vi "Text control 2 v7.2_pump-specific.vi"() -> ()   [LabVIEW 2019]
panel:
  in  "Tab Control":enum32{"Main", "Other parameters"}(tab)
  out "Vdg vs time (Bias Stress)":cluster{"Y data in":dbl[], "X data in":dbl[]}[](graph)
  out "Vp vs Vg (FPP)":cluster{"Y data in":dbl[], "X data in":dbl[]}[](graph)
  out "Vp vs time (FPP Bias Stress)":cluster{"Y data in":dbl[], "X data in":dbl[]}[](graph)
  out "Line running":i32
  out "Total lines":i32
  out "Path":path=path "C:/users/rlp38/09Apr2009LTtesting/test2.txt"
  out "I vs Vg":cluster{"Y data in":dbl[], "X data in":dbl[]}[](graph)
  out "Is max":dbl format="%.2e"
  out "Id max":dbl format="%.2e"
  out "Ig max":dbl format="%.2e"
  out "Imax vs time":cluster{"Y data in":dbl[], "X data in":dbl[]}[](graph)
  out "Imin vs time":cluster{"Y data in":dbl[], "X data in":dbl[]}[](graph)
  out "I vs Vd":cluster{"Y data in":dbl[], "X data in":dbl[]}[](graph)
  in  "Script":string="#-------------------------------------------------------\n# SPM pump cleaning script x 10\n#\n# Version: 0.5\n# Author: Dimitrios Simatos\n# Last updated: 2020-09-03\n#-------------------------------------------------------\n# Description\n#\n# This script is designed to run the cleaning sequence of the SPM OEM pump ten times.\n#-------------------------------------------------------\n# Changes\n#\n# Placed initialization and hard stop commands in the beginning.\n#-------------------------------------------------------\n# Important points\n#\n# Never leave any liquid in the pump to dry after the experiments. If they dry, the residue may block the valve.\n# Always run the cleaning cycle after the experiments.\n# Use clockwise rotation when going up in valve port numbers and vice versa.\n#-------------------------------------------------------\n# Things to do before running the script\n#\n# Remove all reservoirs, except the one in Port 3.\n# Set filenames.\n# Replace the tubing, if necessary.\n#-------------------------------------------------------\n# Port connections\n#\n# Port 1: Waste\n# Port 2: Waste\n# Port 3: Various cleaning liquids\n# Port 4: Waste\n# Port 5: Waste\n# Port 6: Waste\n#\n# Between each of the 4 runs, the settings of Port 3 will change, according to the cleaning protocol.\n# The settings for Port 3 are:\n# 1st run: 1% v/v solution of sodium hypochlorite in ultrapure water\n# 2nd run: 0.1% w/v solution of sodium dodecyl sulfate in ultrapure water\n# 3rd run: Ultrapure water\n# 4th run: Waste (in air, not immersed in liquid)\n#-------------------------------------------------------\n# Cleaning protocol for the SPM OEM pump (from the manual)\n#\n# A cleaning procedure should be performed at the end of each day or in between two different experiments.\n# An effective cleaning can be performed in the following manner:\n# • Bleach solution to kill microorganisms\n# 1. Prepare a solution of 1% chlorine bleach and deionized water\n#    NOTE: Prepare a 1% v/v solution of sodium hypochlorite in deionized water\n# 2. Prepare a reservoir and place 1 tubing in the bleach solution and 5 tubings in a waste recipient\n# 3. Pick up the bleach solution through 1 port to entirely fill the syringe\n# 4. Sequentially output the syringe content through the remaining ports and throw it to the waste\n# 5. Repeat operation at least 2 times\n# • Detergent solution to remove debris\n# 1. Prepare a solution of 0.1% detergent and deionized water\n#    NOTE: Prepare a 0.1% w/v solution of sodium dodecyl sulfate in deionized water\n# 2. Move the tubing from the bleach solution reservoir and place it into a reservoir of detergent solution\n# 3. Pick up the detergent solution through 1 port to entirely fill the syringe\n# 4. Sequentially output the detergent solution through the remaining ports into the waste recipient\n# 5. Repeat operation at least 2 times\n# • Rinsing water to prepare the pump for your next experiment\n# 1. Move the tubing from the detergent solution reservoir and place it into a reservoir of deionized water\n# 2. Pick up the rinsing solution through 1 port to entirely fill the syringe\n# 3. Sequentially output the rinse water through the remaining ports into the waste recipient\n# 4. Repeat operation at least 2 times\n# • Replace the tubing, if necessary\n#-------------------------------------------------------\n# Pumping cycles and execution time\n#\n# Execution time for a single cycle: 6 x (1 min + 10 sec) = 7 minutes\n# Total execution time: 4 x 7 = 28 minutes\n# Since the script has to run 4 times, the cleaning lasts for: 4 x 28 = 112 minutes\n# Air must be the last to be pumped through the valve, to remove all liquids.\n# There are 4 pumping cycles. Each one draws a different liquid through port 3 and pumps it sequentially through ports 1,2,4,5,6.\n# During the sequential pumping, each port receives 200 ul of liquid (20% of the total syringe volume = 600 \"plunger units\")\n# The device must be disconnected from the port during the cleaning procedure.\n# All cycles are similar, except cycle 1 has the initialization command uncommented and the first report valve command commented.\n#-------------------------------------------------------\n# Volume of liquid needed\n#\n# Volume of liquid needed per cycle: 1 ml\n# Total volume of liquid needed per script run: 4 x 1 = 4 ml\n# Since the script has to run 4 times, the first 3 with different liquids, I need:\n# 4 ml of 1% v/v solution of sodium hypochlorite in ultrapure water\n# 4 ml of 0.1% w/v solution of sodium dodecyl sulfate in ultrapure water\n# 4 ml of ultrapure water\n#-------------------------------------------------------\n# Parameters\n#\n# Syringe size: 1 ml\n# Step resolution N = 0.01 mm\n# Drawing flow V = 300 pulses/second (6000 ul/min)\n# Pumping flow V = 300 pulses/second (6000 ul/min)\n#-------------------------------------------------------\n# Pump initialization\npump /1T #hard stop pump\npump /1ZR #initialize pump\n#-------------------------------------------------------\n# Cycle 1\n# Fill the syringe\npump /1Q #query pump\npump /1? #report absolute plunger position\n#pump /1?6 #report valve position\nwait-min 1 #wait 1 minute\npump /1N0R #set step resolution: 0.01 mm\npump /1Q #query pump\npump /1? #report absolute plunger position (the plunger should be at 0)\npump /1?6 #report valve position\nwait 1000 #wait 1 second\npump /1V300R #choose speed: 300 steps/s (6000 ul/min)\npump /1Q #query pump\nwait 1000 #wait 1 second\npump /1I3R #go to port 3, clockwise rotation\npump /1Q #query pump\npump /1?6 #report valve position\nwait 1000 #wait 1 second\npump /1A3000R #go to absolute position 3000 (= draw 1 ml)\nwait 30000 #wait 30 seconds\npump /1Q #query pump\npump /1? #report absolute plunger position (the plunger should have finished moving)\n#pump /1?6 #report valve position\n# The sequential pumping begins\n# Port 1\npump /1O1R #switch to port 1, counterclockwise rotation\npump /1Q #query pump\npump /1?6 #report valve position\npump /1A2400R #go to absolute position 2400 (= pump 200 ul)\npump /1Q #query pump\npump /1? #report absolute plunger position (the plunger should be moving to 0)\nwait-min 1 #wait 1 minute\npump /1? #report absolute plunger position (the plunger should have finished moving)\n# Port 2\npump /1I2R #switch to port 2, clockwise rotation\npump /1Q #query pump\npump /1?6 #report valve position\npump /1A1800R #go to absolute position 1800 (= pump 200 ul)\npump /1Q #query pump\npump /1? #report absolute plunger position (the plunger should be moving to 0)\nwait-min 1 #wait 1 minute\npump /1? #report absolute plunger position (the plunger should have finished moving)\n# Port 4\npump /1I4R #switch to port 4, clockwise rotation\npump /1Q #query pump\npump /1?6 #report valve position\npump /1A1200R #go to absolute position 1200 (= pump 200 ul)\npump /1Q #query pump\npump /1? #report absolute plunger position (the plunger should be moving to 0)\nwait-min 1 #wait 1 minute\npump /1? #report absolute plunger position (the plunger should have finished moving)\n# Port 5\npump /1I5R #switch to port 5, clockwise rotation\npump /1Q #query pump\npump /1?6 #report valve position\npump /1A600R #go to absolute position 600 (= pump 200 ul)\npump /1Q #query pump\npump /1? #report absolute plunger position (the plunger should be moving to 0)\nwait-min 1 #wait 1 minute\npump /1? #report absolute plunger position (the plunger should have finished moving)\n# Port 6\npump /1I6R #switch to port 6, clockwise rotation\npump /1Q #query pump\npump /1?6 #report valve position\npump /1A0R #go to absolute position 0 (= pump 200 ul)\npump /1Q #query pump\npump /1? #report absolute plunger position (the plunger should be moving to 0)\nwait-min 1 #wait 1 minute\npump /1? #report absolute plunger position (the plunger should have finished moving)\n#-------------------------------------------------------\n# Cycle 2\n# Fill the syringe\n#pump /1ZR #initialize pump\npump /1Q #query pump\npump /1? #report absolute plunger position\npump /1?6 #report valve position\nwait-min 1 #wait 1 minute\npump /1N0R #set step resolution: 0.01 mm\npump /1Q #query pump\npump /1? #report absolute plunger position (the plunger should be at 0)\npump /1?6 #report valve position\nwait 1000 #wait 1 second\npump /1V300R #choose speed: 300 steps/s (6000 ul/min)\npump /1Q #query pump\nwait 1000 #wait 1 second\npump /1O3R #go to port 3, counterclockwise rotation\npump /1Q #query pump\npump /1?6 #report valve position\nwait 1000 #wait 1 second\npump /1A3000R #go to absolute position 3000 (= draw 1 ml)\nwait 30000 #wait 30 seconds\npump /1Q #query pump\npump /1? #report absolute plunger position (the plunger should have finished moving)\n#pump /1?6 #report valve position\n# The sequential pumping begins\n# Port 1\npump /1O1R #switch to port 1, counterclockwise rotation\npump /1Q #query pump\npump /1?6 #report valve position\npump /1A2400R #go to absolute position 2400 (= pump 200 ul)\npump /1Q #query pump\npump /1? #report absolute plunger position (the plunger should be moving to 0)\nwait-min 1 #wait 1 minute\npump /1? #report absolute plunger position (the plunger should have finished moving)\n# Port 2\npump /1I2R #switch to port 2, clockwise rotation\npump /1Q #query pump\npump /1?6 #report valve position\npump /1A1800R #go to absolute position 1800 (= pump 200 ul)\npump /1Q #query pump\npump /1? #report absolute plunger position (the plunger should be moving to 0)\nwait-min 1 #wait 1 minute\npump /1? #report absolute plunger position (the plunger should have finished moving)\n# Port 4\npump /1I4R #switch to port 4, clockwise rotation\npump /1Q #query pump\npump /1?6 #report valve position\npump /1A1200R #go to absolute position 1200 (= pump 200 ul)\npump /1Q #query pump\npump /1? #report absolute plunger position (the plunger should be moving to 0)\nwait-min 1 #wait 1 minute\npump /1? #report absolute plunger position (the plunger should have finished moving)\n# Port 5\npump /1I5R #switch to port 5, clockwise rotation\npump /1Q #query pump\npump /1?6 #report valve position\npump /1A600R #go to absolute position 600 (= pump 200 ul)\npump /1Q #query pump\npump /1? #report absolute plunger position (the plunger should be moving to 0)\nwait-min 1 #wait 1 minute\npump /1? #report absolute plunger position (the plunger should have finished moving)\n# Port 6\npump /1I6R #switch to port 6, clockwise rotation\npump /1Q #query pump\npump /1?6 #report valve position\npump /1A0R #go to absolute position 0 (= pump 200 ul)\npump /1Q #query pump\npump /1? #report absolute plunger position (the plunger should be moving to 0)\nwait-min 1 #wait 1 minute\npump /1? #report absolute plunger position (the plunger should have finished moving)\n#-------------------------------------------------------\n# Cycle 3\n# Fill the syringe\n#pump /1ZR #initialize pump\npump /1Q #query pump\npump /1? #report absolute plunger position\npump /1?6 #report valve position\nwait-min 1 #wait 1 minute\npump /1N0R #set step resolution: 0.01 mm\npump /1Q #query pump\npump /1? #report absolute plunger position (the plunger should be at 0)\npump /1?6 #report valve position\nwait 1000 #wait 1 second\npump /1V300R #choose speed: 300 steps/s (6000 ul/min)\npump /1Q #query pump\nwait 1000 #wait 1 second\npump /1O3R #go to port 3, counterclockwise rotation\npump /1Q #query pump\npump /1?6 #report valve position\nwait 1000 #wait 1 second\npump /1A3000R #go to absolute position 3000 (= draw 1 ml)\nwait 30000 #wait 30 seconds\npump /1Q #query pump\npump /1? #report absolute plunger position (the plunger should have finished moving)\n#pump /1?6 #report valve position\n# The sequential pumping begins\n# Port 1\npump /1O1R #switch to port 1, counterclockwise rotation\npump /1Q #query pump\npump /1?6 #report valve position\npump /1A2400R #go to absolute position 2400 (= pump 200 ul)\npump /1Q #query pump\npump /1? #report absolute plunger position (the plunger should be moving to 0)\nwait-min 1 #wait 1 minute\npump /1? #report absolute plunger position (the plunger should have finished moving)\n# Port 2\npump /1I2R #switch to port 2, clockwise rotation\npump /1Q #query pump\npump /1?6 #report valve position\npump /1A1800R #go to absolute position 1800 (= pump 200 ul)\npump /1Q #query pump\npump /1? #report absolute plunger position (the plunger should be moving to 0)\nwait-min 1 #wait 1 minute\npump /1? #report absolute plunger position (the plunger should have finished moving)\n# Port 4\npump /1I4R #switch to port 4, clockwise rotation\npump /1Q #query pump\npump /1?6 #report valve position\npump /1A1200R #go to absolute position 1200 (= pump 200 ul)\npump /1Q #query pump\npump /1? #report absolute plunger position (the plunger should be moving to 0)\nwait-min 1 #wait 1 minute\npump /1? #report absolute plunger position (the plunger should have finished moving)\n# Port 5\npump /1I5R #switch to port 5, clockwise rotation\npump /1Q #query pump\npump /1?6 #report valve position\npump /1A600R #go to absolute position 600 (= pump 200 ul)\npump /1Q #query pump\npump /1? #report absolute plunger position (the plunger should be moving to 0)\nwait-min 1 #wait 1 minute\npump /1? #report absolute plunger position (the plunger should have finished moving)\n# Port 6\npump /1I6R #switch to port 6, clockwise rotation\npump /1Q #query pump\npump /1?6 #report valve position\npump /1A0R #go to absolute position 0 (= pump 200 ul)\npump /1Q #query pump\npump /1? #report absolute plunger position (the plunger should be moving to 0)\nwait-min 1 #wait 1 minute\npump /1? #report absolute plunger position (the plunger should have finished moving)\n#-------------------------------------------------------\n# Cycle 4\n# Fill the syringe\n#pump /1ZR #initialize pump\npump /1Q #query pump\npump /1? #report absolute plunger position\npump /1?6 #report valve position\nwait-min 1 #wait 1 minute\npump /1N0R #set step resolution: 0.01 mm\npump /1Q #query pump\npump /1? #report absolute plunger position (the plunger should be at 0)\npump /1?6 #report valve position\nwait 1000 #wait 1 second\npump /1V300R #choose speed: 300 steps/s (6000 ul/min)\npump /1Q #query pump\nwait 1000 #wait 1 second\npump /1O3R #go to port 3, counterclockwise rotation\npump /1Q #query pump\npump /1?6 #report valve position\nwait 1000 #wait 1 second\npump /1A3000R #go to absolute position 3000 (= draw 1 ml)\nwait 30000 #wait 30 seconds\npump /1Q #query pump\npump /1? #report absolute plunger position (the plunger should have finished moving)\n#pump /1?6 #report valve position\n# The sequential pumping begins\n# Port 1\npump /1O1R #switch to port 1, counterclockwise rotation\npump /1Q #query pump\npump /1?6 #report valve position\npump /1A2400R #go to absolute position 2400 (= pump 200 ul)\npump /1Q #query pump\npump /1? #report absolute plunger position (the plunger should be moving to 0)\nwait-min 1 #wait 1 minute\npump /1? #report absolute plunger position (the plunger should have finished moving)\n# Port 2\npump /1I2R #switch to port 2, clockwise rotation\npump /1Q #query pump\npump /1?6 #report valve position\npump /1A1800R #go to absolute position 1800 (= pump 200 ul)\npump /1Q #query pump\npump /1? #report absolute plunger position (the plunger should be moving to 0)\nwait-min 1 #wait 1 minute\npump /1? #report absolute plunger position (the plunger should have finished moving)\n# Port 4\npump /1I4R #switch to port 4, clockwise rotation\npump /1Q #query pump\npump /1?6 #report valve position\npump /1A1200R #go to absolute position 1200 (= pump 200 ul)\npump /1Q #query pump\npump /1? #report absolute plunger position (the plunger should be moving to 0)\nwait-min 1 #wait 1 minute\npump /1? #report absolute plunger position (the plunger should have finished moving)\n# Port 5\npump /1I5R #switch to port 5, clockwise rotation\npump /1Q #query pump\npump /1?6 #report valve position\npump /1A600R #go to absolute position 600 (= pump 200 ul)\npump /1Q #query pump\npump /1? #report absolute plunger position (the plunger should be moving to 0)\nwait-min 1 #wait 1 minute\npump /1? #report absolute plunger position (the plunger should have finished moving)\n# Port 6\npump /1I6R #switch to port 6, clockwise rotation\npump /1Q #query pump\npump /1?6 #report valve position\npump /1A0R #go to absolute position 0 (= pump 200 ul)\npump /1Q #query pump\npump /1? #report absolute plunger position (the plunger should be moving to 0)\nwait-min 1 #wait 1 minute\npump /1? #report absolute plunger position (the plunger should have finished moving)\n#-------------------------------------------------------\n# Cycle 5\n# Fill the syringe\npump /1Q #query pump\npump /1? #report absolute plunger position\n#pump /1?6 #report valve position\nwait-min 1 #wait 1 minute\npump /1N0R #set step resolution: 0.01 mm\npump /1Q #query pump\npump /1? #report absolute plunger position (the plunger should be at 0)\npump /1?6 #report valve position\nwait 1000 #wait 1 second\npump /1V300R #choose speed: 300 steps/s (6000 ul/min)\npump /1Q #query pump\nwait 1000 #wait 1 second\npump /1I3R #go to port 3, clockwise rotation\npump /1Q #query pump\npump /1?6 #report valve position\nwait 1000 #wait 1 second\npump /1A3000R #go to absolute position 3000 (= draw 1 ml)\nwait 30000 #wait 30 seconds\npump /1Q #query pump\npump /1? #report absolute plunger position (the plunger should have finished moving)\n#pump /1?6 #report valve position\n# The sequential pumping begins\n# Port 1\npump /1O1R #switch to port 1, counterclockwise rotation\npump /1Q #query pump\npump /1?6 #report valve position\npump /1A2400R #go to absolute position 2400 (= pump 200 ul)\npump /1Q #query pump\npump /1? #report absolute plunger position (the plunger should be moving to 0)\nwait-min 1 #wait 1 minute\npump /1? #report absolute plunger position (the plunger should have finished moving)\n# Port 2\npump /1I2R #switch to port 2, clockwise rotation\npump /1Q #query pump\npump /1?6 #report valve position\npump /1A1800R #go to absolute position 1800 (= pump 200 ul)\npump /1Q #query pump\npump /1? #report absolute plunger position (the plunger should be moving to 0)\nwait-min 1 #wait 1 minute\npump /1? #report absolute plunger position (the plunger should have finished moving)\n# Port 4\npump /1I4R #switch to port 4, clockwise rotation\npump /1Q #query pump\npump /1?6 #report valve position\npump /1A1200R #go to absolute position 1200 (= pump 200 ul)\npump /1Q #query pump\npump /1? #report absolute plunger position (the plunger should be moving to 0)\nwait-min 1 #wait 1 minute\npump /1? #report absolute plunger position (the plunger should have finished moving)\n# Port 5\npump /1I5R #switch to port 5, clockwise rotation\npump /1Q #query pump\npump /1?6 #report valve position\npump /1A600R #go to absolute position 600 (= pump 200 ul)\npump /1Q #query pump\npump /1? #report absolute plunger position (the plunger should be moving to 0)\nwait-min 1 #wait 1 minute\npump /1? #report absolute plunger position (the plunger should have finished moving)\n# Port 6\npump /1I6R #switch to port 6, clockwise rotation\npump /1Q #query pump\npump /1?6 #report valve position\npump /1A0R #go to absolute position 0 (= pump 200 ul)\npump /1Q #query pump\npump /1? #report absolute plunger position (the plunger should be moving to 0)\nwait-min 1 #wait 1 minute\npump /1? #report absolute plunger position (the plunger should have finished moving)\n#-------------------------------------------------------\n# Cycle 6\n# Fill the syringe\n#pump /1ZR #initialize pump\npump /1Q #query pump\npump /1? #report absolute plunger position\npump /1?6 #report valve position\nwait-min 1 #wait 1 minute\npump /1N0R #set step resolution: 0.01 mm\npump /1Q #query pump\npump /1? #report absolute plunger position (the plunger should be at 0)\npump /1?6 #report valve position\nwait 1000 #wait 1 second\npump /1V300R #choose speed: 300 steps/s (6000 ul/min)\npump /1Q #query pump\nwait 1000 #wait 1 second\npump /1O3R #go to port 3, counterclockwise rotation\npump /1Q #query pump\npump /1?6 #report valve position\nwait 1000 #wait 1 second\npump /1A3000R #go to absolute position 3000 (= draw 1 ml)\nwait 30000 #wait 30 seconds\npump /1Q #query pump\npump /1? #report absolute plunger position (the plunger should have finished moving)\n#pump /1?6 #report valve position\n# The sequential pumping begins\n# Port 1\npump /1O1R #switch to port 1, counterclockwise rotation\npump /1Q #query pump\npump /1?6 #report valve position\npump /1A2400R #go to absolute position 2400 (= pump 200 ul)\npump /1Q #query pump\npump /1? #report absolute plunger position (the plunger should be moving to 0)\nwait-min 1 #wait 1 minute\npump /1? #report absolute plunger position (the plunger should have finished moving)\n# Port 2\npump /1I2R #switch to port 2, clockwise rotation\npump /1Q #query pump\npump /1?6 #report valve position\npump /1A1800R #go to absolute position 1800 (= pump 200 ul)\npump /1Q #query pump\npump /1? #report absolute plunger position (the plunger should be moving to 0)\nwait-min 1 #wait 1 minute\npump /1? #report absolute plunger position (the plunger should have finished moving)\n# Port 4\npump /1I4R #switch to port 4, clockwise rotation\npump /1Q #query pump\npump /1?6 #report valve position\npump /1A1200R #go to absolute position 1200 (= pump 200 ul)\npump /1Q #query pump\npump /1? #report absolute plunger position (the plunger should be moving to 0)\nwait-min 1 #wait 1 minute\npump /1? #report absolute plunger position (the plunger should have finished moving)\n# Port 5\npump /1I5R #switch to port 5, clockwise rotation\npump /1Q #query pump\npump /1?6 #report valve position\npump /1A600R #go to absolute position 600 (= pump 200 ul)\npump /1Q #query pump\npump /1? #report absolute plunger position (the plunger should be moving to 0)\nwait-min 1 #wait 1 minute\npump /1? #report absolute plunger position (the plunger should have finished moving)\n# Port 6\npump /1I6R #switch to port 6, clockwise rotation\npump /1Q #query pump\npump /1?6 #report valve position\npump /1A0R #go to absolute position 0 (= pump 200 ul)\npump /1Q #query pump\npump /1? #report absolute plunger position (the plunger should be moving to 0)\nwait-min 1 #wait 1 minute\npump /1? #report absolute plunger position (the plunger should have finished moving)\n#-------------------------------------------------------\n# Cycle 7\n# Fill the syringe\n#pump /1ZR #initialize pump\npump /1Q #query pump\npump /1? #report absolute plunger position\npump /1?6 #report valve position\nwait-min 1 #wait 1 minute\npump /1N0R #set step resolution: 0.01 mm\npump /1Q #query pump\npump /1? #report absolute plunger position (the plunger should be at 0)\npump /1?6 #report valve position\nwait 1000 #wait 1 second\npump /1V300R #choose speed: 300 steps/s (6000 ul/min)\npump /1Q #query pump\nwait 1000 #wait 1 second\npump /1O3R #go to port 3, counterclockwise rotation\npump /1Q #query pump\npump /1?6 #report valve position\nwait 1000 #wait 1 second\npump /1A3000R #go to absolute position 3000 (= draw 1 ml)\nwait 30000 #wait 30 seconds\npump /1Q #query pump\npump /1? #report absolute plunger position (the plunger should have finished moving)\n#pump /1?6 #report valve position\n# The sequential pumping begins\n# Port 1\npump /1O1R #switch to port 1, counterclockwise rotation\npump /1Q #query pump\npump /1?6 #report valve position\npump /1A2400R #go to absolute position 2400 (= pump 200 ul)\npump /1Q #query pump\npump /1? #report absolute plunger position (the plunger should be moving to 0)\nwait-min 1 #wait 1 minute\npump /1? #report absolute plunger position (the plunger should have finished moving)\n# Port 2\npump /1I2R #switch to port 2, clockwise rotation\npump /1Q #query pump\npump /1?6 #report valve position\npump /1A1800R #go to absolute position 1800 (= pump 200 ul)\npump /1Q #query pump\npump /1? #report absolute plunger position (the plunger should be moving to 0)\nwait-min 1 #wait 1 minute\npump /1? #report absolute plunger position (the plunger should have finished moving)\n# Port 4\npump /1I4R #switch to port 4, clockwise rotation\npump /1Q #query pump\npump /1?6 #report valve position\npump /1A1200R #go to absolute position 1200 (= pump 200 ul)\npump /1Q #query pump\npump /1? #report absolute plunger position (the plunger should be moving to 0)\nwait-min 1 #wait 1 minute\npump /1? #report absolute plunger position (the plunger should have finished moving)\n# Port 5\npump /1I5R #switch to port 5, clockwise rotation\npump /1Q #query pump\npump /1?6 #report valve position\npump /1A600R #go to absolute position 600 (= pump 200 ul)\npump /1Q #query pump\npump /1? #report absolute plunger position (the plunger should be moving to 0)\nwait-min 1 #wait 1 minute\npump /1? #report absolute plunger position (the plunger should have finished moving)\n# Port 6\npump /1I6R #switch to port 6, clockwise rotation\npump /1Q #query pump\npump /1?6 #report valve position\npump /1A0R #go to absolute position 0 (= pump 200 ul)\npump /1Q #query pump\npump /1? #report absolute plunger position (the plunger should be moving to 0)\nwait-min 1 #wait 1 minute\npump /1? #report absolute plunger position (the plunger should have finished moving)\n#-------------------------------------------------------\n# Cycle 8\n# Fill the syringe\n#pump /1ZR #initialize pump\npump /1Q #query pump\npump /1? #report absolute plunger position\npump /1?6 #report valve position\nwait-min 1 #wait 1 minute\npump /1N0R #set step resolution: 0.01 mm\npump /1Q #query pump\npump /1? #report absolute plunger position (the plunger should be at 0)\npump /1?6 #report valve position\nwait 1000 #wait 1 second\npump /1V300R #choose speed: 300 steps/s (6000 ul/min)\npump /1Q #query pump\nwait 1000 #wait 1 second\npump /1O3R #go to port 3, counterclockwise rotation\npump /1Q #query pump\npump /1?6 #report valve position\nwait 1000 #wait 1 second\npump /1A3000R #go to absolute position 3000 (= draw 1 ml)\nwait 30000 #wait 30 seconds\npump /1Q #query pump\npump /1? #report absolute plunger position (the plunger should have finished moving)\n#pump /1?6 #report valve position\n# The sequential pumping begins\n# Port 1\npump /1O1R #switch to port 1, counterclockwise rotation\npump /1Q #query pump\npump /1?6 #report valve position\npump /1A2400R #go to absolute position 2400 (= pump 200 ul)\npump /1Q #query pump\npump /1? #report absolute plunger position (the plunger should be moving to 0)\nwait-min 1 #wait 1 minute\npump /1? #report absolute plunger position (the plunger should have finished moving)\n# Port 2\npump /1I2R #switch to port 2, clockwise rotation\npump /1Q #query pump\npump /1?6 #report valve position\npump /1A1800R #go to absolute position 1800 (= pump 200 ul)\npump /1Q #query pump\npump /1? #report absolute plunger position (the plunger should be moving to 0)\nwait-min 1 #wait 1 minute\npump /1? #report absolute plunger position (the plunger should have finished moving)\n# Port 4\npump /1I4R #switch to port 4, clockwise rotation\npump /1Q #query pump\npump /1?6 #report valve position\npump /1A1200R #go to absolute position 1200 (= pump 200 ul)\npump /1Q #query pump\npump /1? #report absolute plunger position (the plunger should be moving to 0)\nwait-min 1 #wait 1 minute\npump /1? #report absolute plunger position (the plunger should have finished moving)\n# Port 5\npump /1I5R #switch to port 5, clockwise rotation\npump /1Q #query pump\npump /1?6 #report valve position\npump /1A600R #go to absolute position 600 (= pump 200 ul)\npump /1Q #query pump\npump /1? #report absolute plunger position (the plunger should be moving to 0)\nwait-min 1 #wait 1 minute\npump /1? #report absolute plunger position (the plunger should have finished moving)\n# Port 6\npump /1I6R #switch to port 6, clockwise rotation\npump /1Q #query pump\npump /1?6 #report valve position\npump /1A0R #go to absolute position 0 (= pump 200 ul)\npump /1Q #query pump\npump /1? #report absolute plunger position (the plunger should be moving to 0)\nwait-min 1 #wait 1 minute\npump /1? #report absolute plunger position (the plunger should have finished moving)\n#-------------------------------------------------------\n# Cycle 9\n# Fill the syringe\npump /1Q #query pump\npump /1? #report absolute plunger position\n#pump /1?6 #report valve position\nwait-min 1 #wait 1 minute\npump /1N0R #set step resolution: 0.01 mm\npump /1Q #query pump\npump /1? #report absolute plunger position (the plunger should be at 0)\npump /1?6 #report valve position\nwait 1000 #wait 1 second\npump /1V300R #choose speed: 300 steps/s (6000 ul/min)\npump /1Q #query pump\nwait 1000 #wait 1 second\npump /1I3R #go to port 3, clockwise rotation\npump /1Q #query pump\npump /1?6 #report valve position\nwait 1000 #wait 1 second\npump /1A3000R #go to absolute position 3000 (= draw 1 ml)\nwait 30000 #wait 30 seconds\npump /1Q #query pump\npump /1? #report absolute plunger position (the plunger should have finished moving)\n#pump /1?6 #report valve position\n# The sequential pumping begins\n# Port 1\npump /1O1R #switch to port 1, counterclockwise rotation\npump /1Q #query pump\npump /1?6 #report valve position\npump /1A2400R #go to absolute position 2400 (= pump 200 ul)\npump /1Q #query pump\npump /1? #report absolute plunger position (the plunger should be moving to 0)\nwait-min 1 #wait 1 minute\npump /1? #report absolute plunger position (the plunger should have finished moving)\n# Port 2\npump /1I2R #switch to port 2, clockwise rotation\npump /1Q #query pump\npump /1?6 #report valve position\npump /1A1800R #go to absolute position 1800 (= pump 200 ul)\npump /1Q #query pump\npump /1? #report absolute plunger position (the plunger should be moving to 0)\nwait-min 1 #wait 1 minute\npump /1? #report absolute plunger position (the plunger should have finished moving)\n# Port 4\npump /1I4R #switch to port 4, clockwise rotation\npump /1Q #query pump\npump /1?6 #report valve position\npump /1A1200R #go to absolute position 1200 (= pump 200 ul)\npump /1Q #query pump\npump /1? #report absolute plunger position (the plunger should be moving to 0)\nwait-min 1 #wait 1 minute\npump /1? #report absolute plunger position (the plunger should have finished moving)\n# Port 5\npump /1I5R #switch to port 5, clockwise rotation\npump /1Q #query pump\npump /1?6 #report valve position\npump /1A600R #go to absolute position 600 (= pump 200 ul)\npump /1Q #query pump\npump /1? #report absolute plunger position (the plunger should be moving to 0)\nwait-min 1 #wait 1 minute\npump /1? #report absolute plunger position (the plunger should have finished moving)\n# Port 6\npump /1I6R #switch to port 6, clockwise rotation\npump /1Q #query pump\npump /1?6 #report valve position\npump /1A0R #go to absolute position 0 (= pump 200 ul)\npump /1Q #query pump\npump /1? #report absolute plunger position (the plunger should be moving to 0)\nwait-min 1 #wait 1 minute\npump /1? #report absolute plunger position (the plunger should have finished moving)\n#-------------------------------------------------------\n# Cycle 10\n# Fill the syringe\n#pump /1ZR #initialize pump\npump /1Q #query pump\npump /1? #report absolute plunger position\npump /1?6 #report valve position\nwait-min 1 #wait 1 minute\npump /1N0R #set step resolution: 0.01 mm\npump /1Q #query pump\npump /1? #report absolute plunger position (the plunger should be at 0)\npump /1?6 #report valve position\nwait 1000 #wait 1 second\npump /1V300R #choose speed: 300 steps/s (6000 ul/min)\npump /1Q #query pump\nwait 1000 #wait 1 second\npump /1O3R #go to port 3, counterclockwise rotation\npump /1Q #query pump\npump /1?6 #report valve position\nwait 1000 #wait 1 second\npump /1A3000R #go to absolute position 3000 (= draw 1 ml)\nwait 30000 #wait 30 seconds\npump /1Q #query pump\npump /1? #report absolute plunger position (the plunger should have finished moving)\n#pump /1?6 #report valve position\n# The sequential pumping begins\n# Port 1\npump /1O1R #switch to port 1, counterclockwise rotation\npump /1Q #query pump\npump /1?6 #report valve position\npump /1A2400R #go to absolute position 2400 (= pump 200 ul)\npump /1Q #query pump\npump /1? #report absolute plunger position (the plunger should be moving to 0)\nwait-min 1 #wait 1 minute\npump /1? #report absolute plunger position (the plunger should have finished moving)\n# Port 2\npump /1I2R #switch to port 2, clockwise rotation\npump /1Q #query pump\npump /1?6 #report valve position\npump /1A1800R #go to absolute position 1800 (= pump 200 ul)\npump /1Q #query pump\npump /1? #report absolute plunger position (the plunger should be moving to 0)\nwait-min 1 #wait 1 minute\npump /1? #report absolute plunger position (the plunger should have finished moving)\n# Port 4\npump /1I4R #switch to port 4, clockwise rotation\npump /1Q #query pump\npump /1?6 #report valve position\npump /1A1200R #go to absolute position 1200 (= pump 200 ul)\npump /1Q #query pump\npump /1? #report absolute plunger position (the plunger should be moving to 0)\nwait-min 1 #wait 1 minute\npump /1? #report absolute plunger position (the plunger should have finished moving)\n# Port 5\npump /1I5R #switch to port 5, clockwise rotation\npump /1Q #query pump\npump /1?6 #report valve position\npump /1A600R #go to absolute position 600 (= pump 200 ul)\npump /1Q #query pump\npump /1? #report absolute plunger position (the plunger should be moving to 0)\nwait-min 1 #wait 1 minute\npump /1? #report absolute plunger position (the plunger should have finished moving)\n# Port 6\npump /1I6R #switch to port 6, clockwise rotation\npump /1Q #query pump\npump /1?6 #report valve position\npump /1A0R #go to absolute position 0 (= pump 200 ul)\npump /1Q #query pump\npump /1? #report absolute plunger position (the plunger should be moving to 0)\nwait-min 1 #wait 1 minute\npump /1? #report absolute plunger position (the plunger should have finished moving)\n#-------------------------------------------------------\n# Cycle 11\n# Fill the syringe\n#pump /1ZR #initialize pump\npump /1Q #query pump\npump /1? #report absolute plunger position\npump /1?6 #report valve position\nwait-min 1 #wait 1 minute\npump /1N0R #set step resolution: 0.01 mm\npump /1Q #query pump\npump /1? #report absolute plunger position (the plunger should be at 0)\npump /1?6 #report valve position\nwait 1000 #wait 1 second\npump /1V300R #choose speed: 300 steps/s (6000 ul/min)\npump /1Q #query pump\nwait 1000 #wait 1 second\npump /1O3R #go to port 3, counterclockwise rotation\npump /1Q #query pump\npump /1?6 #report valve position\nwait 1000 #wait 1 second\npump /1A3000R #go to absolute position 3000 (= draw 1 ml)\nwait 30000 #wait 30 seconds\npump /1Q #query pump\npump /1? #report absolute plunger position (the plunger should have finished moving)\n#pump /1?6 #report valve position\n# The sequential pumping begins\n# Port 1\npump /1O1R #switch to port 1, counterclockwise rotation\npump /1Q #query pump\npump /1?6 #report valve position\npump /1A2400R #go to absolute position 2400 (= pump 200 ul)\npump /1Q #query pump\npump /1? #report absolute plunger position (the plunger should be moving to 0)\nwait-min 1 #wait 1 minute\npump /1? #report absolute plunger position (the plunger should have finished moving)\n# Port 2\npump /1I2R #switch to port 2, clockwise rotation\npump /1Q #query pump\npump /1?6 #report valve position\npump /1A1800R #go to absolute position 1800 (= pump 200 ul)\npump /1Q #query pump\npump /1? #report absolute plunger position (the plunger should be moving to 0)\nwait-min 1 #wait 1 minute\npump /1? #report absolute plunger position (the plunger should have finished moving)\n# Port 4\npump /1I4R #switch to port 4, clockwise rotation\npump /1Q #query pump\npump /1?6 #report valve position\npump /1A1200R #go to absolute position 1200 (= pump 200 ul)\npump /1Q #query pump\npump /1? #report absolute plunger position (the plunger should be moving to 0)\nwait-min 1 #wait 1 minute\npump /1? #report absolute plunger position (the plunger should have finished moving)\n# Port 5\npump /1I5R #switch to port 5, clockwise rotation\npump /1Q #query pump\npump /1?6 #report valve position\npump /1A600R #go to absolute position 600 (= pump 200 ul)\npump /1Q #query pump\npump /1? #report absolute plunger position (the plunger should be moving to 0)\nwait-min 1 #wait 1 minute\npump /1? #report absolute plunger position (the plunger should have finished moving)\n# Port 6\npump /1I6R #switch to port 6, clockwise rotation\npump /1Q #query pump\npump /1?6 #report valve position\npump /1A0R #go to absolute position 0 (= pump 200 ul)\npump /1Q #query pump\npump /1? #report absolute plunger position (the plunger should be moving to 0)\nwait-min 1 #wait 1 minute\npump /1? #report absolute plunger position (the plunger should have finished moving)\n#-------------------------------------------------------\n# Cycle 12\n# Fill the syringe\n#pump /1ZR #initialize pump\npump /1Q #query pump\npump /1? #report absolute plunger position\npump /1?6 #report valve position\nwait-min 1 #wait 1 minute\npump /1N0R #set step resolution: 0.01 mm\npump /1Q #query pump\npump /1? #report absolute plunger position (the plunger should be at 0)\npump /1?6 #report valve position\nwait 1000 #wait 1 second\npump /1V300R #choose speed: 300 steps/s (6000 ul/min)\npump /1Q #query pump\nwait 1000 #wait 1 second\npump /1O3R #go to port 3, counterclockwise rotation\npump /1Q #query pump\npump /1?6 #report valve position\nwait 1000 #wait 1 second\npump /1A3000R #go to absolute position 3000 (= draw 1 ml)\nwait 30000 #wait 30 seconds\npump /1Q #query pump\npump /1? #report absolute plunger position (the plunger should have finished moving)\n#pump /1?6 #report valve position\n# The sequential pumping begins\n# Port 1\npump /1O1R #switch to port 1, counterclockwise rotation\npump /1Q #query pump\npump /1?6 #report valve position\npump /1A2400R #go to absolute position 2400 (= pump 200 ul)\npump /1Q #query pump\npump /1? #report absolute plunger position (the plunger should be moving to 0)\nwait-min 1 #wait 1 minute\npump /1? #report absolute plunger position (the plunger should have finished moving)\n# Port 2\npump /1I2R #switch to port 2, clockwise rotation\npump /1Q #query pump\npump /1?6 #report valve position\npump /1A1800R #go to absolute position 1800 (= pump 200 ul)\npump /1Q #query pump\npump /1? #report absolute plunger position (the plunger should be moving to 0)\nwait-min 1 #wait 1 minute\npump /1? #report absolute plunger position (the plunger should have finished moving)\n# Port 4\npump /1I4R #switch to port 4, clockwise rotation\npump /1Q #query pump\npump /1?6 #report valve position\npump /1A1200R #go to absolute position 1200 (= pump 200 ul)\npump /1Q #query pump\npump /1? #report absolute plunger position (the plunger should be moving to 0)\nwait-min 1 #wait 1 minute\npump /1? #report absolute plunger position (the plunger should have finished moving)\n# Port 5\npump /1I5R #switch to port 5, clockwise rotation\npump /1Q #query pump\npump /1?6 #report valve position\npump /1A600R #go to absolute position 600 (= pump 200 ul)\npump /1Q #query pump\npump /1? #report absolute plunger position (the plunger should be moving to 0)\nwait-min 1 #wait 1 minute\npump /1? #report absolute plunger position (the plunger should have finished moving)\n# Port 6\npump /1I6R #switch to port 6, clockwise rotation\npump /1Q #query pump\npump /1?6 #report valve position\npump /1A0R #go to absolute position 0 (= pump 200 ul)\npump /1Q #query pump\npump /1? #report absolute plunger position (the plunger should be moving to 0)\nwait-min 1 #wait 1 minute\npump /1? #report absolute plunger position (the plunger should have finished moving)\n#-------------------------------------------------------\n# Cycle 13\n# Fill the syringe\npump /1Q #query pump\npump /1? #report absolute plunger position\n#pump /1?6 #report valve position\nwait-min 1 #wait 1 minute\npump /1N0R #set step resolution: 0.01 mm\npump /1Q #query pump\npump /1? #report absolute plunger position (the plunger should be at 0)\npump /1?6 #report valve position\nwait 1000 #wait 1 second\npump /1V300R #choose speed: 300 steps/s (6000 ul/min)\npump /1Q #query pump\nwait 1000 #wait 1 second\npump /1I3R #go to port 3, clockwise rotation\npump /1Q #query pump\npump /1?6 #report valve position\nwait 1000 #wait 1 second\npump /1A3000R #go to absolute position 3000 (= draw 1 ml)\nwait 30000 #wait 30 seconds\npump /1Q #query pump\npump /1? #report absolute plunger position (the plunger should have finished moving)\n#pump /1?6 #report valve position\n# The sequential pumping begins\n# Port 1\npump /1O1R #switch to port 1, counterclockwise rotation\npump /1Q #query pump\npump /1?6 #report valve position\npump /1A2400R #go to absolute position 2400 (= pump 200 ul)\npump /1Q #query pump\npump /1? #report absolute plunger position (the plunger should be moving to 0)\nwait-min 1 #wait 1 minute\npump /1? #report absolute plunger position (the plunger should have finished moving)\n# Port 2\npump /1I2R #switch to port 2, clockwise rotation\npump /1Q #query pump\npump /1?6 #report valve position\npump /1A1800R #go to absolute position 1800 (= pump 200 ul)\npump /1Q #query pump\npump /1? #report absolute plunger position (the plunger should be moving to 0)\nwait-min 1 #wait 1 minute\npump /1? #report absolute plunger position (the plunger should have finished moving)\n# Port 4\npump /1I4R #switch to port 4, clockwise rotation\npump /1Q #query pump\npump /1?6 #report valve position\npump /1A1200R #go to absolute position 1200 (= pump 200 ul)\npump /1Q #query pump\npump /1? #report absolute plunger position (the plunger should be moving to 0)\nwait-min 1 #wait 1 minute\npump /1? #report absolute plunger position (the plunger should have finished moving)\n# Port 5\npump /1I5R #switch to port 5, clockwise rotation\npump /1Q #query pump\npump /1?6 #report valve position\npump /1A600R #go to absolute position 600 (= pump 200 ul)\npump /1Q #query pump\npump /1? #report absolute plunger position (the plunger should be moving to 0)\nwait-min 1 #wait 1 minute\npump /1? #report absolute plunger position (the plunger should have finished moving)\n# Port 6\npump /1I6R #switch to port 6, clockwise rotation\npump /1Q #query pump\npump /1?6 #report valve position\npump /1A0R #go to absolute position 0 (= pump 200 ul)\npump /1Q #query pump\npump /1? #report absolute plunger position (the plunger should be moving to 0)\nwait-min 1 #wait 1 minute\npump /1? #report absolute plunger position (the plunger should have finished moving)\n#-------------------------------------------------------\n# Cycle 14\n# Fill the syringe\n#pump /1ZR #initialize pump\npump /1Q #query pump\npump /1? #report absolute plunger position\npump /1?6 #report valve position\nwait-min 1 #wait 1 minute\npump /1N0R #set step resolution: 0.01 mm\npump /1Q #query pump\npump /1? #report absolute plunger position (the plunger should be at 0)\npump /1?6 #report valve position\nwait 1000 #wait 1 second\npump /1V300R #choose speed: 300 steps/s (6000 ul/min)\npump /1Q #query pump\nwait 1000 #wait 1 second\npump /1O3R #go to port 3, counterclockwise rotation\npump /1Q #query pump\npump /1?6 #report valve position\nwait 1000 #wait 1 second\npump /1A3000R #go to absolute position 3000 (= draw 1 ml)\nwait 30000 #wait 30 seconds\npump /1Q #query pump\npump /1? #report absolute plunger position (the plunger should have finished moving)\n#pump /1?6 #report valve position\n# The sequential pumping begins\n# Port 1\npump /1O1R #switch to port 1, counterclockwise rotation\npump /1Q #query pump\npump /1?6 #report valve position\npump /1A2400R #go to absolute position 2400 (= pump 200 ul)\npump /1Q #query pump\npump /1? #report absolute plunger position (the plunger should be moving to 0)\nwait-min 1 #wait 1 minute\npump /1? #report absolute plunger position (the plunger should have finished moving)\n# Port 2\npump /1I2R #switch to port 2, clockwise rotation\npump /1Q #query pump\npump /1?6 #report valve position\npump /1A1800R #go to absolute position 1800 (= pump 200 ul)\npump /1Q #query pump\npump /1? #report absolute plunger position (the plunger should be moving to 0)\nwait-min 1 #wait 1 minute\npump /1? #report absolute plunger position (the plunger should have finished moving)\n# Port 4\npump /1I4R #switch to port 4, clockwise rotation\npump /1Q #query pump\npump /1?6 #report valve position\npump /1A1200R #go to absolute position 1200 (= pump 200 ul)\npump /1Q #query pump\npump /1? #report absolute plunger position (the plunger should be moving to 0)\nwait-min 1 #wait 1 minute\npump /1? #report absolute plunger position (the plunger should have finished moving)\n# Port 5\npump /1I5R #switch to port 5, clockwise rotation\npump /1Q #query pump\npump /1?6 #report valve position\npump /1A600R #go to absolute position 600 (= pump 200 ul)\npump /1Q #query pump\npump /1? #report absolute plunger position (the plunger should be moving to 0)\nwait-min 1 #wait 1 minute\npump /1? #report absolute plunger position (the plunger should have finished moving)\n# Port 6\npump /1I6R #switch to port 6, clockwise rotation\npump /1Q #query pump\npump /1?6 #report valve position\npump /1A0R #go to absolute position 0 (= pump 200 ul)\npump /1Q #query pump\npump /1? #report absolute plunger position (the plunger should be moving to 0)\nwait-min 1 #wait 1 minute\npump /1? #report absolute plunger position (the plunger should have finished moving)\n#-------------------------------------------------------\n# Cycle 15\n# Fill the syringe\n#pump /1ZR #initialize pump\npump /1Q #query pump\npump /1? #report absolute plunger position\npump /1?6 #report valve position\nwait-min 1 #wait 1 minute\npump /1N0R #set step resolution: 0.01 mm\npump /1Q #query pump\npump /1? #report absolute plunger position (the plunger should be at 0)\npump /1?6 #report valve position\nwait 1000 #wait 1 second\npump /1V300R #choose speed: 300 steps/s (6000 ul/min)\npump /1Q #query pump\nwait 1000 #wait 1 second\npump /1O3R #go to port 3, counterclockwise rotation\npump /1Q #query pump\npump /1?6 #report valve position\nwait 1000 #wait 1 second\npump /1A3000R #go to absolute position 3000 (= draw 1 ml)\nwait 30000 #wait 30 seconds\npump /1Q #query pump\npump /1? #report absolute plunger position (the plunger should have finished moving)\n#pump /1?6 #report valve position\n# The sequential pumping begins\n# Port 1\npump /1O1R #switch to port 1, counterclockwise rotation\npump /1Q #query pump\npump /1?6 #report valve position\npump /1A2400R #go to absolute position 2400 (= pump 200 ul)\npump /1Q #query pump\npump /1? #report absolute plunger position (the plunger should be moving to 0)\nwait-min 1 #wait 1 minute\npump /1? #report absolute plunger position (the plunger should have finished moving)\n# Port 2\npump /1I2R #switch to port 2, clockwise rotation\npump /1Q #query pump\npump /1?6 #report valve position\npump /1A1800R #go to absolute position 1800 (= pump 200 ul)\npump /1Q #query pump\npump /1? #report absolute plunger position (the plunger should be moving to 0)\nwait-min 1 #wait 1 minute\npump /1? #report absolute plunger position (the plunger should have finished moving)\n# Port 4\npump /1I4R #switch to port 4, clockwise rotation\npump /1Q #query pump\npump /1?6 #report valve position\npump /1A1200R #go to absolute position 1200 (= pump 200 ul)\npump /1Q #query pump\npump /1? #report absolute plunger position (the plunger should be moving to 0)\nwait-min 1 #wait 1 minute\npump /1? #report absolute plunger position (the plunger should have finished moving)\n# Port 5\npump /1I5R #switch to port 5, clockwise rotation\npump /1Q #query pump\npump /1?6 #report valve position\npump /1A600R #go to absolute position 600 (= pump 200 ul)\npump /1Q #query pump\npump /1? #report absolute plunger position (the plunger should be moving to 0)\nwait-min 1 #wait 1 minute\npump /1? #report absolute plunger position (the plunger should have finished moving)\n# Port 6\npump /1I6R #switch to port 6, clockwise rotation\npump /1Q #query pump\npump /1?6 #report valve position\npump /1A0R #go to absolute position 0 (= pump 200 ul)\npump /1Q #query pump\npump /1? #report absolute plunger position (the plunger should be moving to 0)\nwait-min 1 #wait 1 minute\npump /1? #report absolute plunger position (the plunger should have finished moving)\n#-------------------------------------------------------\n# Cycle 16\n# Fill the syringe\n#pump /1ZR #initialize pump\npump /1Q #query pump\npump /1? #report absolute plunger position\npump /1?6 #report valve position\nwait-min 1 #wait 1 minute\npump /1N0R #set step resolution: 0.01 mm\npump /1Q #query pump\npump /1? #report absolute plunger position (the plunger should be at 0)\npump /1?6 #report valve position\nwait 1000 #wait 1 second\npump /1V300R #choose speed: 300 steps/s (6000 ul/min)\npump /1Q #query pump\nwait 1000 #wait 1 second\npump /1O3R #go to port 3, counterclockwise rotation\npump /1Q #query pump\npump /1?6 #report valve position\nwait 1000 #wait 1 second\npump /1A3000R #go to absolute position 3000 (= draw 1 ml)\nwait 30000 #wait 30 seconds\npump /1Q #query pump\npump /1? #report absolute plunger position (the plunger should have finished moving)\n#pump /1?6 #report valve position\n# The sequential pumping begins\n# Port 1\npump /1O1R #switch to port 1, counterclockwise rotation\npump /1Q #query pump\npump /1?6 #report valve position\npump /1A2400R #go to absolute position 2400 (= pump 200 ul)\npump /1Q #query pump\npump /1? #report absolute plunger position (the plunger should be moving to 0)\nwait-min 1 #wait 1 minute\npump /1? #report absolute plunger position (the plunger should have finished moving)\n# Port 2\npump /1I2R #switch to port 2, clockwise rotation\npump /1Q #query pump\npump /1?6 #report valve position\npump /1A1800R #go to absolute position 1800 (= pump 200 ul)\npump /1Q #query pump\npump /1? #report absolute plunger position (the plunger should be moving to 0)\nwait-min 1 #wait 1 minute\npump /1? #report absolute plunger position (the plunger should have finished moving)\n# Port 4\npump /1I4R #switch to port 4, clockwise rotation\npump /1Q #query pump\npump /1?6 #report valve position\npump /1A1200R #go to absolute position 1200 (= pump 200 ul)\npump /1Q #query pump\npump /1? #report absolute plunger position (the plunger should be moving to 0)\nwait-min 1 #wait 1 minute\npump /1? #report absolute plunger position (the plunger should have finished moving)\n# Port 5\npump /1I5R #switch to port 5, clockwise rotation\npump /1Q #query pump\npump /1?6 #report valve position\npump /1A600R #go to absolute position 600 (= pump 200 ul)\npump /1Q #query pump\npump /1? #report absolute plunger position (the plunger should be moving to 0)\nwait-min 1 #wait 1 minute\npump /1? #report absolute plunger position (the plunger should have finished moving)\n# Port 6\npump /1I6R #switch to port 6, clockwise rotation\npump /1Q #query pump\npump /1?6 #report valve position\npump /1A0R #go to absolute position 0 (= pump 200 ul)\npump /1Q #query pump\npump /1? #report absolute plunger position (the plunger should be moving to 0)\nwait-min 1 #wait 1 minute\npump /1? #report absolute plunger position (the plunger should have finished moving)\n#-------------------------------------------------------\n# Cycle 17\n# Fill the syringe\npump /1Q #query pump\npump /1? #report absolute plunger position\n#pump /1?6 #report valve position\nwait-min 1 #wait 1 minute\npump /1N0R #set step resolution: 0.01 mm\npump /1Q #query pump\npump /1? #report absolute plunger position (the plunger should be at 0)\npump /1?6 #report valve position\nwait 1000 #wait 1 second\npump /1V300R #choose speed: 300 steps/s (6000 ul/min)\npump /1Q #query pump\nwait 1000 #wait 1 second\npump /1I3R #go to port 3, clockwise rotation\npump /1Q #query pump\npump /1?6 #report valve position\nwait 1000 #wait 1 second\npump /1A3000R #go to absolute position 3000 (= draw 1 ml)\nwait 30000 #wait 30 seconds\npump /1Q #query pump\npump /1? #report absolute plunger position (the plunger should have finished moving)\n#pump /1?6 #report valve position\n# The sequential pumping begins\n# Port 1\npump /1O1R #switch to port 1, counterclockwise rotation\npump /1Q #query pump\npump /1?6 #report valve position\npump /1A2400R #go to absolute position 2400 (= pump 200 ul)\npump /1Q #query pump\npump /1? #report absolute plunger position (the plunger should be moving to 0)\nwait-min 1 #wait 1 minute\npump /1? #report absolute plunger position (the plunger should have finished moving)\n# Port 2\npump /1I2R #switch to port 2, clockwise rotation\npump /1Q #query pump\npump /1?6 #report valve position\npump /1A1800R #go to absolute position 1800 (= pump 200 ul)\npump /1Q #query pump\npump /1? #report absolute plunger position (the plunger should be moving to 0)\nwait-min 1 #wait 1 minute\npump /1? #report absolute plunger position (the plunger should have finished moving)\n# Port 4\npump /1I4R #switch to port 4, clockwise rotation\npump /1Q #query pump\npump /1?6 #report valve position\npump /1A1200R #go to absolute position 1200 (= pump 200 ul)\npump /1Q #query pump\npump /1? #report absolute plunger position (the plunger should be moving to 0)\nwait-min 1 #wait 1 minute\npump /1? #report absolute plunger position (the plunger should have finished moving)\n# Port 5\npump /1I5R #switch to port 5, clockwise rotation\npump /1Q #query pump\npump /1?6 #report valve position\npump /1A600R #go to absolute position 600 (= pump 200 ul)\npump /1Q #query pump\npump /1? #report absolute plunger position (the plunger should be moving to 0)\nwait-min 1 #wait 1 minute\npump /1? #report absolute plunger position (the plunger should have finished moving)\n# Port 6\npump /1I6R #switch to port 6, clockwise rotation\npump /1Q #query pump\npump /1?6 #report valve position\npump /1A0R #go to absolute position 0 (= pump 200 ul)\npump /1Q #query pump\npump /1? #report absolute plunger position (the plunger should be moving to 0)\nwait-min 1 #wait 1 minute\npump /1? #report absolute plunger position (the plunger should have finished moving)\n#-------------------------------------------------------\n# Cycle 18\n# Fill the syringe\n#pump /1ZR #initialize pump\npump /1Q #query pump\npump /1? #report absolute plunger position\npump /1?6 #report valve position\nwait-min 1 #wait 1 minute\npump /1N0R #set step resolution: 0.01 mm\npump /1Q #query pump\npump /1? #report absolute plunger position (the plunger should be at 0)\npump /1?6 #report valve position\nwait 1000 #wait 1 second\npump /1V300R #choose speed: 300 steps/s (6000 ul/min)\npump /1Q #query pump\nwait 1000 #wait 1 second\npump /1O3R #go to port 3, counterclockwise rotation\npump /1Q #query pump\npump /1?6 #report valve position\nwait 1000 #wait 1 second\npump /1A3000R #go to absolute position 3000 (= draw 1 ml)\nwait 30000 #wait 30 seconds\npump /1Q #query pump\npump /1? #report absolute plunger position (the plunger should have finished moving)\n#pump /1?6 #report valve position\n# The sequential pumping begins\n# Port 1\npump /1O1R #switch to port 1, counterclockwise rotation\npump /1Q #query pump\npump /1?6 #report valve position\npump /1A2400R #go to absolute position 2400 (= pump 200 ul)\npump /1Q #query pump\npump /1? #report absolute plunger position (the plunger should be moving to 0)\nwait-min 1 #wait 1 minute\npump /1? #report absolute plunger position (the plunger should have finished moving)\n# Port 2\npump /1I2R #switch to port 2, clockwise rotation\npump /1Q #query pump\npump /1?6 #report valve position\npump /1A1800R #go to absolute position 1800 (= pump 200 ul)\npump /1Q #query pump\npump /1? #report absolute plunger position (the plunger should be moving to 0)\nwait-min 1 #wait 1 minute\npump /1? #report absolute plunger position (the plunger should have finished moving)\n# Port 4\npump /1I4R #switch to port 4, clockwise rotation\npump /1Q #query pump\npump /1?6 #report valve position\npump /1A1200R #go to absolute position 1200 (= pump 200 ul)\npump /1Q #query pump\npump /1? #report absolute plunger position (the plunger should be moving to 0)\nwait-min 1 #wait 1 minute\npump /1? #report absolute plunger position (the plunger should have finished moving)\n# Port 5\npump /1I5R #switch to port 5, clockwise rotation\npump /1Q #query pump\npump /1?6 #report valve position\npump /1A600R #go to absolute position 600 (= pump 200 ul)\npump /1Q #query pump\npump /1? #report absolute plunger position (the plunger should be moving to 0)\nwait-min 1 #wait 1 minute\npump /1? #report absolute plunger position (the plunger should have finished moving)\n# Port 6\npump /1I6R #switch to port 6, clockwise rotation\npump /1Q #query pump\npump /1?6 #report valve position\npump /1A0R #go to absolute position 0 (= pump 200 ul)\npump /1Q #query pump\npump /1? #report absolute plunger position (the plunger should be moving to 0)\nwait-min 1 #wait 1 minute\npump /1? #report absolute plunger position (the plunger should have finished moving)\n#-------------------------------------------------------\n# Cycle 19\n# Fill the syringe\n#pump /1ZR #initialize pump\npump /1Q #query pump\npump /1? #report absolute plunger position\npump /1?6 #report valve position\nwait-min 1 #wait 1 minute\npump /1N0R #set step resolution: 0.01 mm\npump /1Q #query pump\npump /1? #report absolute plunger position (the plunger should be at 0)\npump /1?6 #report valve position\nwait 1000 #wait 1 second\npump /1V300R #choose speed: 300 steps/s (6000 ul/min)\npump /1Q #query pump\nwait 1000 #wait 1 second\npump /1O3R #go to port 3, counterclockwise rotation\npump /1Q #query pump\npump /1?6 #report valve position\nwait 1000 #wait 1 second\npump /1A3000R #go to absolute position 3000 (= draw 1 ml)\nwait 30000 #wait 30 seconds\npump /1Q #query pump\npump /1? #report absolute plunger position (the plunger should have finished moving)\n#pump /1?6 #report valve position\n# The sequential pumping begins\n# Port 1\npump /1O1R #switch to port 1, counterclockwise rotation\npump /1Q #query pump\npump /1?6 #report valve position\npump /1A2400R #go to absolute position 2400 (= pump 200 ul)\npump /1Q #query pump\npump /1? #report absolute plunger position (the plunger should be moving to 0)\nwait-min 1 #wait 1 minute\npump /1? #report absolute plunger position (the plunger should have finished moving)\n# Port 2\npump /1I2R #switch to port 2, clockwise rotation\npump /1Q #query pump\npump /1?6 #report valve position\npump /1A1800R #go to absolute position 1800 (= pump 200 ul)\npump /1Q #query pump\npump /1? #report absolute plunger position (the plunger should be moving to 0)\nwait-min 1 #wait 1 minute\npump /1? #report absolute plunger position (the plunger should have finished moving)\n# Port 4\npump /1I4R #switch to port 4, clockwise rotation\npump /1Q #query pump\npump /1?6 #report valve position\npump /1A1200R #go to absolute position 1200 (= pump 200 ul)\npump /1Q #query pump\npump /1? #report absolute plunger position (the plunger should be moving to 0)\nwait-min 1 #wait 1 minute\npump /1? #report absolute plunger position (the plunger should have finished moving)\n# Port 5\npump /1I5R #switch to port 5, clockwise rotation\npump /1Q #query pump\npump /1?6 #report valve position\npump /1A600R #go to absolute position 600 (= pump 200 ul)\npump /1Q #query pump\npump /1? #report absolute plunger position (the plunger should be moving to 0)\nwait-min 1 #wait 1 minute\npump /1? #report absolute plunger position (the plunger should have finished moving)\n# Port 6\npump /1I6R #switch to port 6, clockwise rotation\npump /1Q #query pump\npump /1?6 #report valve position\npump /1A0R #go to absolute position 0 (= pump 200 ul)\npump /1Q #query pump\npump /1? #report absolute plunger position (the plunger should be moving to 0)\nwait-min 1 #wait 1 minute\npump /1? #report absolute plunger position (the plunger should have finished moving)\n#-------------------------------------------------------\n# Cycle 20\n# Fill the syringe\n#pump /1ZR #initialize pump\npump /1Q #query pump\npump /1? #report absolute plunger position\npump /1?6 #report valve position\nwait-min 1 #wait 1 minute\npump /1N0R #set step resolution: 0.01 mm\npump /1Q #query pump\npump /1? #report absolute plunger position (the plunger should be at 0)\npump /1?6 #report valve position\nwait 1000 #wait 1 second\npump /1V300R #choose speed: 300 steps/s (6000 ul/min)\npump /1Q #query pump\nwait 1000 #wait 1 second\npump /1O3R #go to port 3, counterclockwise rotation\npump /1Q #query pump\npump /1?6 #report valve position\nwait 1000 #wait 1 second\npump /1A3000R #go to absolute position 3000 (= draw 1 ml)\nwait 30000 #wait 30 seconds\npump /1Q #query pump\npump /1? #report absolute plunger position (the plunger should have finished moving)\n#pump /1?6 #report valve position\n# The sequential pumping begins\n# Port 1\npump /1O1R #switch to port 1, counterclockwise rotation\npump /1Q #query pump\npump /1?6 #report valve position\npump /1A2400R #go to absolute position 2400 (= pump 200 ul)\npump /1Q #query pump\npump /1? #report absolute plunger position (the plunger should be moving to 0)\nwait-min 1 #wait 1 minute\npump /1? #report absolute plunger position (the plunger should have finished moving)\n# Port 2\npump /1I2R #switch to port 2, clockwise rotation\npump /1Q #query pump\npump /1?6 #report valve position\npump /1A1800R #go to absolute position 1800 (= pump 200 ul)\npump /1Q #query pump\npump /1? #report absolute plunger position (the plunger should be moving to 0)\nwait-min 1 #wait 1 minute\npump /1? #report absolute plunger position (the plunger should have finished moving)\n# Port 4\npump /1I4R #switch to port 4, clockwise rotation\npump /1Q #query pump\npump /1?6 #report valve position\npump /1A1200R #go to absolute position 1200 (= pump 200 ul)\npump /1Q #query pump\npump /1? #report absolute plunger position (the plunger should be moving to 0)\nwait-min 1 #wait 1 minute\npump /1? #report absolute plunger position (the plunger should have finished moving)\n# Port 5\npump /1I5R #switch to port 5, clockwise rotation\npump /1Q #query pump\npump /1?6 #report valve position\npump /1A600R #go to absolute position 600 (= pump 200 ul)\npump /1Q #query pump\npump /1? #report absolute plunger position (the plunger should be moving to 0)\nwait-min 1 #wait 1 minute\npump /1? #report absolute plunger position (the plunger should have finished moving)\n# Port 6\npump /1I6R #switch to port 6, clockwise rotation\npump /1Q #query pump\npump /1?6 #report valve position\npump /1A0R #go to absolute position 0 (= pump 200 ul)\npump /1Q #query pump\npump /1? #report absolute plunger position (the plunger should be moving to 0)\nwait-min 1 #wait 1 minute\npump /1? #report absolute plunger position (the plunger should have finished moving)\n#-------------------------------------------------------\n# Cycle 21\n# Fill the syringe\npump /1Q #query pump\npump /1? #report absolute plunger position\n#pump /1?6 #report valve position\nwait-min 1 #wait 1 minute\npump /1N0R #set step resolution: 0.01 mm\npump /1Q #query pump\npump /1? #report absolute plunger position (the plunger should be at 0)\npump /1?6 #report valve position\nwait 1000 #wait 1 second\npump /1V300R #choose speed: 300 steps/s (6000 ul/min)\npump /1Q #query pump\nwait 1000 #wait 1 second\npump /1I3R #go to port 3, clockwise rotation\npump /1Q #query pump\npump /1?6 #report valve position\nwait 1000 #wait 1 second\npump /1A3000R #go to absolute position 3000 (= draw 1 ml)\nwait 30000 #wait 30 seconds\npump /1Q #query pump\npump /1? #report absolute plunger position (the plunger should have finished moving)\n#pump /1?6 #report valve position\n# The sequential pumping begins\n# Port 1\npump /1O1R #switch to port 1, counterclockwise rotation\npump /1Q #query pump\npump /1?6 #report valve position\npump /1A2400R #go to absolute position 2400 (= pump 200 ul)\npump /1Q #query pump\npump /1? #report absolute plunger position (the plunger should be moving to 0)\nwait-min 1 #wait 1 minute\npump /1? #report absolute plunger position (the plunger should have finished moving)\n# Port 2\npump /1I2R #switch to port 2, clockwise rotation\npump /1Q #query pump\npump /1?6 #report valve position\npump /1A1800R #go to absolute position 1800 (= pump 200 ul)\npump /1Q #query pump\npump /1? #report absolute plunger position (the plunger should be moving to 0)\nwait-min 1 #wait 1 minute\npump /1? #report absolute plunger position (the plunger should have finished moving)\n# Port 4\npump /1I4R #switch to port 4, clockwise rotation\npump /1Q #query pump\npump /1?6 #report valve position\npump /1A1200R #go to absolute position 1200 (= pump 200 ul)\npump /1Q #query pump\npump /1? #report absolute plunger position (the plunger should be moving to 0)\nwait-min 1 #wait 1 minute\npump /1? #report absolute plunger position (the plunger should have finished moving)\n# Port 5\npump /1I5R #switch to port 5, clockwise rotation\npump /1Q #query pump\npump /1?6 #report valve position\npump /1A600R #go to absolute position 600 (= pump 200 ul)\npump /1Q #query pump\npump /1? #report absolute plunger position (the plunger should be moving to 0)\nwait-min 1 #wait 1 minute\npump /1? #report absolute plunger position (the plunger should have finished moving)\n# Port 6\npump /1I6R #switch to port 6, clockwise rotation\npump /1Q #query pump\npump /1?6 #report valve position\npump /1A0R #go to absolute position 0 (= pump 200 ul)\npump /1Q #query pump\npump /1? #report absolute plunger position (the plunger should be moving to 0)\nwait-min 1 #wait 1 minute\npump /1? #report absolute plunger position (the plunger should have finished moving)\n#-------------------------------------------------------\n# Cycle 22\n# Fill the syringe\n#pump /1ZR #initialize pump\npump /1Q #query pump\npump /1? #report absolute plunger position\npump /1?6 #report valve position\nwait-min 1 #wait 1 minute\npump /1N0R #set step resolution: 0.01 mm\npump /1Q #query pump\npump /1? #report absolute plunger position (the plunger should be at 0)\npump /1?6 #report valve position\nwait 1000 #wait 1 second\npump /1V300R #choose speed: 300 steps/s (6000 ul/min)\npump /1Q #query pump\nwait 1000 #wait 1 second\npump /1O3R #go to port 3, counterclockwise rotation\npump /1Q #query pump\npump /1?6 #report valve position\nwait 1000 #wait 1 second\npump /1A3000R #go to absolute position 3000 (= draw 1 ml)\nwait 30000 #wait 30 seconds\npump /1Q #query pump\npump /1? #report absolute plunger position (the plunger should have finished moving)\n#pump /1?6 #report valve position\n# The sequential pumping begins\n# Port 1\npump /1O1R #switch to port 1, counterclockwise rotation\npump /1Q #query pump\npump /1?6 #report valve position\npump /1A2400R #go to absolute position 2400 (= pump 200 ul)\npump /1Q #query pump\npump /1? #report absolute plunger position (the plunger should be moving to 0)\nwait-min 1 #wait 1 minute\npump /1? #report absolute plunger position (the plunger should have finished moving)\n# Port 2\npump /1I2R #switch to port 2, clockwise rotation\npump /1Q #query pump\npump /1?6 #report valve position\npump /1A1800R #go to absolute position 1800 (= pump 200 ul)\npump /1Q #query pump\npump /1? #report absolute plunger position (the plunger should be moving to 0)\nwait-min 1 #wait 1 minute\npump /1? #report absolute plunger position (the plunger should have finished moving)\n# Port 4\npump /1I4R #switch to port 4, clockwise rotation\npump /1Q #query pump\npump /1?6 #report valve position\npump /1A1200R #go to absolute position 1200 (= pump 200 ul)\npump /1Q #query pump\npump /1? #report absolute plunger position (the plunger should be moving to 0)\nwait-min 1 #wait 1 minute\npump /1? #report absolute plunger position (the plunger should have finished moving)\n# Port 5\npump /1I5R #switch to port 5, clockwise rotation\npump /1Q #query pump\npump /1?6 #report valve position\npump /1A600R #go to absolute position 600 (= pump 200 ul)\npump /1Q #query pump\npump /1? #report absolute plunger position (the plunger should be moving to 0)\nwait-min 1 #wait 1 minute\npump /1? #report absolute plunger position (the plunger should have finished moving)\n# Port 6\npump /1I6R #switch to port 6, clockwise rotation\npump /1Q #query pump\npump /1?6 #report valve position\npump /1A0R #go to absolute position 0 (= pump 200 ul)\npump /1Q #query pump\npump /1? #report absolute plunger position (the plunger should be moving to 0)\nwait-min 1 #wait 1 minute\npump /1? #report absolute plunger position (the plunger should have finished moving)\n#-------------------------------------------------------\n# Cycle 23\n# Fill the syringe\n#pump /1ZR #initialize pump\npump /1Q #query pump\npump /1? #report absolute plunger position\npump /1?6 #report valve position\nwait-min 1 #wait 1 minute\npump /1N0R #set step resolution: 0.01 mm\npump /1Q #query pump\npump /1? #report absolute plunger position (the plunger should be at 0)\npump /1?6 #report valve position\nwait 1000 #wait 1 second\npump /1V300R #choose speed: 300 steps/s (6000 ul/min)\npump /1Q #query pump\nwait 1000 #wait 1 second\npump /1O3R #go to port 3, counterclockwise rotation\npump /1Q #query pump\npump /1?6 #report valve position\nwait 1000 #wait 1 second\npump /1A3000R #go to absolute position 3000 (= draw 1 ml)\nwait 30000 #wait 30 seconds\npump /1Q #query pump\npump /1? #report absolute plunger position (the plunger should have finished moving)\n#pump /1?6 #report valve position\n# The sequential pumping begins\n# Port 1\npump /1O1R #switch to port 1, counterclockwise rotation\npump /1Q #query pump\npump /1?6 #report valve position\npump /1A2400R #go to absolute position 2400 (= pump 200 ul)\npump /1Q #query pump\npump /1? #report absolute plunger position (the plunger should be moving to 0)\nwait-min 1 #wait 1 minute\npump /1? #report absolute plunger position (the plunger should have finished moving)\n# Port 2\npump /1I2R #switch to port 2, clockwise rotation\npump /1Q #query pump\npump /1?6 #report valve position\npump /1A1800R #go to absolute position 1800 (= pump 200 ul)\npump /1Q #query pump\npump /1? #report absolute plunger position (the plunger should be moving to 0)\nwait-min 1 #wait 1 minute\npump /1? #report absolute plunger position (the plunger should have finished moving)\n# Port 4\npump /1I4R #switch to port 4, clockwise rotation\npump /1Q #query pump\npump /1?6 #report valve position\npump /1A1200R #go to absolute position 1200 (= pump 200 ul)\npump /1Q #query pump\npump /1? #report absolute plunger position (the plunger should be moving to 0)\nwait-min 1 #wait 1 minute\npump /1? #report absolute plunger position (the plunger should have finished moving)\n# Port 5\npump /1I5R #switch to port 5, clockwise rotation\npump /1Q #query pump\npump /1?6 #report valve position\npump /1A600R #go to absolute position 600 (= pump 200 ul)\npump /1Q #query pump\npump /1? #report absolute plunger position (the plunger should be moving to 0)\nwait-min 1 #wait 1 minute\npump /1? #report absolute plunger position (the plunger should have finished moving)\n# Port 6\npump /1I6R #switch to port 6, clockwise rotation\npump /1Q #query pump\npump /1?6 #report valve position\npump /1A0R #go to absolute position 0 (= pump 200 ul)\npump /1Q #query pump\npump /1? #report absolute plunger position (the plunger should be moving to 0)\nwait-min 1 #wait 1 minute\npump /1? #report absolute plunger position (the plunger should have finished moving)\n#-------------------------------------------------------\n# Cycle 24\n# Fill the syringe\n#pump /1ZR #initialize pump\npump /1Q #query pump\npump /1? #report absolute plunger position\npump /1?6 #report valve position\nwait-min 1 #wait 1 minute\npump /1N0R #set step resolution: 0.01 mm\npump /1Q #query pump\npump /1? #report absolute plunger position (the plunger should be at 0)\npump /1?6 #report valve position\nwait 1000 #wait 1 second\npump /1V300R #choose speed: 300 steps/s (6000 ul/min)\npump /1Q #query pump\nwait 1000 #wait 1 second\npump /1O3R #go to port 3, counterclockwise rotation\npump /1Q #query pump\npump /1?6 #report valve position\nwait 1000 #wait 1 second\npump /1A3000R #go to absolute position 3000 (= draw 1 ml)\nwait 30000 #wait 30 seconds\npump /1Q #query pump\npump /1? #report absolute plunger position (the plunger should have finished moving)\n#pump /1?6 #report valve position\n# The sequential pumping begins\n# Port 1\npump /1O1R #switch to port 1, counterclockwise rotation\npump /1Q #query pump\npump /1?6 #report valve position\npump /1A2400R #go to absolute position 2400 (= pump 200 ul)\npump /1Q #query pump\npump /1? #report absolute plunger position (the plunger should be moving to 0)\nwait-min 1 #wait 1 minute\npump /1? #report absolute plunger position (the plunger should have finished moving)\n# Port 2\npump /1I2R #switch to port 2, clockwise rotation\npump /1Q #query pump\npump /1?6 #report valve position\npump /1A1800R #go to absolute position 1800 (= pump 200 ul)\npump /1Q #query pump\npump /1? #report absolute plunger position (the plunger should be moving to 0)\nwait-min 1 #wait 1 minute\npump /1? #report absolute plunger position (the plunger should have finished moving)\n# Port 4\npump /1I4R #switch to port 4, clockwise rotation\npump /1Q #query pump\npump /1?6 #report valve position\npump /1A1200R #go to absolute position 1200 (= pump 200 ul)\npump /1Q #query pump\npump /1? #report absolute plunger position (the plunger should be moving to 0)\nwait-min 1 #wait 1 minute\npump /1? #report absolute plunger position (the plunger should have finished moving)\n# Port 5\npump /1I5R #switch to port 5, clockwise rotation\npump /1Q #query pump\npump /1?6 #report valve position\npump /1A600R #go to absolute position 600 (= pump 200 ul)\npump /1Q #query pump\npump /1? #report absolute plunger position (the plunger should be moving to 0)\nwait-min 1 #wait 1 minute\npump /1? #report absolute plunger position (the plunger should have finished moving)\n# Port 6\npump /1I6R #switch to port 6, clockwise rotation\npump /1Q #query pump\npump /1?6 #report valve position\npump /1A0R #go to absolute position 0 (= pump 200 ul)\npump /1Q #query pump\npump /1? #report absolute plunger position (the plunger should be moving to 0)\nwait-min 1 #wait 1 minute\npump /1? #report absolute plunger position (the plunger should have finished moving)\n#-------------------------------------------------------\n# Cycle 25\n# Fill the syringe\npump /1Q #query pump\npump /1? #report absolute plunger position\n#pump /1?6 #report valve position\nwait-min 1 #wait 1 minute\npump /1N0R #set step resolution: 0.01 mm\npump /1Q #query pump\npump /1? #report absolute plunger position (the plunger should be at 0)\npump /1?6 #report valve position\nwait 1000 #wait 1 second\npump /1V300R #choose speed: 300 steps/s (6000 ul/min)\npump /1Q #query pump\nwait 1000 #wait 1 second\npump /1I3R #go to port 3, clockwise rotation\npump /1Q #query pump\npump /1?6 #report valve position\nwait 1000 #wait 1 second\npump /1A3000R #go to absolute position 3000 (= draw 1 ml)\nwait 30000 #wait 30 seconds\npump /1Q #query pump\npump /1? #report absolute plunger position (the plunger should have finished moving)\n#pump /1?6 #report valve position\n# The sequential pumping begins\n# Port 1\npump /1O1R #switch to port 1, counterclockwise rotation\npump /1Q #query pump\npump /1?6 #report valve position\npump /1A2400R #go to absolute position 2400 (= pump 200 ul)\npump /1Q #query pump\npump /1? #report absolute plunger position (the plunger should be moving to 0)\nwait-min 1 #wait 1 minute\npump /1? #report absolute plunger position (the plunger should have finished moving)\n# Port 2\npump /1I2R #switch to port 2, clockwise rotation\npump /1Q #query pump\npump /1?6 #report valve position\npump /1A1800R #go to absolute position 1800 (= pump 200 ul)\npump /1Q #query pump\npump /1? #report absolute plunger position (the plunger should be moving to 0)\nwait-min 1 #wait 1 minute\npump /1? #report absolute plunger position (the plunger should have finished moving)\n# Port 4\npump /1I4R #switch to port 4, clockwise rotation\npump /1Q #query pump\npump /1?6 #report valve position\npump /1A1200R #go to absolute position 1200 (= pump 200 ul)\npump /1Q #query pump\npump /1? #report absolute plunger position (the plunger should be moving to 0)\nwait-min 1 #wait 1 minute\npump /1? #report absolute plunger position (the plunger should have finished moving)\n# Port 5\npump /1I5R #switch to port 5, clockwise rotation\npump /1Q #query pump\npump /1?6 #report valve position\npump /1A600R #go to absolute position 600 (= pump 200 ul)\npump /1Q #query pump\npump /1? #report absolute plunger position (the plunger should be moving to 0)\nwait-min 1 #wait 1 minute\npump /1? #report absolute plunger position (the plunger should have finished moving)\n# Port 6\npump /1I6R #switch to port 6, clockwise rotation\npump /1Q #query pump\npump /1?6 #report valve position\npump /1A0R #go to absolute position 0 (= pump 200 ul)\npump /1Q #query pump\npump /1? #report absolute plunger position (the plunger should be moving to 0)\nwait-min 1 #wait 1 minute\npump /1? #report absolute plunger position (the plunger should have finished moving)\n#-------------------------------------------------------\n# Cycle 26\n# Fill the syringe\n#pump /1ZR #initialize pump\npump /1Q #query pump\npump /1? #report absolute plunger position\npump /1?6 #report valve position\nwait-min 1 #wait 1 minute\npump /1N0R #set step resolution: 0.01 mm\npump /1Q #query pump\npump /1? #report absolute plunger position (the plunger should be at 0)\npump /1?6 #report valve position\nwait 1000 #wait 1 second\npump /1V300R #choose speed: 300 steps/s (6000 ul/min)\npump /1Q #query pump\nwait 1000 #wait 1 second\npump /1O3R #go to port 3, counterclockwise rotation\npump /1Q #query pump\npump /1?6 #report valve position\nwait 1000 #wait 1 second\npump /1A3000R #go to absolute position 3000 (= draw 1 ml)\nwait 30000 #wait 30 seconds\npump /1Q #query pump\npump /1? #report absolute plunger position (the plunger should have finished moving)\n#pump /1?6 #report valve position\n# The sequential pumping begins\n# Port 1\npump /1O1R #switch to port 1, counterclockwise rotation\npump /1Q #query pump\npump /1?6 #report valve position\npump /1A2400R #go to absolute position 2400 (= pump 200 ul)\npump /1Q #query pump\npump /1? #report absolute plunger position (the plunger should be moving to 0)\nwait-min 1 #wait 1 minute\npump /1? #report absolute plunger position (the plunger should have finished moving)\n# Port 2\npump /1I2R #switch to port 2, clockwise rotation\npump /1Q #query pump\npump /1?6 #report valve position\npump /1A1800R #go to absolute position 1800 (= pump 200 ul)\npump /1Q #query pump\npump /1? #report absolute plunger position (the plunger should be moving to 0)\nwait-min 1 #wait 1 minute\npump /1? #report absolute plunger position (the plunger should have finished moving)\n# Port 4\npump /1I4R #switch to port 4, clockwise rotation\npump /1Q #query pump\npump /1?6 #report valve position\npump /1A1200R #go to absolute position 1200 (= pump 200 ul)\npump /1Q #query pump\npump /1? #report absolute plunger position (the plunger should be moving to 0)\nwait-min 1 #wait 1 minute\npump /1? #report absolute plunger position (the plunger should have finished moving)\n# Port 5\npump /1I5R #switch to port 5, clockwise rotation\npump /1Q #query pump\npump /1?6 #report valve position\npump /1A600R #go to absolute position 600 (= pump 200 ul)\npump /1Q #query pump\npump /1? #report absolute plunger position (the plunger should be moving to 0)\nwait-min 1 #wait 1 minute\npump /1? #report absolute plunger position (the plunger should have finished moving)\n# Port 6\npump /1I6R #switch to port 6, clockwise rotation\npump /1Q #query pump\npump /1?6 #report valve position\npump /1A0R #go to absolute position 0 (= pump 200 ul)\npump /1Q #query pump\npump /1? #report absolute plunger position (the plunger should be moving to 0)\nwait-min 1 #wait 1 minute\npump /1? #report absolute plunger position (the plunger should have finished moving)\n#-------------------------------------------------------\n# Cycle 27\n# Fill the syringe\n#pump /1ZR #initialize pump\npump /1Q #query pump\npump /1? #report absolute plunger position\npump /1?6 #report valve position\nwait-min 1 #wait 1 minute\npump /1N0R #set step resolution: 0.01 mm\npump /1Q #query pump\npump /1? #report absolute plunger position (the plunger should be at 0)\npump /1?6 #report valve position\nwait 1000 #wait 1 second\npump /1V300R #choose speed: 300 steps/s (6000 ul/min)\npump /1Q #query pump\nwait 1000 #wait 1 second\npump /1O3R #go to port 3, counterclockwise rotation\npump /1Q #query pump\npump /1?6 #report valve position\nwait 1000 #wait 1 second\npump /1A3000R #go to absolute position 3000 (= draw 1 ml)\nwait 30000 #wait 30 seconds\npump /1Q #query pump\npump /1? #report absolute plunger position (the plunger should have finished moving)\n#pump /1?6 #report valve position\n# The sequential pumping begins\n# Port 1\npump /1O1R #switch to port 1, counterclockwise rotation\npump /1Q #query pump\npump /1?6 #report valve position\npump /1A2400R #go to absolute position 2400 (= pump 200 ul)\npump /1Q #query pump\npump /1? #report absolute plunger position (the plunger should be moving to 0)\nwait-min 1 #wait 1 minute\npump /1? #report absolute plunger position (the plunger should have finished moving)\n# Port 2\npump /1I2R #switch to port 2, clockwise rotation\npump /1Q #query pump\npump /1?6 #report valve position\npump /1A1800R #go to absolute position 1800 (= pump 200 ul)\npump /1Q #query pump\npump /1? #report absolute plunger position (the plunger should be moving to 0)\nwait-min 1 #wait 1 minute\npump /1? #report absolute plunger position (the plunger should have finished moving)\n# Port 4\npump /1I4R #switch to port 4, clockwise rotation\npump /1Q #query pump\npump /1?6 #report valve position\npump /1A1200R #go to absolute position 1200 (= pump 200 ul)\npump /1Q #query pump\npump /1? #report absolute plunger position (the plunger should be moving to 0)\nwait-min 1 #wait 1 minute\npump /1? #report absolute plunger position (the plunger should have finished moving)\n# Port 5\npump /1I5R #switch to port 5, clockwise rotation\npump /1Q #query pump\npump /1?6 #report valve position\npump /1A600R #go to absolute position 600 (= pump 200 ul)\npump /1Q #query pump\npump /1? #report absolute plunger position (the plunger should be moving to 0)\nwait-min 1 #wait 1 minute\npump /1? #report absolute plunger position (the plunger should have finished moving)\n# Port 6\npump /1I6R #switch to port 6, clockwise rotation\npump /1Q #query pump\npump /1?6 #report valve position\npump /1A0R #go to absolute position 0 (= pump 200 ul)\npump /1Q #query pump\npump /1? #report absolute plunger position (the plunger should be moving to 0)\nwait-min 1 #wait 1 minute\npump /1? #report absolute plunger position (the plunger should have finished moving)\n#-------------------------------------------------------\n# Cycle 28\n# Fill the syringe\n#pump /1ZR #initialize pump\npump /1Q #query pump\npump /1? #report absolute plunger position\npump /1?6 #report valve position\nwait-min 1 #wait 1 minute\npump /1N0R #set step resolution: 0.01 mm\npump /1Q #query pump\npump /1? #report absolute plunger position (the plunger should be at 0)\npump /1?6 #report valve position\nwait 1000 #wait 1 second\npump /1V300R #choose speed: 300 steps/s (6000 ul/min)\npump /1Q #query pump\nwait 1000 #wait 1 second\npump /1O3R #go to port 3, counterclockwise rotation\npump /1Q #query pump\npump /1?6 #report valve position\nwait 1000 #wait 1 second\npump /1A3000R #go to absolute position 3000 (= draw 1 ml)\nwait 30000 #wait 30 seconds\npump /1Q #query pump\npump /1? #report absolute plunger position (the plunger should have finished moving)\n#pump /1?6 #report valve position\n# The sequential pumping begins\n# Port 1\npump /1O1R #switch to port 1, counterclockwise rotation\npump /1Q #query pump\npump /1?6 #report valve position\npump /1A2400R #go to absolute position 2400 (= pump 200 ul)\npump /1Q #query pump\npump /1? #report absolute plunger position (the plunger should be moving to 0)\nwait-min 1 #wait 1 minute\npump /1? #report absolute plunger position (the plunger should have finished moving)\n# Port 2\npump /1I2R #switch to port 2, clockwise rotation\npump /1Q #query pump\npump /1?6 #report valve position\npump /1A1800R #go to absolute position 1800 (= pump 200 ul)\npump /1Q #query pump\npump /1? #report absolute plunger position (the plunger should be moving to 0)\nwait-min 1 #wait 1 minute\npump /1? #report absolute plunger position (the plunger should have finished moving)\n# Port 4\npump /1I4R #switch to port 4, clockwise rotation\npump /1Q #query pump\npump /1?6 #report valve position\npump /1A1200R #go to absolute position 1200 (= pump 200 ul)\npump /1Q #query pump\npump /1? #report absolute plunger position (the plunger should be moving to 0)\nwait-min 1 #wait 1 minute\npump /1? #report absolute plunger position (the plunger should have finished moving)\n# Port 5\npump /1I5R #switch to port 5, clockwise rotation\npump /1Q #query pump\npump /1?6 #report valve position\npump /1A600R #go to absolute position 600 (= pump 200 ul)\npump /1Q #query pump\npump /1? #report absolute plunger position (the plunger should be moving to 0)\nwait-min 1 #wait 1 minute\npump /1? #report absolute plunger position (the plunger should have finished moving)\n# Port 6\npump /1I6R #switch to port 6, clockwise rotation\npump /1Q #query pump\npump /1?6 #report valve position\npump /1A0R #go to absolute position 0 (= pump 200 ul)\npump /1Q #query pump\npump /1? #report absolute plunger position (the plunger should be moving to 0)\nwait-min 1 #wait 1 minute\npump /1? #report absolute plunger position (the plunger should have finished moving)\n#-------------------------------------------------------\n# Cycle 29\n# Fill the syringe\npump /1Q #query pump\npump /1? #report absolute plunger position\n#pump /1?6 #report valve position\nwait-min 1 #wait 1 minute\npump /1N0R #set step resolution: 0.01 mm\npump /1Q #query pump\npump /1? #report absolute plunger position (the plunger should be at 0)\npump /1?6 #report valve position\nwait 1000 #wait 1 second\npump /1V300R #choose speed: 300 steps/s (6000 ul/min)\npump /1Q #query pump\nwait 1000 #wait 1 second\npump /1I3R #go to port 3, clockwise rotation\npump /1Q #query pump\npump /1?6 #report valve position\nwait 1000 #wait 1 second\npump /1A3000R #go to absolute position 3000 (= draw 1 ml)\nwait 30000 #wait 30 seconds\npump /1Q #query pump\npump /1? #report absolute plunger position (the plunger should have finished moving)\n#pump /1?6 #report valve position\n# The sequential pumping begins\n# Port 1\npump /1O1R #switch to port 1, counterclockwise rotation\npump /1Q #query pump\npump /1?6 #report valve position\npump /1A2400R #go to absolute position 2400 (= pump 200 ul)\npump /1Q #query pump\npump /1? #report absolute plunger position (the plunger should be moving to 0)\nwait-min 1 #wait 1 minute\npump /1? #report absolute plunger position (the plunger should have finished moving)\n# Port 2\npump /1I2R #switch to port 2, clockwise rotation\npump /1Q #query pump\npump /1?6 #report valve position\npump /1A1800R #go to absolute position 1800 (= pump 200 ul)\npump /1Q #query pump\npump /1? #report absolute plunger position (the plunger should be moving to 0)\nwait-min 1 #wait 1 minute\npump /1? #report absolute plunger position (the plunger should have finished moving)\n# Port 4\npump /1I4R #switch to port 4, clockwise rotation\npump /1Q #query pump\npump /1?6 #report valve position\npump /1A1200R #go to absolute position 1200 (= pump 200 ul)\npump /1Q #query pump\npump /1? #report absolute plunger position (the plunger should be moving to 0)\nwait-min 1 #wait 1 minute\npump /1? #report absolute plunger position (the plunger should have finished moving)\n# Port 5\npump /1I5R #switch to port 5, clockwise rotation\npump /1Q #query pump\npump /1?6 #report valve position\npump /1A600R #go to absolute position 600 (= pump 200 ul)\npump /1Q #query pump\npump /1? #report absolute plunger position (the plunger should be moving to 0)\nwait-min 1 #wait 1 minute\npump /1? #report absolute plunger position (the plunger should have finished moving)\n# Port 6\npump /1I6R #switch to port 6, clockwise rotation\npump /1Q #query pump\npump /1?6 #report valve position\npump /1A0R #go to absolute position 0 (= pump 200 ul)\npump /1Q #query pump\npump /1? #report absolute plunger position (the plunger should be moving to 0)\nwait-min 1 #wait 1 minute\npump /1? #report absolute plunger position (the plunger should have finished moving)\n#-------------------------------------------------------\n# Cycle 30\n# Fill the syringe\n#pump /1ZR #initialize pump\npump /1Q #query pump\npump /1? #report absolute plunger position\npump /1?6 #report valve position\nwait-min 1 #wait 1 minute\npump /1N0R #set step resolution: 0.01 mm\npump /1Q #query pump\npump /1? #report absolute plunger position (the plunger should be at 0)\npump /1?6 #report valve position\nwait 1000 #wait 1 second\npump /1V300R #choose speed: 300 steps/s (6000 ul/min)\npump /1Q #query pump\nwait 1000 #wait 1 second\npump /1O3R #go to port 3, counterclockwise rotation\npump /1Q #query pump\npump /1?6 #report valve position\nwait 1000 #wait 1 second\npump /1A3000R #go to absolute position 3000 (= draw 1 ml)\nwait 30000 #wait 30 seconds\npump /1Q #query pump\npump /1? #report absolute plunger position (the plunger should have finished moving)\n#pump /1?6 #report valve position\n# The sequential pumping begins\n# Port 1\npump /1O1R #switch to port 1, counterclockwise rotation\npump /1Q #query pump\npump /1?6 #report valve position\npump /1A2400R #go to absolute position 2400 (= pump 200 ul)\npump /1Q #query pump\npump /1? #report absolute plunger position (the plunger should be moving to 0)\nwait-min 1 #wait 1 minute\npump /1? #report absolute plunger position (the plunger should have finished moving)\n# Port 2\npump /1I2R #switch to port 2, clockwise rotation\npump /1Q #query pump\npump /1?6 #report valve position\npump /1A1800R #go to absolute position 1800 (= pump 200 ul)\npump /1Q #query pump\npump /1? #report absolute plunger position (the plunger should be moving to 0)\nwait-min 1 #wait 1 minute\npump /1? #report absolute plunger position (the plunger should have finished moving)\n# Port 4\npump /1I4R #switch to port 4, clockwise rotation\npump /1Q #query pump\npump /1?6 #report valve position\npump /1A1200R #go to absolute position 1200 (= pump 200 ul)\npump /1Q #query pump\npump /1? #report absolute plunger position (the plunger should be moving to 0)\nwait-min 1 #wait 1 minute\npump /1? #report absolute plunger position (the plunger should have finished moving)\n# Port 5\npump /1I5R #switch to port 5, clockwise rotation\npump /1Q #query pump\npump /1?6 #report valve position\npump /1A600R #go to absolute position 600 (= pump 200 ul)\npump /1Q #query pump\npump /1? #report absolute plunger position (the plunger should be moving to 0)\nwait-min 1 #wait 1 minute\npump /1? #report absolute plunger position (the plunger should have finished moving)\n# Port 6\npump /1I6R #switch to port 6, clockwise rotation\npump /1Q #query pump\npump /1?6 #report valve position\npump /1A0R #go to absolute position 0 (= pump 200 ul)\npump /1Q #query pump\npump /1? #report absolute plunger position (the plunger should be moving to 0)\nwait-min 1 #wait 1 minute\npump /1? #report absolute plunger position (the plunger should have finished moving)\n#-------------------------------------------------------\n# Cycle 31\n# Fill the syringe\n#pump /1ZR #initialize pump\npump /1Q #query pump\npump /1? #report absolute plunger position\npump /1?6 #report valve position\nwait-min 1 #wait 1 minute\npump /1N0R #set step resolution: 0.01 mm\npump /1Q #query pump\npump /1? #report absolute plunger position (the plunger should be at 0)\npump /1?6 #report valve position\nwait 1000 #wait 1 second\npump /1V300R #choose speed: 300 steps/s (6000 ul/min)\npump /1Q #query pump\nwait 1000 #wait 1 second\npump /1O3R #go to port 3, counterclockwise rotation\npump /1Q #query pump\npump /1?6 #report valve position\nwait 1000 #wait 1 second\npump /1A3000R #go to absolute position 3000 (= draw 1 ml)\nwait 30000 #wait 30 seconds\npump /1Q #query pump\npump /1? #report absolute plunger position (the plunger should have finished moving)\n#pump /1?6 #report valve position\n# The sequential pumping begins\n# Port 1\npump /1O1R #switch to port 1, counterclockwise rotation\npump /1Q #query pump\npump /1?6 #report valve position\npump /1A2400R #go to absolute position 2400 (= pump 200 ul)\npump /1Q #query pump\npump /1? #report absolute plunger position (the plunger should be moving to 0)\nwait-min 1 #wait 1 minute\npump /1? #report absolute plunger position (the plunger should have finished moving)\n# Port 2\npump /1I2R #switch to port 2, clockwise rotation\npump /1Q #query pump\npump /1?6 #report valve position\npump /1A1800R #go to absolute position 1800 (= pump 200 ul)\npump /1Q #query pump\npump /1? #report absolute plunger position (the plunger should be moving to 0)\nwait-min 1 #wait 1 minute\npump /1? #report absolute plunger position (the plunger should have finished moving)\n# Port 4\npump /1I4R #switch to port 4, clockwise rotation\npump /1Q #query pump\npump /1?6 #report valve position\npump /1A1200R #go to absolute position 1200 (= pump 200 ul)\npump /1Q #query pump\npump /1? #report absolute plunger position (the plunger should be moving to 0)\nwait-min 1 #wait 1 minute\npump /1? #report absolute plunger position (the plunger should have finished moving)\n# Port 5\npump /1I5R #switch to port 5, clockwise rotation\npump /1Q #query pump\npump /1?6 #report valve position\npump /1A600R #go to absolute position 600 (= pump 200 ul)\npump /1Q #query pump\npump /1? #report absolute plunger position (the plunger should be moving to 0)\nwait-min 1 #wait 1 minute\npump /1? #report absolute plunger position (the plunger should have finished moving)\n# Port 6\npump /1I6R #switch to port 6, clockwise rotation\npump /1Q #query pump\npump /1?6 #report valve position\npump /1A0R #go to absolute position 0 (= pump 200 ul)\npump /1Q #query pump\npump /1? #report absolute plunger position (the plunger should be moving to 0)\nwait-min 1 #wait 1 minute\npump /1? #report absolute plunger position (the plunger should have finished moving)\n#-------------------------------------------------------\n# Cycle 32\n# Fill the syringe\n#pump /1ZR #initialize pump\npump /1Q #query pump\npump /1? #report absolute plunger position\npump /1?6 #report valve position\nwait-min 1 #wait 1 minute\npump /1N0R #set step resolution: 0.01 mm\npump /1Q #query pump\npump /1? #report absolute plunger position (the plunger should be at 0)\npump /1?6 #report valve position\nwait 1000 #wait 1 second\npump /1V300R #choose speed: 300 steps/s (6000 ul/min)\npump /1Q #query pump\nwait 1000 #wait 1 second\npump /1O3R #go to port 3, counterclockwise rotation\npump /1Q #query pump\npump /1?6 #report valve position\nwait 1000 #wait 1 second\npump /1A3000R #go to absolute position 3000 (= draw 1 ml)\nwait 30000 #wait 30 seconds\npump /1Q #query pump\npump /1? #report absolute plunger position (the plunger should have finished moving)\n#pump /1?6 #report valve position\n# The sequential pumping begins\n# Port 1\npump /1O1R #switch to port 1, counterclockwise rotation\npump /1Q #query pump\npump /1?6 #report valve position\npump /1A2400R #go to absolute position 2400 (= pump 200 ul)\npump /1Q #query pump\npump /1? #report absolute plunger position (the plunger should be moving to 0)\nwait-min 1 #wait 1 minute\npump /1? #report absolute plunger position (the plunger should have finished moving)\n# Port 2\npump /1I2R #switch to port 2, clockwise rotation\npump /1Q #query pump\npump /1?6 #report valve position\npump /1A1800R #go to absolute position 1800 (= pump 200 ul)\npump /1Q #query pump\npump /1? #report absolute plunger position (the plunger should be moving to 0)\nwait-min 1 #wait 1 minute\npump /1? #report absolute plunger position (the plunger should have finished moving)\n# Port 4\npump /1I4R #switch to port 4, clockwise rotation\npump /1Q #query pump\npump /1?6 #report valve position\npump /1A1200R #go to absolute position 1200 (= pump 200 ul)\npump /1Q #query pump\npump /1? #report absolute plunger position (the plunger should be moving to 0)\nwait-min 1 #wait 1 minute\npump /1? #report absolute plunger position (the plunger should have finished moving)\n# Port 5\npump /1I5R #switch to port 5, clockwise rotation\npump /1Q #query pump\npump /1?6 #report valve position\npump /1A600R #go to absolute position 600 (= pump 200 ul)\npump /1Q #query pump\npump /1? #report absolute plunger position (the plunger should be moving to 0)\nwait-min 1 #wait 1 minute\npump /1? #report absolute plunger position (the plunger should have finished moving)\n# Port 6\npump /1I6R #switch to port 6, clockwise rotation\npump /1Q #query pump\npump /1?6 #report valve position\npump /1A0R #go to absolute position 0 (= pump 200 ul)\npump /1Q #query pump\npump /1? #report absolute plunger position (the plunger should be moving to 0)\nwait-min 1 #wait 1 minute\npump /1? #report absolute plunger position (the plunger should have finished moving)\n#-------------------------------------------------------\n# Cycle 33\n# Fill the syringe\npump /1Q #query pump\npump /1? #report absolute plunger position\n#pump /1?6 #report valve position\nwait-min 1 #wait 1 minute\npump /1N0R #set step resolution: 0.01 mm\npump /1Q #query pump\npump /1? #report absolute plunger position (the plunger should be at 0)\npump /1?6 #report valve position\nwait 1000 #wait 1 second\npump /1V300R #choose speed: 300 steps/s (6000 ul/min)\npump /1Q #query pump\nwait 1000 #wait 1 second\npump /1I3R #go to port 3, clockwise rotation\npump /1Q #query pump\npump /1?6 #report valve position\nwait 1000 #wait 1 second\npump /1A3000R #go to absolute position 3000 (= draw 1 ml)\nwait 30000 #wait 30 seconds\npump /1Q #query pump\npump /1? #report absolute plunger position (the plunger should have finished moving)\n#pump /1?6 #report valve position\n# The sequential pumping begins\n# Port 1\npump /1O1R #switch to port 1, counterclockwise rotation\npump /1Q #query pump\npump /1?6 #report valve position\npump /1A2400R #go to absolute position 2400 (= pump 200 ul)\npump /1Q #query pump\npump /1? #report absolute plunger position (the plunger should be moving to 0)\nwait-min 1 #wait 1 minute\npump /1? #report absolute plunger position (the plunger should have finished moving)\n# Port 2\npump /1I2R #switch to port 2, clockwise rotation\npump /1Q #query pump\npump /1?6 #report valve position\npump /1A1800R #go to absolute position 1800 (= pump 200 ul)\npump /1Q #query pump\npump /1? #report absolute plunger position (the plunger should be moving to 0)\nwait-min 1 #wait 1 minute\npump /1? #report absolute plunger position (the plunger should have finished moving)\n# Port 4\npump /1I4R #switch to port 4, clockwise rotation\npump /1Q #query pump\npump /1?6 #report valve position\npump /1A1200R #go to absolute position 1200 (= pump 200 ul)\npump /1Q #query pump\npump /1? #report absolute plunger position (the plunger should be moving to 0)\nwait-min 1 #wait 1 minute\npump /1? #report absolute plunger position (the plunger should have finished moving)\n# Port 5\npump /1I5R #switch to port 5, clockwise rotation\npump /1Q #query pump\npump /1?6 #report valve position\npump /1A600R #go to absolute position 600 (= pump 200 ul)\npump /1Q #query pump\npump /1? #report absolute plunger position (the plunger should be moving to 0)\nwait-min 1 #wait 1 minute\npump /1? #report absolute plunger position (the plunger should have finished moving)\n# Port 6\npump /1I6R #switch to port 6, clockwise rotation\npump /1Q #query pump\npump /1?6 #report valve position\npump /1A0R #go to absolute position 0 (= pump 200 ul)\npump /1Q #query pump\npump /1? #report absolute plunger position (the plunger should be moving to 0)\nwait-min 1 #wait 1 minute\npump /1? #report absolute plunger position (the plunger should have finished moving)\n#-------------------------------------------------------\n# Cycle 34\n# Fill the syringe\n#pump /1ZR #initialize pump\npump /1Q #query pump\npump /1? #report absolute plunger position\npump /1?6 #report valve position\nwait-min 1 #wait 1 minute\npump /1N0R #set step resolution: 0.01 mm\npump /1Q #query pump\npump /1? #report absolute plunger position (the plunger should be at 0)\npump /1?6 #report valve position\nwait 1000 #wait 1 second\npump /1V300R #choose speed: 300 steps/s (6000 ul/min)\npump /1Q #query pump\nwait 1000 #wait 1 second\npump /1O3R #go to port 3, counterclockwise rotation\npump /1Q #query pump\npump /1?6 #report valve position\nwait 1000 #wait 1 second\npump /1A3000R #go to absolute position 3000 (= draw 1 ml)\nwait 30000 #wait 30 seconds\npump /1Q #query pump\npump /1? #report absolute plunger position (the plunger should have finished moving)\n#pump /1?6 #report valve position\n# The sequential pumping begins\n# Port 1\npump /1O1R #switch to port 1, counterclockwise rotation\npump /1Q #query pump\npump /1?6 #report valve position\npump /1A2400R #go to absolute position 2400 (= pump 200 ul)\npump /1Q #query pump\npump /1? #report absolute plunger position (the plunger should be moving to 0)\nwait-min 1 #wait 1 minute\npump /1? #report absolute plunger position (the plunger should have finished moving)\n# Port 2\npump /1I2R #switch to port 2, clockwise rotation\npump /1Q #query pump\npump /1?6 #report valve position\npump /1A1800R #go to absolute position 1800 (= pump 200 ul)\npump /1Q #query pump\npump /1? #report absolute plunger position (the plunger should be moving to 0)\nwait-min 1 #wait 1 minute\npump /1? #report absolute plunger position (the plunger should have finished moving)\n# Port 4\npump /1I4R #switch to port 4, clockwise rotation\npump /1Q #query pump\npump /1?6 #report valve position\npump /1A1200R #go to absolute position 1200 (= pump 200 ul)\npump /1Q #query pump\npump /1? #report absolute plunger position (the plunger should be moving to 0)\nwait-min 1 #wait 1 minute\npump /1? #report absolute plunger position (the plunger should have finished moving)\n# Port 5\npump /1I5R #switch to port 5, clockwise rotation\npump /1Q #query pump\npump /1?6 #report valve position\npump /1A600R #go to absolute position 600 (= pump 200 ul)\npump /1Q #query pump\npump /1? #report absolute plunger position (the plunger should be moving to 0)\nwait-min 1 #wait 1 minute\npump /1? #report absolute plunger position (the plunger should have finished moving)\n# Port 6\npump /1I6R #switch to port 6, clockwise rotation\npump /1Q #query pump\npump /1?6 #report valve position\npump /1A0R #go to absolute position 0 (= pump 200 ul)\npump /1Q #query pump\npump /1? #report absolute plunger position (the plunger should be moving to 0)\nwait-min 1 #wait 1 minute\npump /1? #report absolute plunger position (the plunger should have finished moving)\n#-------------------------------------------------------\n# Cycle 35\n# Fill the syringe\n#pump /1ZR #initialize pump\npump /1Q #query pump\npump /1? #report absolute plunger position\npump /1?6 #report valve position\nwait-min 1 #wait 1 minute\npump /1N0R #set step resolution: 0.01 mm\npump /1Q #query pump\npump /1? #report absolute plunger position (the plunger should be at 0)\npump /1?6 #report valve position\nwait 1000 #wait 1 second\npump /1V300R #choose speed: 300 steps/s (6000 ul/min)\npump /1Q #query pump\nwait 1000 #wait 1 second\npump /1O3R #go to port 3, counterclockwise rotation\npump /1Q #query pump\npump /1?6 #report valve position\nwait 1000 #wait 1 second\npump /1A3000R #go to absolute position 3000 (= draw 1 ml)\nwait 30000 #wait 30 seconds\npump /1Q #query pump\npump /1? #report absolute plunger position (the plunger should have finished moving)\n#pump /1?6 #report valve position\n# The sequential pumping begins\n# Port 1\npump /1O1R #switch to port 1, counterclockwise rotation\npump /1Q #query pump\npump /1?6 #report valve position\npump /1A2400R #go to absolute position 2400 (= pump 200 ul)\npump /1Q #query pump\npump /1? #report absolute plunger position (the plunger should be moving to 0)\nwait-min 1 #wait 1 minute\npump /1? #report absolute plunger position (the plunger should have finished moving)\n# Port 2\npump /1I2R #switch to port 2, clockwise rotation\npump /1Q #query pump\npump /1?6 #report valve position\npump /1A1800R #go to absolute position 1800 (= pump 200 ul)\npump /1Q #query pump\npump /1? #report absolute plunger position (the plunger should be moving to 0)\nwait-min 1 #wait 1 minute\npump /1? #report absolute plunger position (the plunger should have finished moving)\n# Port 4\npump /1I4R #switch to port 4, clockwise rotation\npump /1Q #query pump\npump /1?6 #report valve position\npump /1A1200R #go to absolute position 1200 (= pump 200 ul)\npump /1Q #query pump\npump /1? #report absolute plunger position (the plunger should be moving to 0)\nwait-min 1 #wait 1 minute\npump /1? #report absolute plunger position (the plunger should have finished moving)\n# Port 5\npump /1I5R #switch to port 5, clockwise rotation\npump /1Q #query pump\npump /1?6 #report valve position\npump /1A600R #go to absolute position 600 (= pump 200 ul)\npump /1Q #query pump\npump /1? #report absolute plunger position (the plunger should be moving to 0)\nwait-min 1 #wait 1 minute\npump /1? #report absolute plunger position (the plunger should have finished moving)\n# Port 6\npump /1I6R #switch to port 6, clockwise rotation\npump /1Q #query pump\npump /1?6 #report valve position\npump /1A0R #go to absolute position 0 (= pump 200 ul)\npump /1Q #query pump\npump /1? #report absolute plunger position (the plunger should be moving to 0)\nwait-min 1 #wait 1 minute\npump /1? #report absolute plunger position (the plunger should have finished moving)\n#-------------------------------------------------------\n# Cycle 36\n# Fill the syringe\n#pump /1ZR #initialize pump\npump /1Q #query pump\npump /1? #report absolute plunger position\npump /1?6 #report valve position\nwait-min 1 #wait 1 minute\npump /1N0R #set step resolution: 0.01 mm\npump /1Q #query pump\npump /1? #report absolute plunger position (the plunger should be at 0)\npump /1?6 #report valve position\nwait 1000 #wait 1 second\npump /1V300R #choose speed: 300 steps/s (6000 ul/min)\npump /1Q #query pump\nwait 1000 #wait 1 second\npump /1O3R #go to port 3, counterclockwise rotation\npump /1Q #query pump\npump /1?6 #report valve position\nwait 1000 #wait 1 second\npump /1A3000R #go to absolute position 3000 (= draw 1 ml)\nwait 30000 #wait 30 seconds\npump /1Q #query pump\npump /1? #report absolute plunger position (the plunger should have finished moving)\n#pump /1?6 #report valve position\n# The sequential pumping begins\n# Port 1\npump /1O1R #switch to port 1, counterclockwise rotation\npump /1Q #query pump\npump /1?6 #report valve position\npump /1A2400R #go to absolute position 2400 (= pump 200 ul)\npump /1Q #query pump\npump /1? #report absolute plunger position (the plunger should be moving to 0)\nwait-min 1 #wait 1 minute\npump /1? #report absolute plunger position (the plunger should have finished moving)\n# Port 2\npump /1I2R #switch to port 2, clockwise rotation\npump /1Q #query pump\npump /1?6 #report valve position\npump /1A1800R #go to absolute position 1800 (= pump 200 ul)\npump /1Q #query pump\npump /1? #report absolute plunger position (the plunger should be moving to 0)\nwait-min 1 #wait 1 minute\npump /1? #report absolute plunger position (the plunger should have finished moving)\n# Port 4\npump /1I4R #switch to port 4, clockwise rotation\npump /1Q #query pump\npump /1?6 #report valve position\npump /1A1200R #go to absolute position 1200 (= pump 200 ul)\npump /1Q #query pump\npump /1? #report absolute plunger position (the plunger should be moving to 0)\nwait-min 1 #wait 1 minute\npump /1? #report absolute plunger position (the plunger should have finished moving)\n# Port 5\npump /1I5R #switch to port 5, clockwise rotation\npump /1Q #query pump\npump /1?6 #report valve position\npump /1A600R #go to absolute position 600 (= pump 200 ul)\npump /1Q #query pump\npump /1? #report absolute plunger position (the plunger should be moving to 0)\nwait-min 1 #wait 1 minute\npump /1? #report absolute plunger position (the plunger should have finished moving)\n# Port 6\npump /1I6R #switch to port 6, clockwise rotation\npump /1Q #query pump\npump /1?6 #report valve position\npump /1A0R #go to absolute position 0 (= pump 200 ul)\npump /1Q #query pump\npump /1? #report absolute plunger position (the plunger should be moving to 0)\nwait-min 1 #wait 1 minute\npump /1? #report absolute plunger position (the plunger should have finished moving)\n#-------------------------------------------------------\n# Cycle 37\n# Fill the syringe\npump /1Q #query pump\npump /1? #report absolute plunger position\n#pump /1?6 #report valve position\nwait-min 1 #wait 1 minute\npump /1N0R #set step resolution: 0.01 mm\npump /1Q #query pump\npump /1? #report absolute plunger position (the plunger should be at 0)\npump /1?6 #report valve position\nwait 1000 #wait 1 second\npump /1V300R #choose speed: 300 steps/s (6000 ul/min)\npump /1Q #query pump\nwait 1000 #wait 1 second\npump /1I3R #go to port 3, clockwise rotation\npump /1Q #query pump\npump /1?6 #report valve position\nwait 1000 #wait 1 second\npump /1A3000R #go to absolute position 3000 (= draw 1 ml)\nwait 30000 #wait 30 seconds\npump /1Q #query pump\npump /1? #report absolute plunger position (the plunger should have finished moving)\n#pump /1?6 #report valve position\n# The sequential pumping begins\n# Port 1\npump /1O1R #switch to port 1, counterclockwise rotation\npump /1Q #query pump\npump /1?6 #report valve position\npump /1A2400R #go to absolute position 2400 (= pump 200 ul)\npump /1Q #query pump\npump /1? #report absolute plunger position (the plunger should be moving to 0)\nwait-min 1 #wait 1 minute\npump /1? #report absolute plunger position (the plunger should have finished moving)\n# Port 2\npump /1I2R #switch to port 2, clockwise rotation\npump /1Q #query pump\npump /1?6 #report valve position\npump /1A1800R #go to absolute position 1800 (= pump 200 ul)\npump /1Q #query pump\npump /1? #report absolute plunger position (the plunger should be moving to 0)\nwait-min 1 #wait 1 minute\npump /1? #report absolute plunger position (the plunger should have finished moving)\n# Port 4\npump /1I4R #switch to port 4, clockwise rotation\npump /1Q #query pump\npump /1?6 #report valve position\npump /1A1200R #go to absolute position 1200 (= pump 200 ul)\npump /1Q #query pump\npump /1? #report absolute plunger position (the plunger should be moving to 0)\nwait-min 1 #wait 1 minute\npump /1? #report absolute plunger position (the plunger should have finished moving)\n# Port 5\npump /1I5R #switch to port 5, clockwise rotation\npump /1Q #query pump\npump /1?6 #report valve position\npump /1A600R #go to absolute position 600 (= pump 200 ul)\npump /1Q #query pump\npump /1? #report absolute plunger position (the plunger should be moving to 0)\nwait-min 1 #wait 1 minute\npump /1? #report absolute plunger position (the plunger should have finished moving)\n# Port 6\npump /1I6R #switch to port 6, clockwise rotation\npump /1Q #query pump\npump /1?6 #report valve position\npump /1A0R #go to absolute position 0 (= pump 200 ul)\npump /1Q #query pump\npump /1? #report absolute plunger position (the plunger should be moving to 0)\nwait-min 1 #wait 1 minute\npump /1? #report absolute plunger position (the plunger should have finished moving)\n#-------------------------------------------------------\n# Cycle 38\n# Fill the syringe\n#pump /1ZR #initialize pump\npump /1Q #query pump\npump /1? #report absolute plunger position\npump /1?6 #report valve position\nwait-min 1 #wait 1 minute\npump /1N0R #set step resolution: 0.01 mm\npump /1Q #query pump\npump /1? #report absolute plunger position (the plunger should be at 0)\npump /1?6 #report valve position\nwait 1000 #wait 1 second\npump /1V300R #choose speed: 300 steps/s (6000 ul/min)\npump /1Q #query pump\nwait 1000 #wait 1 second\npump /1O3R #go to port 3, counterclockwise rotation\npump /1Q #query pump\npump /1?6 #report valve position\nwait 1000 #wait 1 second\npump /1A3000R #go to absolute position 3000 (= draw 1 ml)\nwait 30000 #wait 30 seconds\npump /1Q #query pump\npump /1? #report absolute plunger position (the plunger should have finished moving)\n#pump /1?6 #report valve position\n# The sequential pumping begins\n# Port 1\npump /1O1R #switch to port 1, counterclockwise rotation\npump /1Q #query pump\npump /1?6 #report valve position\npump /1A2400R #go to absolute position 2400 (= pump 200 ul)\npump /1Q #query pump\npump /1? #report absolute plunger position (the plunger should be moving to 0)\nwait-min 1 #wait 1 minute\npump /1? #report absolute plunger position (the plunger should have finished moving)\n# Port 2\npump /1I2R #switch to port 2, clockwise rotation\npump /1Q #query pump\npump /1?6 #report valve position\npump /1A1800R #go to absolute position 1800 (= pump 200 ul)\npump /1Q #query pump\npump /1? #report absolute plunger position (the plunger should be moving to 0)\nwait-min 1 #wait 1 minute\npump /1? #report absolute plunger position (the plunger should have finished moving)\n# Port 4\npump /1I4R #switch to port 4, clockwise rotation\npump /1Q #query pump\npump /1?6 #report valve position\npump /1A1200R #go to absolute position 1200 (= pump 200 ul)\npump /1Q #query pump\npump /1? #report absolute plunger position (the plunger should be moving to 0)\nwait-min 1 #wait 1 minute\npump /1? #report absolute plunger position (the plunger should have finished moving)\n# Port 5\npump /1I5R #switch to port 5, clockwise rotation\npump /1Q #query pump\npump /1?6 #report valve position\npump /1A600R #go to absolute position 600 (= pump 200 ul)\npump /1Q #query pump\npump /1? #report absolute plunger position (the plunger should be moving to 0)\nwait-min 1 #wait 1 minute\npump /1? #report absolute plunger position (the plunger should have finished moving)\n# Port 6\npump /1I6R #switch to port 6, clockwise rotation\npump /1Q #query pump\npump /1?6 #report valve position\npump /1A0R #go to absolute position 0 (= pump 200 ul)\npump /1Q #query pump\npump /1? #report absolute plunger position (the plunger should be moving to 0)\nwait-min 1 #wait 1 minute\npump /1? #report absolute plunger position (the plunger should have finished moving)\n#-------------------------------------------------------\n# Cycle 39\n# Fill the syringe\n#pump /1ZR #initialize pump\npump /1Q #query pump\npump /1? #report absolute plunger position\npump /1?6 #report valve position\nwait-min 1 #wait 1 minute\npump /1N0R #set step resolution: 0.01 mm\npump /1Q #query pump\npump /1? #report absolute plunger position (the plunger should be at 0)\npump /1?6 #report valve position\nwait 1000 #wait 1 second\npump /1V300R #choose speed: 300 steps/s (6000 ul/min)\npump /1Q #query pump\nwait 1000 #wait 1 second\npump /1O3R #go to port 3, counterclockwise rotation\npump /1Q #query pump\npump /1?6 #report valve position\nwait 1000 #wait 1 second\npump /1A3000R #go to absolute position 3000 (= draw 1 ml)\nwait 30000 #wait 30 seconds\npump /1Q #query pump\npump /1? #report absolute plunger position (the plunger should have finished moving)\n#pump /1?6 #report valve position\n# The sequential pumping begins\n# Port 1\npump /1O1R #switch to port 1, counterclockwise rotation\npump /1Q #query pump\npump /1?6 #report valve position\npump /1A2400R #go to absolute position 2400 (= pump 200 ul)\npump /1Q #query pump\npump /1? #report absolute plunger position (the plunger should be moving to 0)\nwait-min 1 #wait 1 minute\npump /1? #report absolute plunger position (the plunger should have finished moving)\n# Port 2\npump /1I2R #switch to port 2, clockwise rotation\npump /1Q #query pump\npump /1?6 #report valve position\npump /1A1800R #go to absolute position 1800 (= pump 200 ul)\npump /1Q #query pump\npump /1? #report absolute plunger position (the plunger should be moving to 0)\nwait-min 1 #wait 1 minute\npump /1? #report absolute plunger position (the plunger should have finished moving)\n# Port 4\npump /1I4R #switch to port 4, clockwise rotation\npump /1Q #query pump\npump /1?6 #report valve position\npump /1A1200R #go to absolute position 1200 (= pump 200 ul)\npump /1Q #query pump\npump /1? #report absolute plunger position (the plunger should be moving to 0)\nwait-min 1 #wait 1 minute\npump /1? #report absolute plunger position (the plunger should have finished moving)\n# Port 5\npump /1I5R #switch to port 5, clockwise rotation\npump /1Q #query pump\npump /1?6 #report valve position\npump /1A600R #go to absolute position 600 (= pump 200 ul)\npump /1Q #query pump\npump /1? #report absolute plunger position (the plunger should be moving to 0)\nwait-min 1 #wait 1 minute\npump /1? #report absolute plunger position (the plunger should have finished moving)\n# Port 6\npump /1I6R #switch to port 6, clockwise rotation\npump /1Q #query pump\npump /1?6 #report valve position\npump /1A0R #go to absolute position 0 (= pump 200 ul)\npump /1Q #query pump\npump /1? #report absolute plunger position (the plunger should be moving to 0)\nwait-min 1 #wait 1 minute\npump /1? #report absolute plunger position (the plunger should have finished moving)\n#-------------------------------------------------------\n# Cycle 40\n# Fill the syringe\n#pump /1ZR #initialize pump\npump /1Q #query pump\npump /1? #report absolute plunger position\npump /1?6 #report valve position\nwait-min 1 #wait 1 minute\npump /1N0R #set step resolution: 0.01 mm\npump /1Q #query pump\npump /1? #report absolute plunger position (the plunger should be at 0)\npump /1?6 #report valve position\nwait 1000 #wait 1 second\npump /1V300R #choose speed: 300 steps/s (6000 ul/min)\npump /1Q #query pump\nwait 1000 #wait 1 second\npump /1O3R #go to port 3, counterclockwise rotation\npump /1Q #query pump\npump /1?6 #report valve position\nwait 1000 #wait 1 second\npump /1A3000R #go to absolute position 3000 (= draw 1 ml)\nwait 30000 #wait 30 seconds\npump /1Q #query pump\npump /1? #report absolute plunger position (the plunger should have finished moving)\n#pump /1?6 #report valve position\n# The sequential pumping begins\n# Port 1\npump /1O1R #switch to port 1, counterclockwise rotation\npump /1Q #query pump\npump /1?6 #report valve position\npump /1A2400R #go to absolute position 2400 (= pump 200 ul)\npump /1Q #query pump\npump /1? #report absolute plunger position (the plunger should be moving to 0)\nwait-min 1 #wait 1 minute\npump /1? #report absolute plunger position (the plunger should have finished moving)\n# Port 2\npump /1I2R #switch to port 2, clockwise rotation\npump /1Q #query pump\npump /1?6 #report valve position\npump /1A1800R #go to absolute position 1800 (= pump 200 ul)\npump /1Q #query pump\npump /1? #report absolute plunger position (the plunger should be moving to 0)\nwait-min 1 #wait 1 minute\npump /1? #report absolute plunger position (the plunger should have finished moving)\n# Port 4\npump /1I4R #switch to port 4, clockwise rotation\npump /1Q #query pump\npump /1?6 #report valve position\npump /1A1200R #go to absolute position 1200 (= pump 200 ul)\npump /1Q #query pump\npump /1? #report absolute plunger position (the plunger should be moving to 0)\nwait-min 1 #wait 1 minute\npump /1? #report absolute plunger position (the plunger should have finished moving)\n# Port 5\npump /1I5R #switch to port 5, clockwise rotation\npump /1Q #query pump\npump /1?6 #report valve position\npump /1A600R #go to absolute position 600 (= pump 200 ul)\npump /1Q #query pump\npump /1? #report absolute plunger position (the plunger should be moving to 0)\nwait-min 1 #wait 1 minute\npump /1? #report absolute plunger position (the plunger should have finished moving)\n# Port 6\npump /1I6R #switch to port 6, clockwise rotation\npump /1Q #query pump\npump /1?6 #report valve position\npump /1A0R #go to absolute position 0 (= pump 200 ul)\npump /1Q #query pump\npump /1? #report absolute plunger position (the plunger should be moving to 0)\nwait-min 1 #wait 1 minute\npump /1? #report absolute plunger position (the plunger should have finished moving)\n#-------------------------------------------------------"
  out "Command running:":string
  out "Serial port data":string
  out "Elapsed Time":dbl caption="Elapsed Time (s)"
  in  "Time Units":u16(ring)=1 items=["Seconds", "Minutes", "Hours"]
  in  "Time Offset":dbl caption="Set Start Time (s)"
  in  "Reset":bool
  in  "Auto Reset":bool
  in  "integration time":u32(slide) max=2 step=1 scale=0.0..2.0
  in  "Interrupt scan":bool
  out "Absolute plunger position vs time":cluster{"Y data in":dbl[], "X data in":dbl[]}[](graph)
  out "Valve position vs time":cluster{"Y data in":dbl[], "X data in":dbl[]}[](graph)
  out "Is on":dbl format="%.2e"
  out "Id on":dbl format="%.2e"
  out "Ig on":dbl format="%.2e"
  out "Ion vs time":cluster{"Y data in":dbl[], "X data in":dbl[]}[](graph)
  out "Ioff vs time":cluster{"Y data in":dbl[], "X data in":dbl[]}[](graph)
  out "Ig min":dbl format="%.2e"
  out "Id min":dbl format="%.2e"
  out "Is min":dbl format="%.2e"
  out "Is off":dbl format="%.2e"
  out "Id off":dbl format="%.2e"
  out "Ig off":dbl format="%.2e"
  in  "Integration time (long)":dbl=0.32 min=0.04 max=2.0 step=0.02 format="%.2f"
  in  "Integration time (short)":dbl=0.0019 min=8e-05 max=0.0019 step=8e-05 format="%^.0e"
  in  "Gate: Compliance":dbl=0.001 format="%.8f"
  in  "Drain: Compliance":dbl=0.001 format="%.8f"
  in  "Hard stop pump":bool
  in  "Halt pump":bool
  in  "Interrupt program":bool
  in  "Suffix (script)":string="step_1_up-H2O_initial_script.txt"
  in  "Filename (variable part)":string="step_1_up-H2O_initial_"
  in  "Plot output curve extrema vs time":bool
  in  "Plot transfer curve extrema vs time":bool=TRUE
  in  "Plot sample extrema vs time":bool
  out "I vs time (Bias Stress)":cluster{"Y data in":dbl[], "X data in":dbl[]}[](graph)
  out "Vp1":dbl format="%.2e"
  out "Vp2":dbl format="%.2e"
  in  "Sample I - Probe 4 (Disabled)":u32(ring)=3 items=["SMU1  ", "SMU2  ", "SMU3  ", "SMU4  ", "SMU5  ", "SMU6  ", "VSU1  ", "VSU2  "]
  in  "Sample I - Source/Common":u32(ring) items=["SMU1  ", "SMU2  ", "SMU3  ", "SMU4  ", "SMU5  ", "SMU6  ", "VSU1  ", "VSU2  "]
  in  "Sample I - Probe 3 (Disabled)":u32(ring)=2 items=["SMU1  ", "SMU2  ", "SMU3  ", "SMU4  ", "SMU5  ", "SMU6  ", "VSU1  ", "VSU2  "]
  in  "Sample I - Drain/Gate":u32(ring)=1 items=["SMU1  ", "SMU2  ", "SMU3  ", "SMU4  ", "SMU5  ", "SMU6  ", "VSU1  ", "VSU2  "]
  in  "Sample - Probe 4":u32(ring)=3 items=["SMU1  ", "SMU2  ", "SMU3  ", "SMU4  ", "SMU5  ", "SMU6  ", "VSU1  ", "VSU2  "]
  in  "Sample - Source/Common":u32(ring) items=["SMU1  ", "SMU2  ", "SMU3  ", "SMU4  ", "SMU5  ", "SMU6  ", "VSU1  ", "VSU2  "]
  in  "Sample - Gate":u32(ring)=2 items=["SMU1  ", "SMU2  ", "SMU3  ", "SMU4  ", "SMU5  ", "SMU6  ", "VSU1  ", "VSU2  "]
  in  "Sample - Drain":u32(ring)=1 items=["SMU1  ", "SMU2  ", "SMU3  ", "SMU4  ", "SMU5  ", "SMU6  ", "VSU1  ", "VSU2  "]
  in  "VSU2 Stress - Source/Common":u32(ring) items=["SMU1  ", "SMU2  ", "SMU3  ", "SMU4  ", "SMU5  ", "SMU6  ", "VSU1  "]
  in  "Stress I - Source/Common":u32(ring) items=["SMU1  ", "SMU2  ", "SMU3  ", "SMU4  ", "SMU5  ", "SMU6  ", "VSU1  ", "VSU2  "]
  in  "Stress I - Drain/Gate":u32(ring)=1 items=["SMU1  ", "SMU2  ", "SMU3  ", "SMU4  ", "SMU5  ", "SMU6  ", "VSU1  ", "VSU2  "]
  in  "Stress V - Source/Common":u32(ring) items=["SMU1  ", "SMU2  ", "SMU3  ", "SMU4  ", "SMU5  ", "SMU6  ", "VSU1  ", "VSU2  "]
  in  "Stress V - Gate":u32(ring)=2 items=["SMU1  ", "SMU2  ", "SMU3  ", "SMU4  ", "SMU5  ", "SMU6  ", "VSU1  ", "VSU2  "]
  in  "Stress V - Drain":u32(ring)=1 items=["SMU1  ", "SMU2  ", "SMU3  ", "SMU4  ", "SMU5  ", "SMU6  ", "VSU1  ", "VSU2  "]
  in  "FPP - Source":u32(ring)=6 items=["SMU1  ", "SMU2  ", "SMU3  ", "SMU4  ", "SMU5  ", "SMU6  ", "VSU1  ", "VSU2  "]
  in  "FPP - Probe 2":u32(ring)=3 items=["SMU1  ", "SMU2  ", "SMU3  ", "SMU4  ", "SMU5  ", "SMU6  ", "VSU1  ", "VSU2  "]
  in  "FPP - Probe 1":u32(ring) items=["SMU1  ", "SMU2  ", "SMU3  ", "SMU4  ", "SMU5  ", "SMU6  ", "VSU1  ", "VSU2  "]
  in  "FPP - Gate":u32(ring)=2 items=["SMU1  ", "SMU2  ", "SMU3  ", "SMU4  ", "SMU5  ", "SMU6  ", "VSU1  ", "VSU2  "]
  in  "FPP - Drain":u32(ring)=1 items=["SMU1  ", "SMU2  ", "SMU3  ", "SMU4  ", "SMU5  ", "SMU6  ", "VSU1  ", "VSU2  "]
  in  "Pulsed Stress V - Vextra":u32(ring)=6 items=["SMU1  ", "SMU2  ", "SMU3  ", "SMU4  ", "SMU5  ", "SMU6  ", "VSU1  ", "VSU2  "]
  in  "Pulsed Stress V - Probe 4":u32(ring)=3 items=["SMU1  ", "SMU2  ", "SMU3  ", "SMU4  ", "SMU5  ", "SMU6  ", "VSU1  ", "VSU2  "]
  in  "Pulsed Stress V - Source/Common":u32(ring) items=["SMU1  ", "SMU2  ", "SMU3  ", "SMU4  ", "SMU5  ", "SMU6  ", "VSU1  ", "VSU2  "]
  in  "Pulsed Stress V - Gate":u32(ring)=2 items=["SMU1  ", "SMU2  ", "SMU3  ", "SMU4  ", "SMU5  ", "SMU6  ", "VSU1  ", "VSU2  "]
  in  "Pulsed Stress V - Drain":u32(ring)=1 items=["SMU1  ", "SMU2  ", "SMU3  ", "SMU4  ", "SMU5  ", "SMU6  ", "VSU1  ", "VSU2  "]
  in  "Transfer/Output - Probe 4":u32(ring)=3 items=["SMU1  ", "SMU2  ", "SMU3  ", "SMU4  ", "SMU5  ", "SMU6  ", "VSU1  ", "VSU2  "]
  in  "Transfer/Output - Source/Common":u32(ring) items=["SMU1  ", "SMU2  ", "SMU3  ", "SMU4  ", "SMU5  ", "SMU6  ", "VSU1  ", "VSU2  "]
  in  "Transfer/Output - Gate":u32(ring)=2 items=["SMU1  ", "SMU2  ", "SMU3  ", "SMU4  ", "SMU5  ", "SMU6  ", "VSU1  ", "VSU2  "]
  in  "Transfer/Output - Drain":u32(ring)=1 items=["SMU1  ", "SMU2  ", "SMU3  ", "SMU4  ", "SMU5  ", "SMU6  ", "VSU1  ", "VSU2  "]
  in  "Gate Range\nmode":u16(ring) items=["Auto", "Limited", "Fixed"]
  in  "Gate Range":u8(slide)=3 max=11 scale=0.0..11.0
  in  "Source/Drain\nRange mode":u16(ring) items=["Auto", "Limited", "Fixed"]
  in  "Source/Drain Range":u8(slide)=3 max=11 scale=0.0..11.0
  in  "Panel Controls":T1={"Emergency Stop"=refnum, "TransGraph Max"=1e-05, "Text/Graph (text=false)"=TRUE} {"TransGraph Max" format="%.2e"}
  in  "Panel Controls 2":T2={"Emergency Stop"=refnum, "TransGraph Max"=1e-05, "Text/Graph (text=false)"=TRUE, "TransGraph Min"=1e-11} {"TransGraph Min" format="%.2e"; "TransGraph Max" format="%.2e"}
  in  "Probe 4":cluster{"on/off":bool, "Voltage":dbl} {"Voltage" min=-100.0 max=100.0 format="%.2f"}
  in  "Full Reset":bool
  in  "Standby":T3
  out "error out":errorcluster
  in  "Delay before read (ms)":u32=1000
  in  "byte count":u32=64
  in  "Serial End Mode for Reads":u16(ring)=2 items=["None", "LastBit", "TermChar"]
  in  "Timeout (ms)":u32=10000
  in  "Enable Termination\nChar (T)":bool=TRUE
  in  "Termination char\n(0xA = '\\n' = LF)\n(0xD = '\\r' = CR)":u8=13 format="%.0x"
  in  "flow control":u16(ring) items=["None"=0, "XON/XOFF"=1, "RTS/CTS"=2, "DTR/DSR"=4]
  in  "stop bits":u16(ring)=10 items=["1.0"=10, "1.5"=15, "2.0"=20]
  in  "parity":u16(ring) items=["None", "Odd", "Even", "Mark", "Space"]
  in  "data bits":u16=8 min=5 max=8 step=1
  in  "VISA resource name":refnum<visa-resource-name>="COM6"
  in  "baud rate":u32=9600
  out "Timings Indicator":T4 {"integration time" scale=0.0..2.0}
  in  "Timings (overwritten by the Front Panel)":T5={"integration time"=0, "Short/Long integration time"=0.00064, "hold time (sec)"=0.0, "delay time (sec)"=0.0, "Step Time (0 disables)"=0.0, "sweep method"=0, "Pulse period"=0.005, "Base voltage"=0.0, "Pulse width"=0.0005} {"Pulse width" min=0.0005 max=0.1 step=0.0001 format="%.4f"; "Base voltage" format="%^.4e"; "Pulse period" min=0.005 max=1.0 step=0.0001 format="%.4f"; "sweep method" items=["Continuous", "Pulsed"]; "Step Time (0 disables)" format="%.2f"; "delay time (sec)" format="%.4f"; "hold time (sec)" format="%.4f"; "Short/Long integration time" format="%^.0e"; "integration time" scale=0.0..2.0}
  out "Probe 4 Indicator":cluster{"on/off":bool, "Voltage":dbl} {"Voltage" min=-100.0 max=100.0 format="%.2f"}
  in  "VISA resource name in":refnum<visa-resource-name>="GPIB0::14::INSTR"
  in  "Gate":T6={"Gate Start"=0.0, "Gate Stop"=2.0, "Gate Step (linear only)"=1.0, "Gate Compliance"=0.0001, "Gate PComp"=0.0, "Range mode"=0, "Range"=6} {"Range" max=11 scale=0.0..11.0; "Range mode" items=["Auto", "Limited", "Fixed"]; "Gate PComp" format="%^.2e"; "Gate Compliance" format="%^.2e"; "Gate Step (linear only)" format="%^.4e"; "Gate Stop" format="%^.4e"; "Gate Start" format="%^.4e"}
  in  "Drain 2":T7={"Drain Start"=0.0, "Drain Stop"=2.0, "Drain Compliance"=0.0001, "Drain Step"=1.0, "Drain PComp"=0.0, "Range mode"=0, "Range"=6} {"Range" max=11 scale=0.0..11.0; "Range mode" items=["Auto", "Limited", "Fixed"]; "Drain PComp" format="%^.2e"; "Drain Step" format="%^.4e"; "Drain Compliance" format="%^.2e"; "Drain Stop" format="%^.4e"; "Drain Start" format="%^.4e"}
  # "Syntax:\nitime [s|m|l] time(sec): [s|m|l] determines the integration time setting (small|medium|long) and time sets the value.\nNOTE: The value of the integration time has to be within the range allowed by its category (s|m|l), otherwise, the closest value will be used. (e.g. if the category is set to short but the time value is very long, the actual value used will be the maximum short integration time.\nIntegration times:\n    Short: Default: 640 us. Range: 8E-5 - 1.92E-3 seconds.\n    Medium: Fixed at 1 NPL cycle (0.02 seconds).\n    Long: Default: 16 NPL cycles (0.32 seconds). Range: 2-100 NPL cycles (0.04 seconds - 2 seconds).\ngaterangemode [a|l|f]\ndrainrangemode [a|l|f]\npulsed [on|off] PulsePeriod(sec) PulseBaseVoltage PulseONWidth(sec)\nstandby [on l off]\nwait NumMilliseconds\nwait-min NumMinutes\n# texthere = comment\nProbe4 [ON|OFF] Voltage\ntransfer [s|d] VgStart VgStop VgStep VdStart VdStop VdStep\noutput [s|d] VgStart VgStop VgStep VdStart VdStop VdStep\nsample Vg Vd NumSamples Time(s) SampleInterval(s)\nsamplei Idg NumSamples Time(s) SampleInterval(s) VDGcompliance\n100 samples is approximately 13 seconds with medium integration\n# If in doubt use SampleInterval(s) = 0.004\n    NOTE: When doing bias stress measurements, it is best to set the Time Units to \"Seconds\", as the \"sample\" command has been configured to give the output to seconds.\nstressV VG VD IGcompliance IDcompliance Duration(sec)\nstressI IDG VDGcompliance Duration(sec)\nvsu2pulse Bias Duration(s)\npulsedstressV [s|d] VEstop VgON VgOFF Period(s) PulseONwidth(s) Vd\nsample-fpp Vg Vd NumSamples Time\nresample-fpp Vg Vd\ntransfer-fpp [s|d] VgStart VgStop VgStep VdStart VdStop VdStep\noutput-fpp [s|d] VgStart VgStop VgStep VdStart VdStop VdStep\nserial SerialPortCommand\npump SerialPortCommand for the SPM pump\n\nSPM Pump Syntax (<x>: pump number, use 1 if only one pump):\nif the command syntax contains [R], then append the letter R to the command\n/<x>Q: query (a query command should follow each command)\n/<x>Z[R] or /<x>Y[R]: initialize pump\n/<x>N<n>[R] (<n>=0,1): <0> (<1>) microstep 0.01 mm (0.00125 mm) resolution\n/<x>I<n> (<n>=0-6): turn to port number n (clockwise)\n/<x>O<n> (<n>=0-6): turn to port number n (counterclockwise)\n/<x>X: Re-execute last command string\n/<x>G<n>[R] (<n>=0-60000): repeat command sequence (default: 0, 0=loop forever)\n/<x>g: Mark the start of a repeat sequence (max = 10)\n/<x>M<n>[R] (<n>=0-86400000): delay command execution by n milliseconds\n/<x>H: Halt; Pause the sequence after finishing the current move\n/<x>T: Hardstop; Interrupt the current move and suppress it from the sequence\n/<x>A<n>[R] (<n>=0-3000 with N=0, 0-24000 with N=1): absolute position\n/<x>P<n>[R] (<n>=0-3000 with N=0, 0-24000 with N=1): relative pickup\n/<x>D<n>[R] (<n>=0-3000 with N=0, 0-24000 with N=1): relative dispense\n/<x>V<n>[R] (<n>=1-1600 default: 150): set peak speed (pulses/sec)\nNOTE: The lowest speed limit is 1 pulse/sec, not 5, as the manual states.\n/<x>S<n>[R] (<n>=10-40 default: 22): set speed (NOT in pulses/sec, look in manual)\nNOTE: When controlled with absolute position, one does not need to pay special attention to the syringe that is mounted on the pump.\nWithdraw from lower stage (ports 3, 5), dispense from higher stage (ports 2, 4, 6).\nConnect Port 1 to waste."
  # "Time"
  # "1\n2\n3\n4\n5\n6\n7\n8\n9\n10\n11\n12\n13\n14\n15\n16\n17\n18\n19\n20"
  # "Serial port settings"
  # "SMUs"
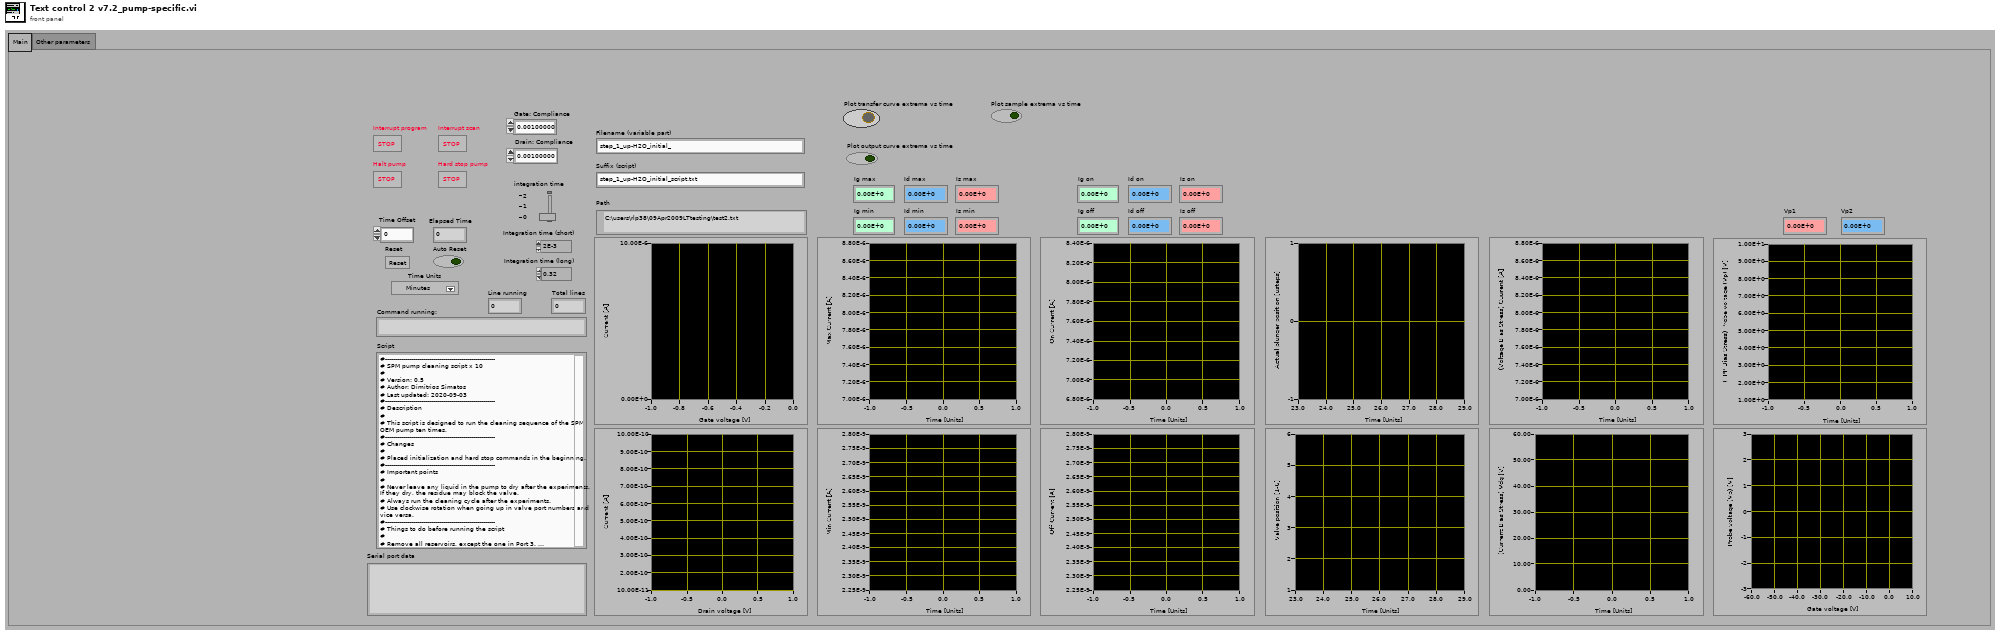
[diagram p1: front panel]
types:
  T1 = cluster{"Emergency Stop":refnum<vi>, "TransGraph Max":dbl, "Text/Graph (text=false)":bool}
  T2 = cluster{"Emergency Stop":refnum<vi>, "TransGraph Max":dbl, "Text/Graph (text=false)":bool, "TransGraph Min":dbl}
  T3 = cluster{"Gate Standby":bool, "Drain Standby":bool}
  T4 = cluster{"Short/Long integration time":dbl, "hold time (sec)":dbl, "delay time (sec)":dbl, "Step Time (0 disables)":dbl, "sweep method":u16, "Pulse period":dbl, "Base voltage":dbl, "Pulse width":dbl, "integration time":u32}
  T5 = cluster{"integration time":u32, "Short/Long integration time":dbl, "hold time (sec)":dbl, "delay time (sec)":dbl, "Step Time (0 disables)":dbl, "sweep method":u16, "Pulse period":dbl, "Base voltage":dbl, "Pulse width":dbl}
  T6 = cluster{"Gate Start":dbl, "Gate Stop":dbl, "Gate Step (linear only)":dbl, "Gate Compliance":dbl, "Gate PComp":dbl, "Range mode":u16, "Range":u8}
  T7 = cluster{"Drain Start":dbl, "Drain Stop":dbl, "Drain Compliance":dbl, "Drain Step":dbl, "Drain PComp":dbl, "Range mode":u16, "Range":u8}
  T8 = enum16{"open", "replace", "create", "open or create", "replace or create", "replace or create with confirmation"}
  T9 = cluster{"V2 Start":dbl, "V2 Step":dbl, "Number of points":i32}
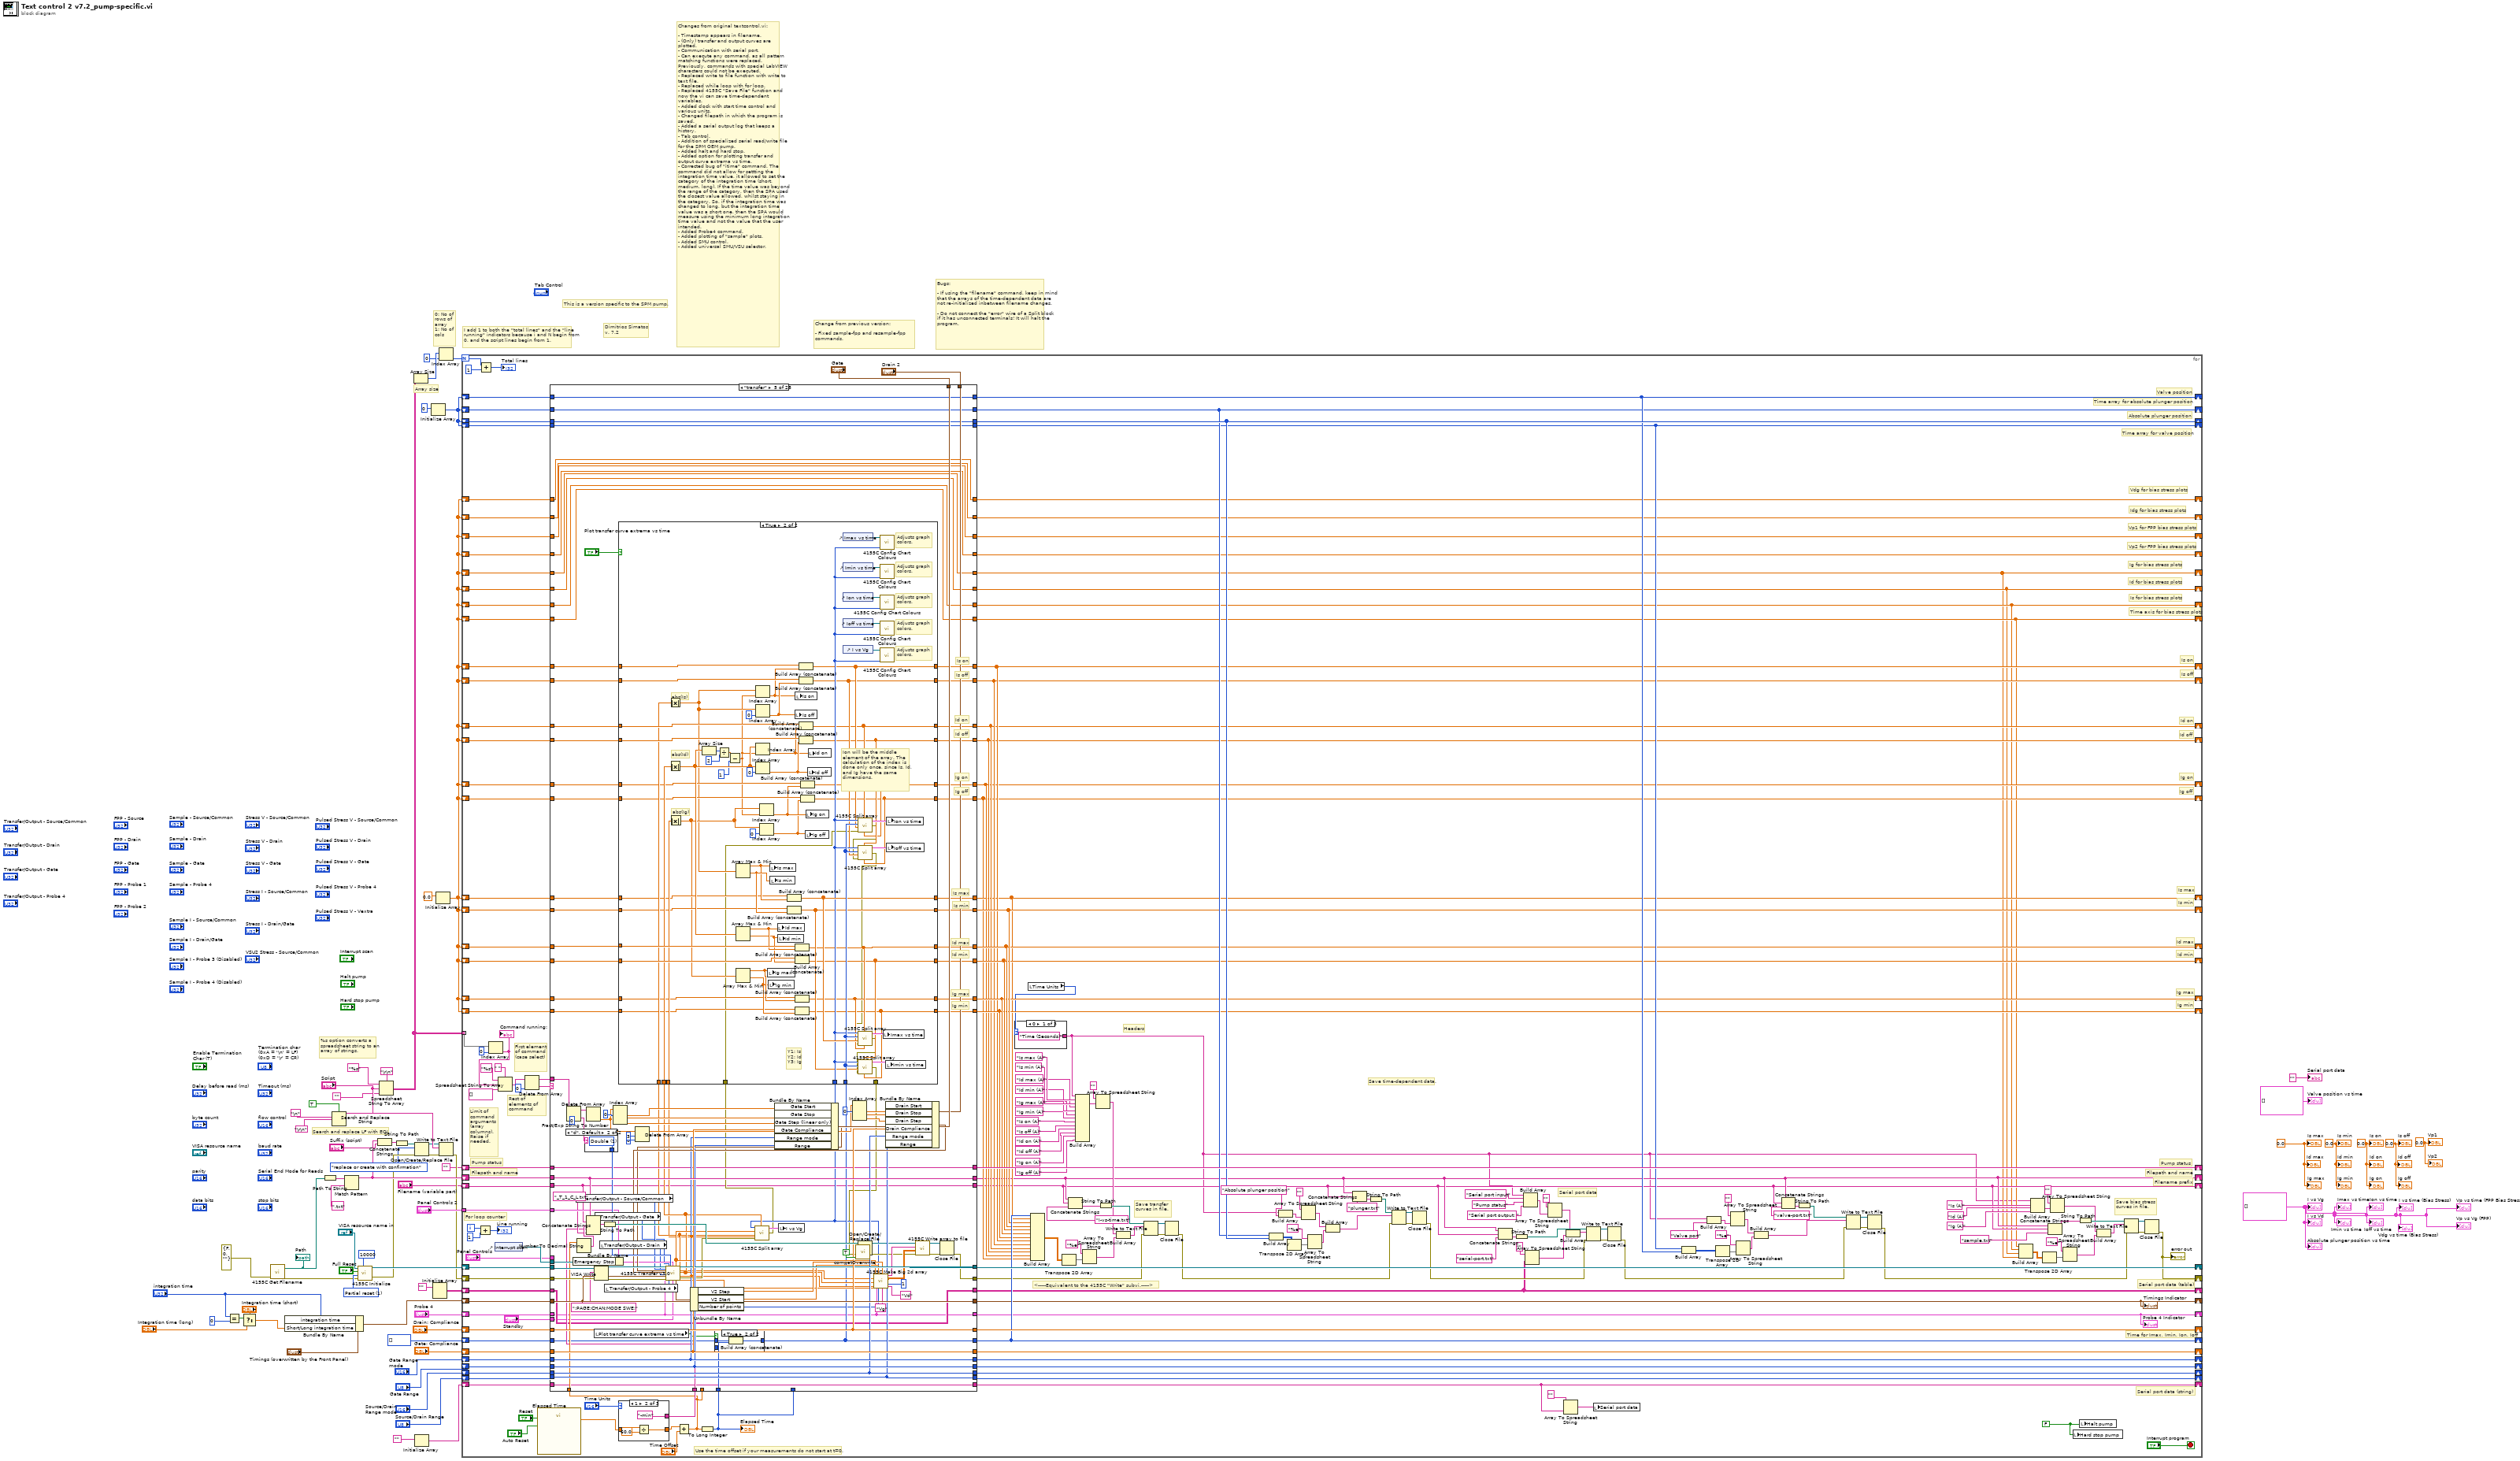
[diagram p0: block diagram]
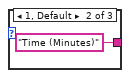
[diagram p2: hidden frame]
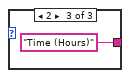
[diagram p3: hidden frame]
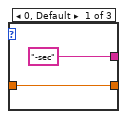
[diagram p4: hidden frame]
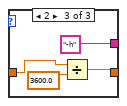
[diagram p5: hidden frame]
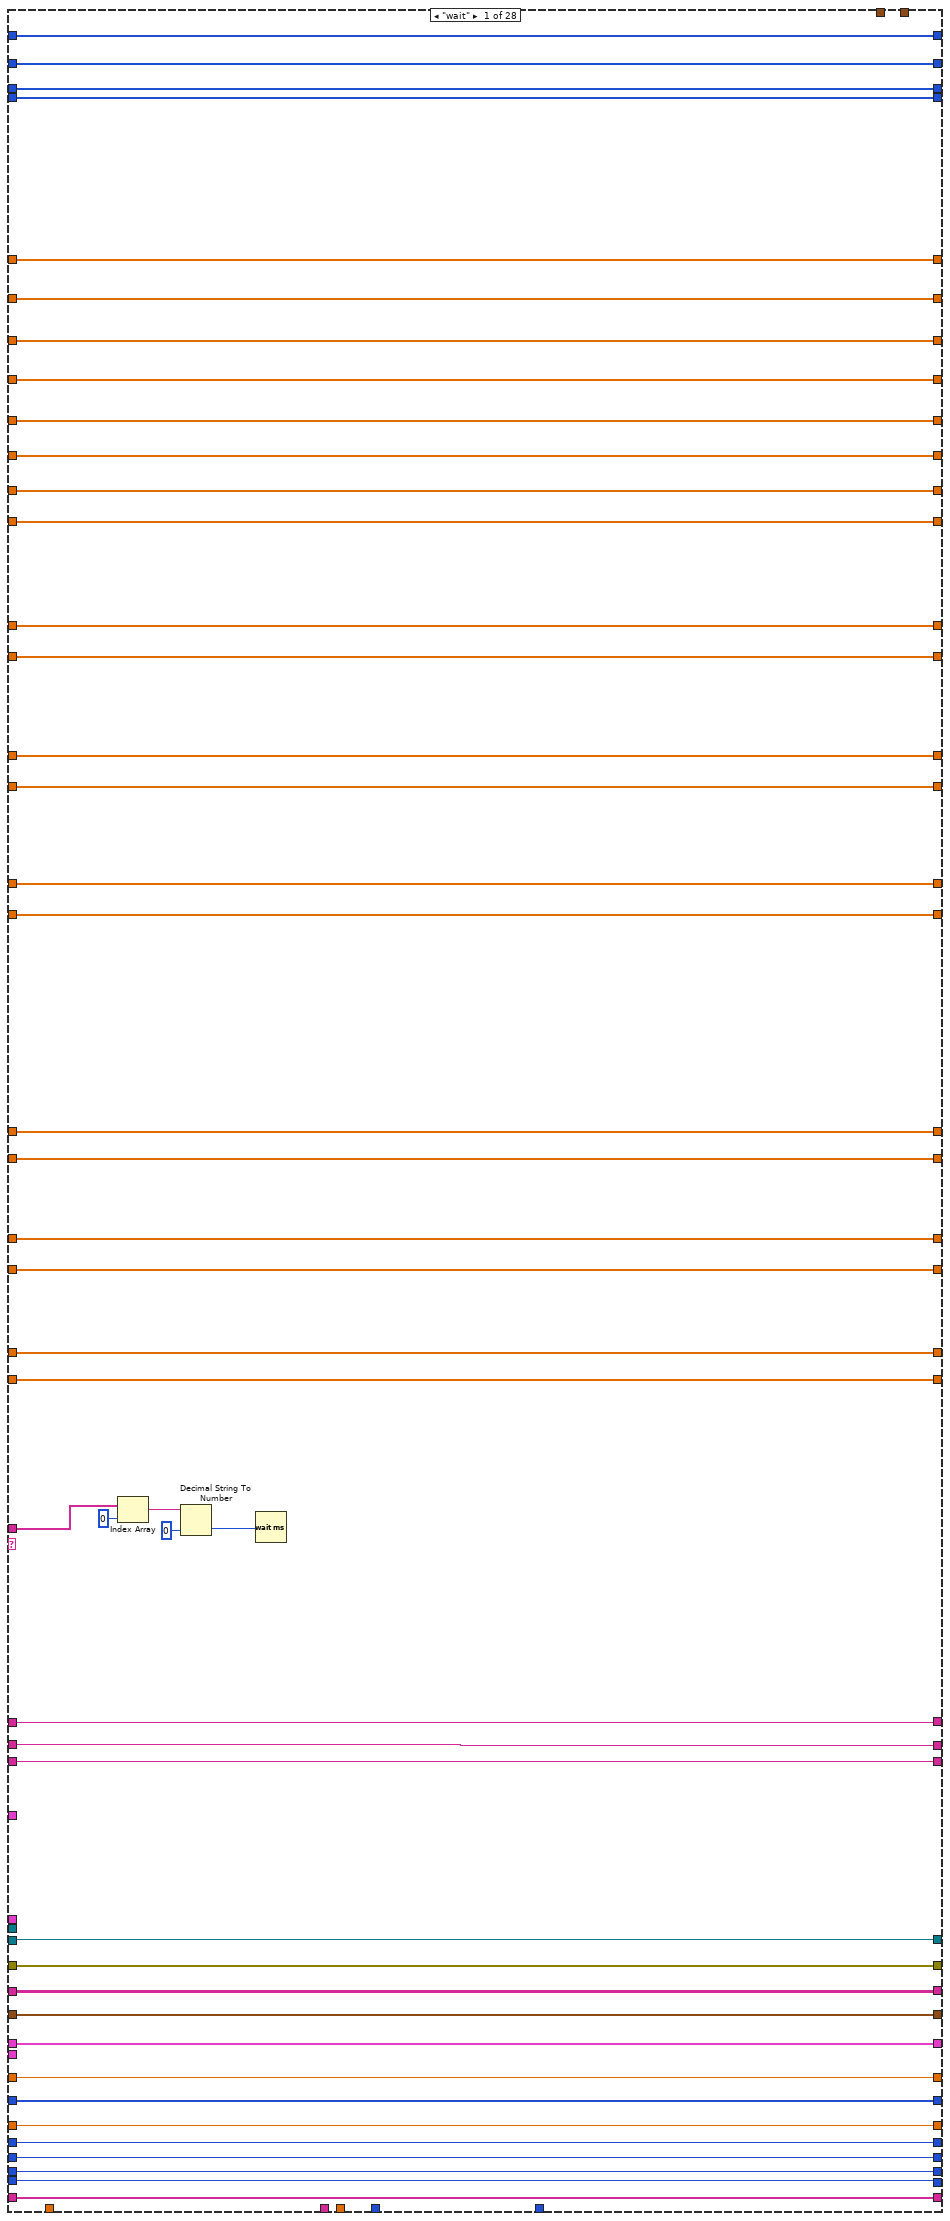
[diagram p6: hidden frame]
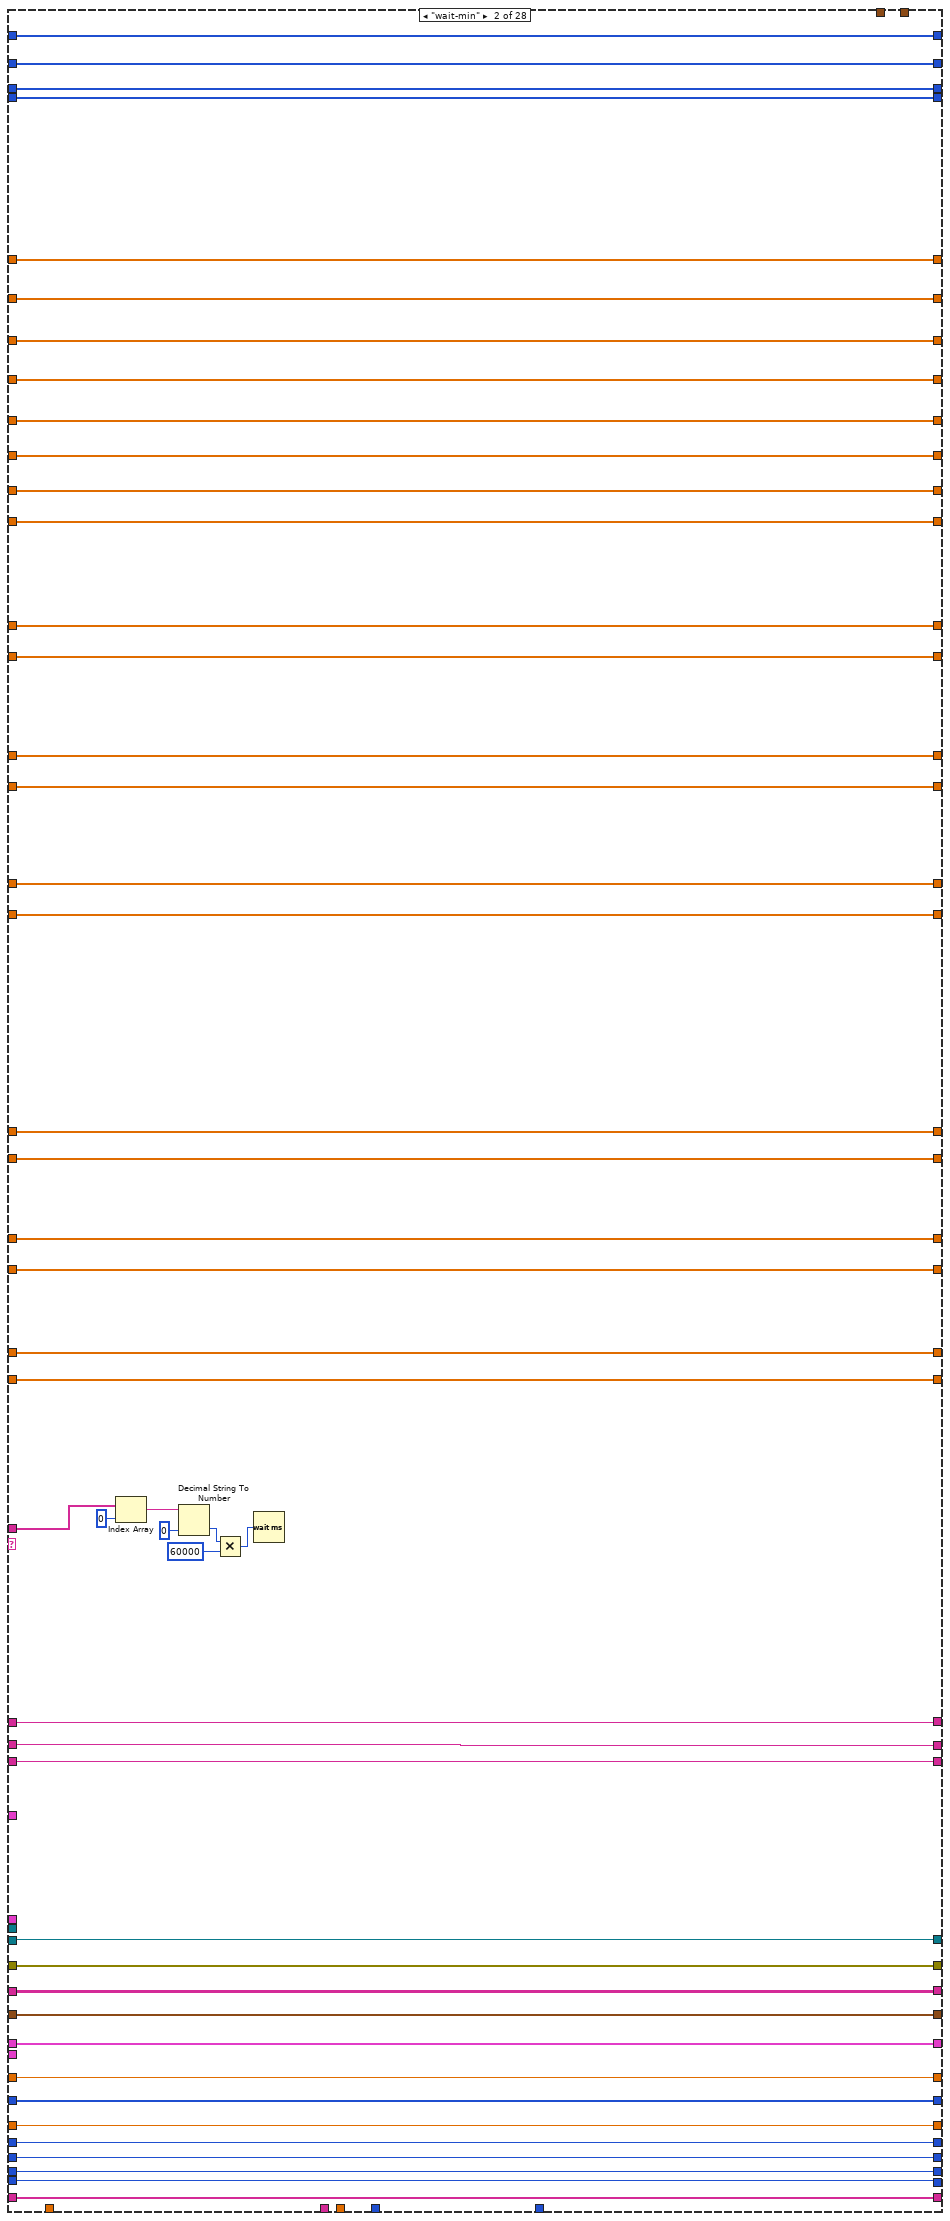
[diagram p7: hidden frame]
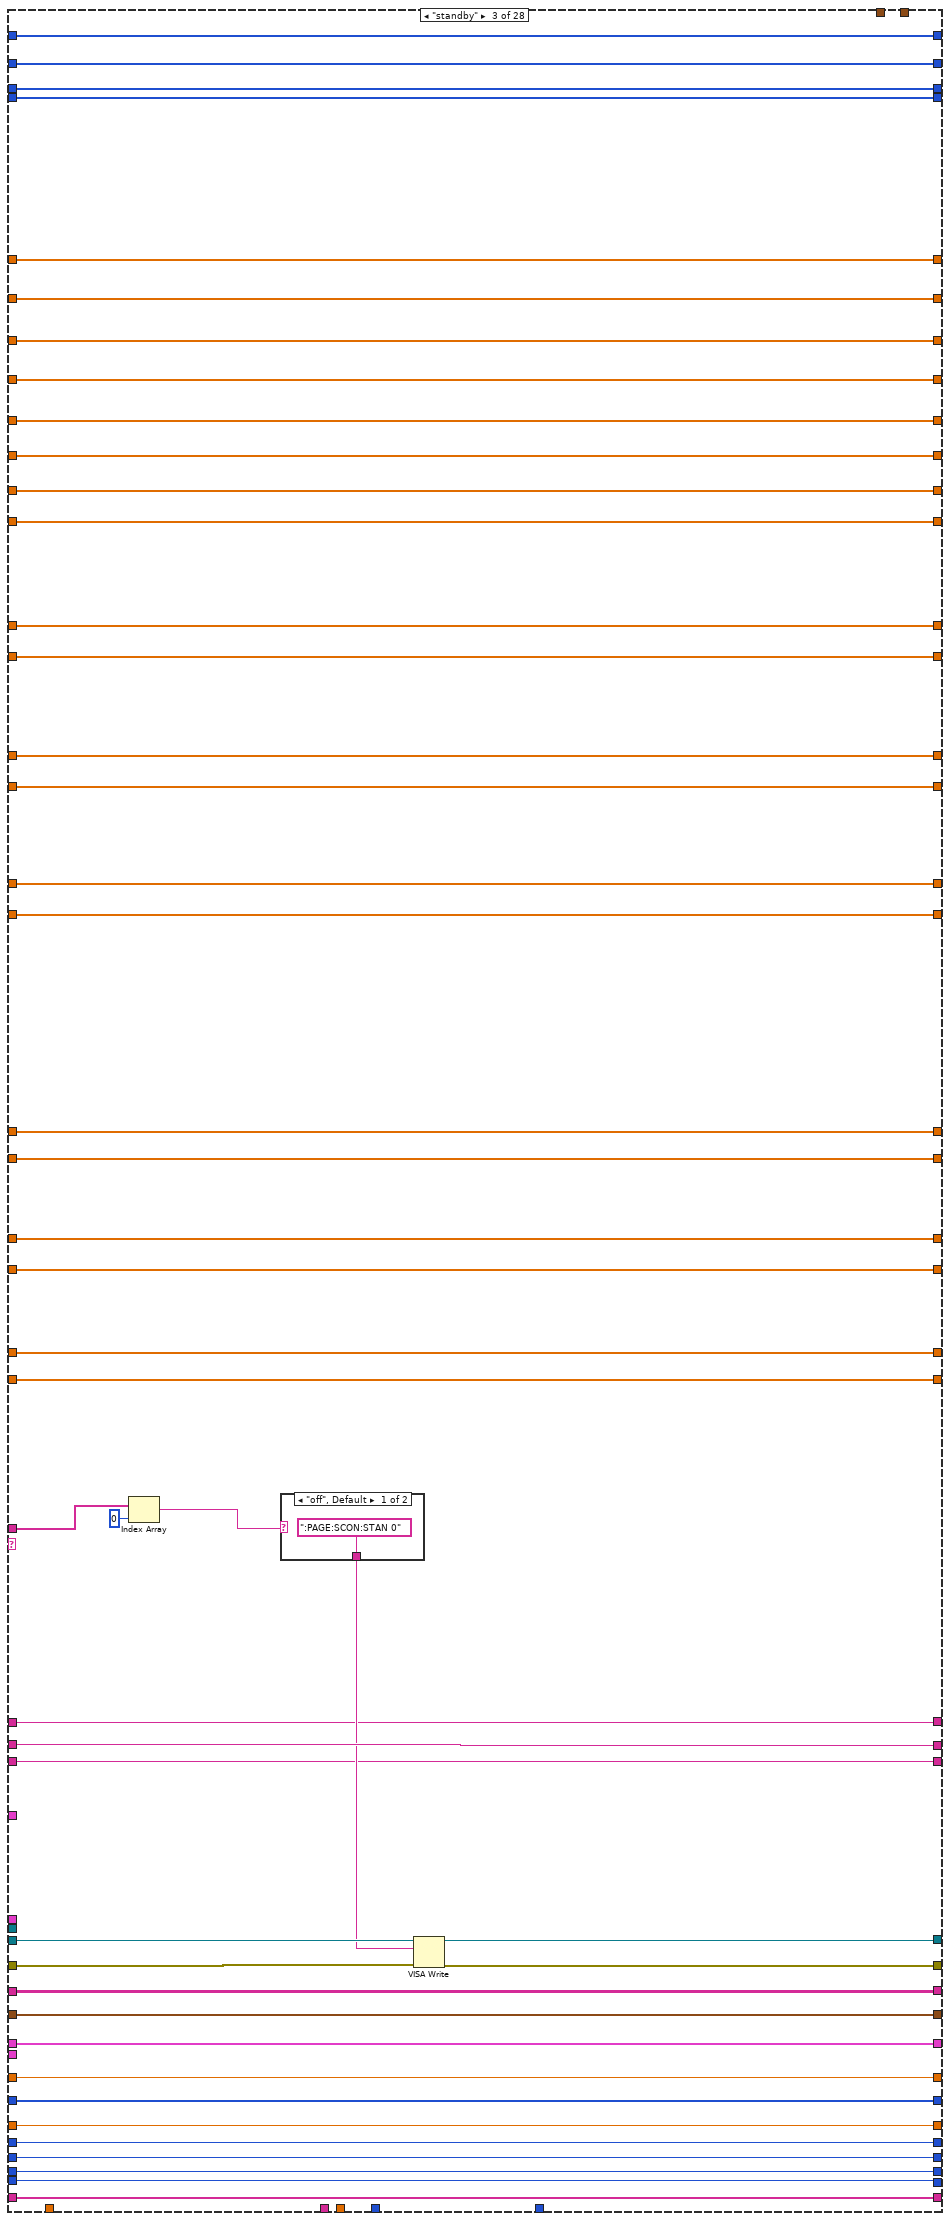
[diagram p8: hidden frame]
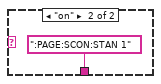
[diagram p9: hidden frame]
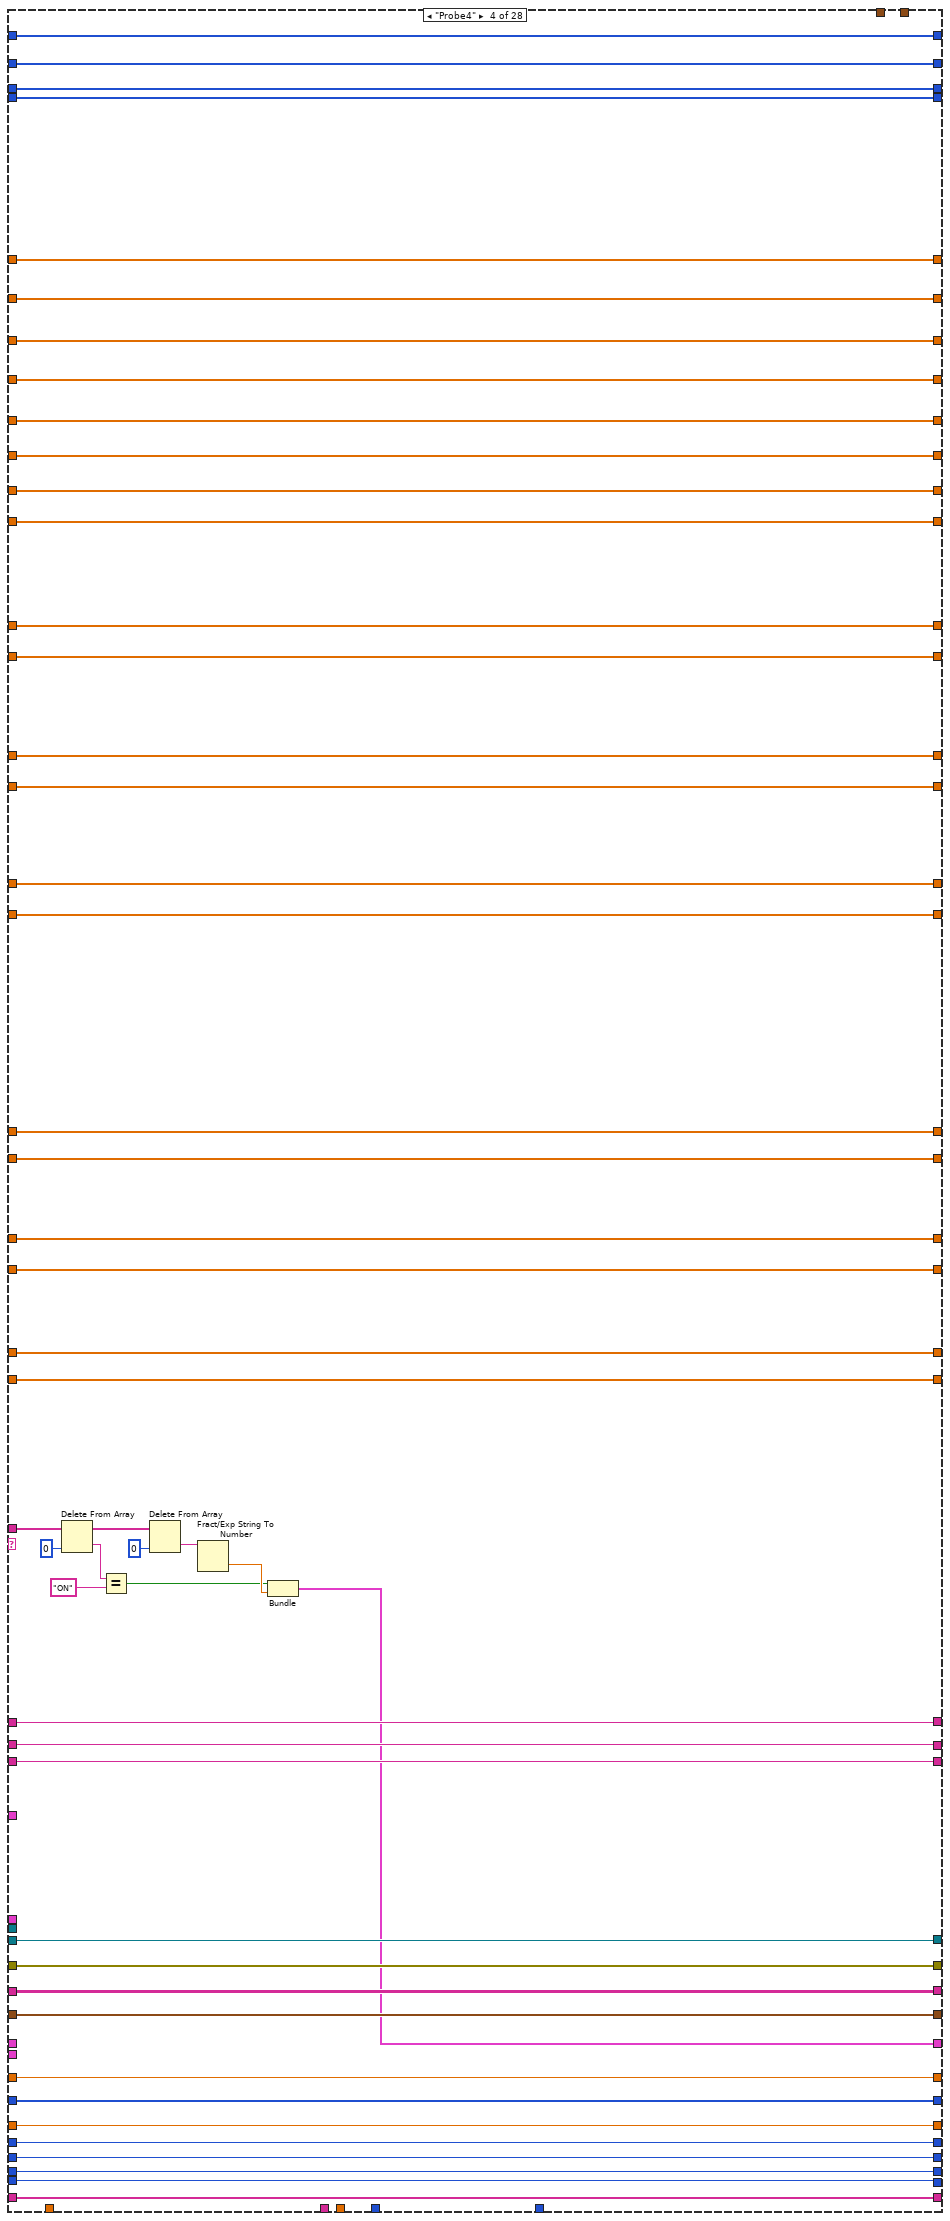
[diagram p10: hidden frame]
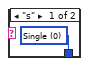
[diagram p13: hidden frame]
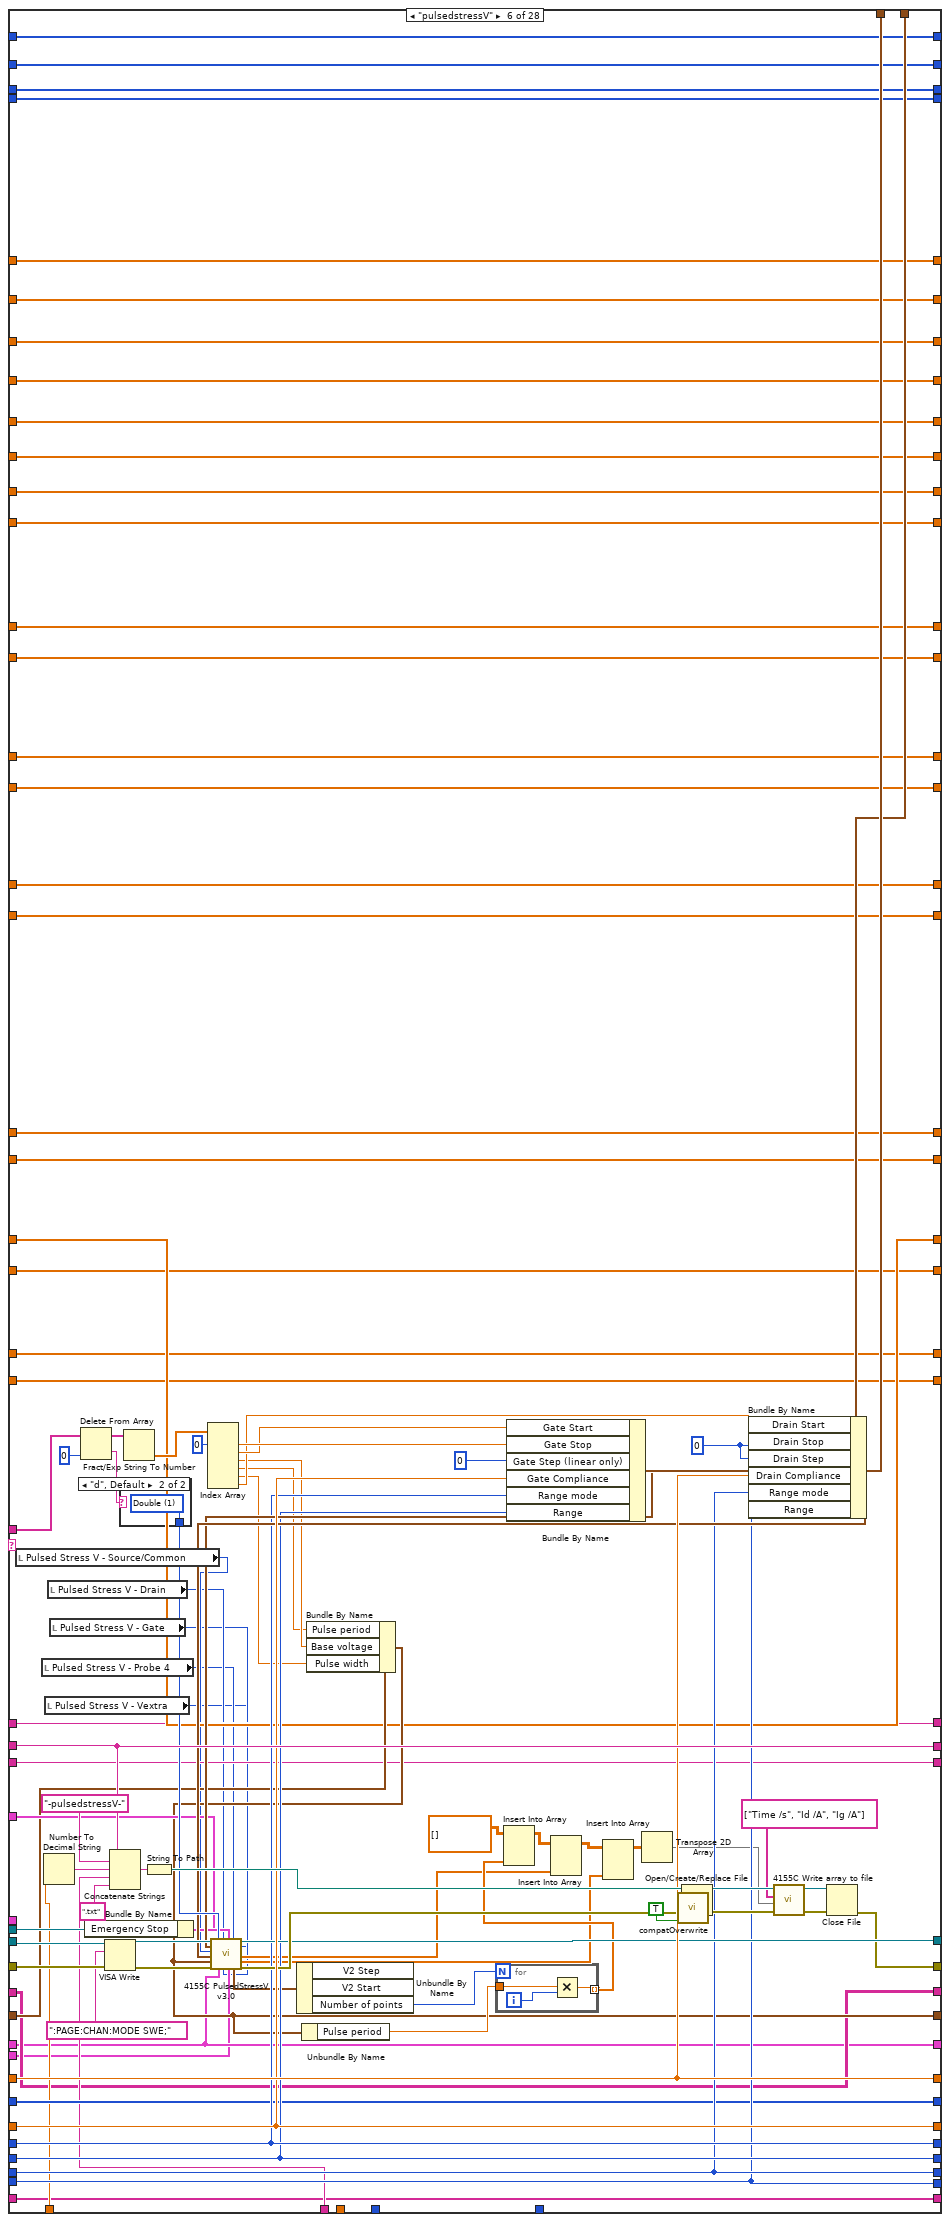
[diagram p14: hidden frame]
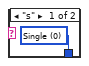
[diagram p15: hidden frame]
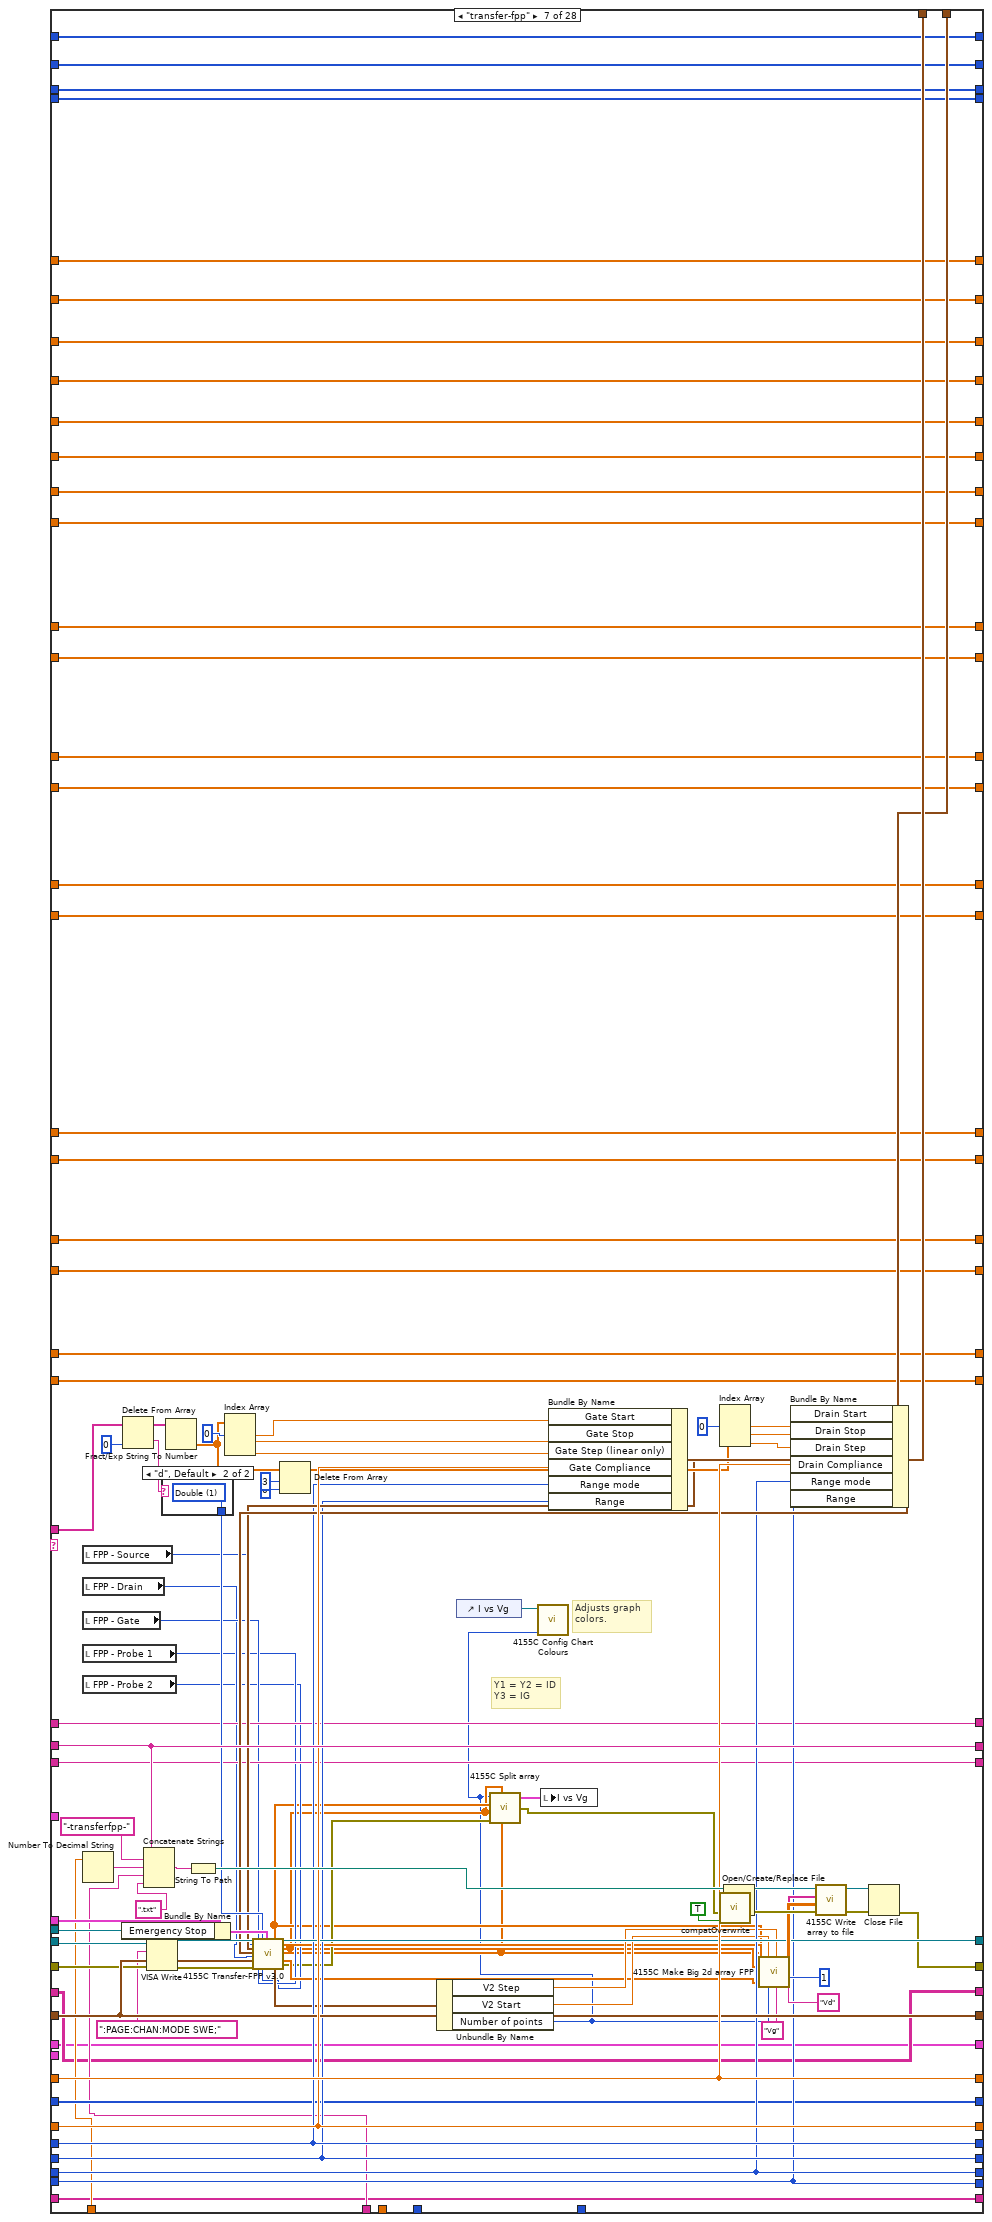
[diagram p16: hidden frame]
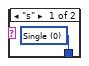
[diagram p17: hidden frame]
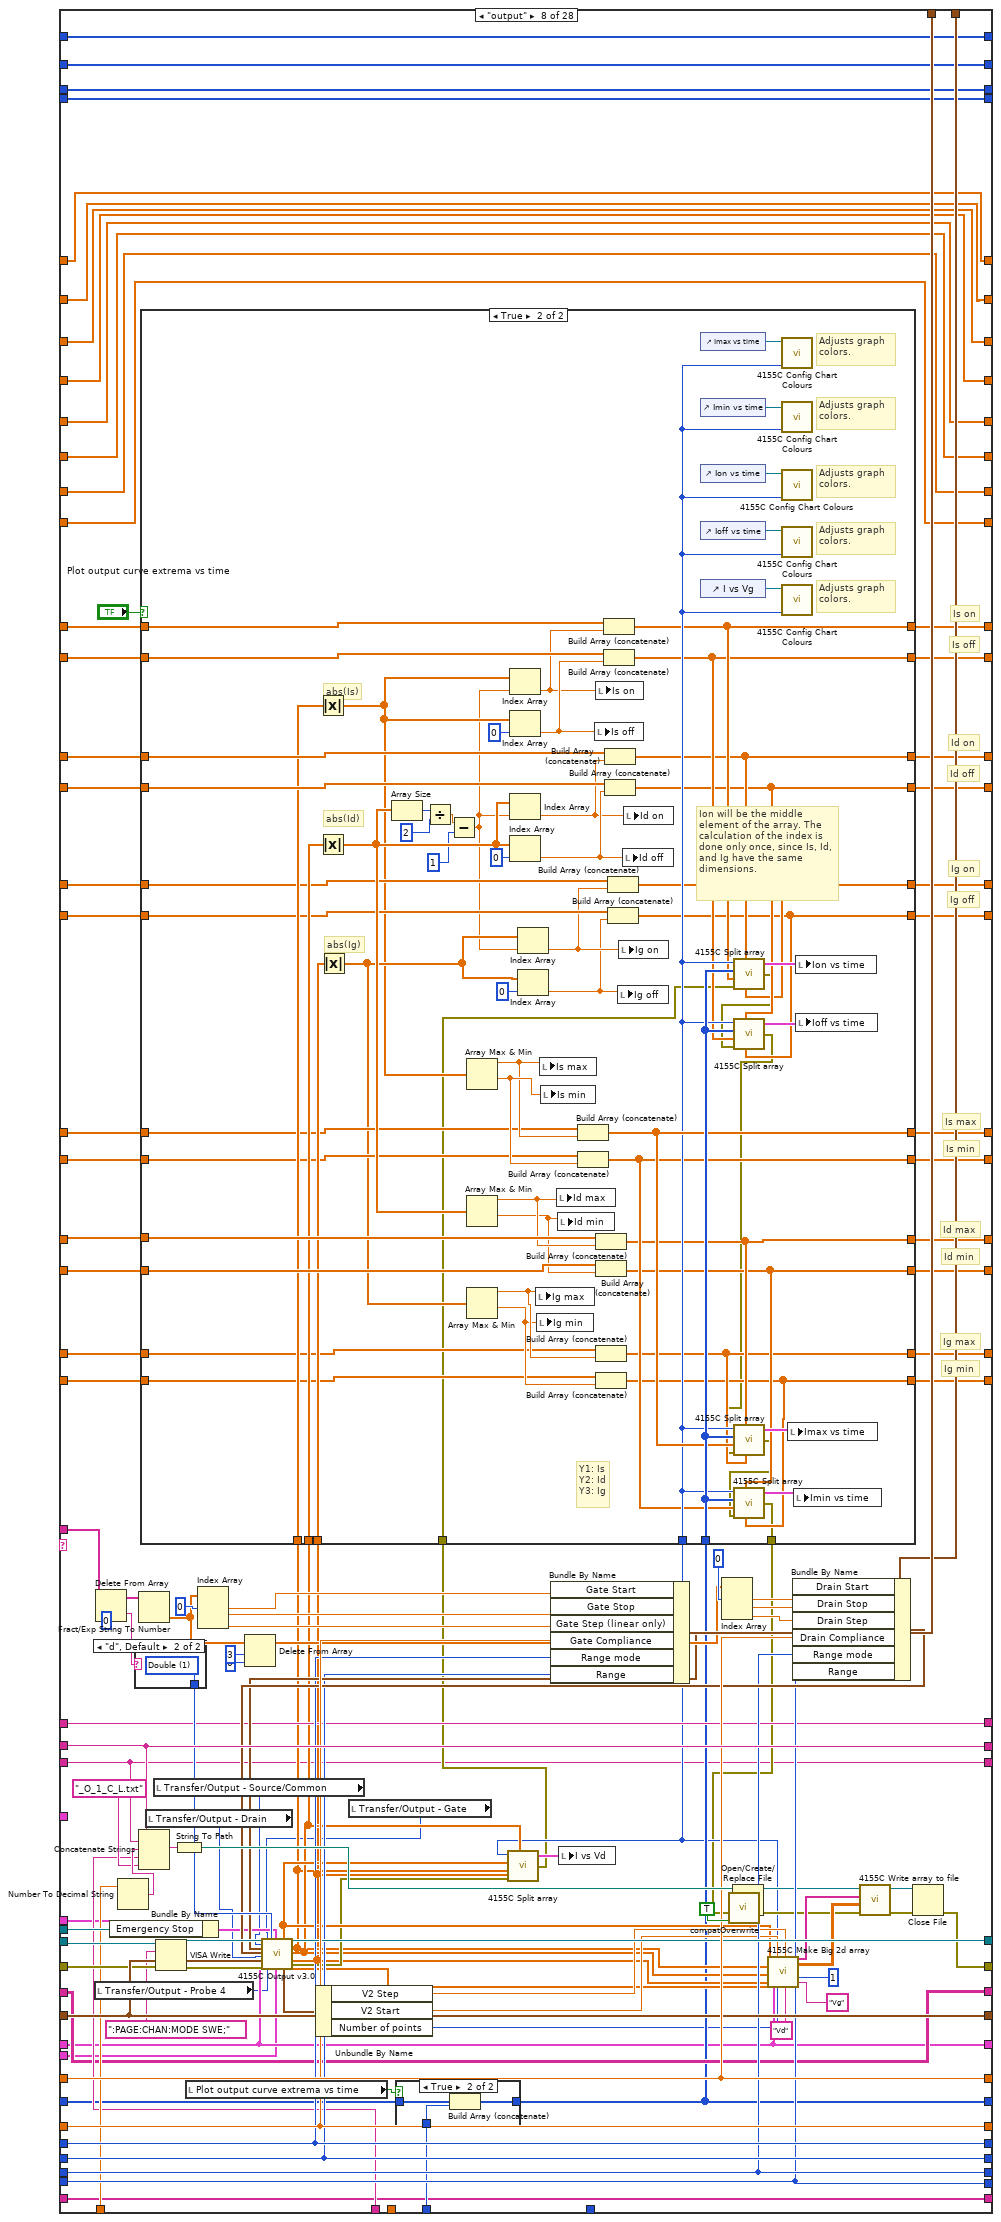
[diagram p18: hidden frame]
diagram:
  w3 = 0.0 ("Is off")
  w2 = cluster{"Y data in":dbl[], "X data in":dbl[]}[] [] ("I vs Vg")
  w12 = 0.0 ("Is off")
  w13 = 0.0 ("Is on")
  w14 = 0.0 ("Is min")
  w15 = 0.0 ("Is max")
  w61 = u16 1 items=["Reset All", "Partial reset"] ("Type of reset")
  # "Change from previous version:\n\n- Fixed sample-fpp and resample-fpp commands."
  # "This is a version specific to the SPM pump."
  # "I add 1 to both the \"total lines\" and the \"line running\" indicators because i and N begin from 0, and the script lines begin from 1."
  # "Bugs:\n\n- If using the \"filename\" command, keep in mind that the arrays of the time-dependent data are not re-initialized inbetween filename changes. \n\n- Do not connect the \"error\" wire of a Split block if it has unconnected terminals! It will halt the program."
  # "Array size"
  # "%s option converts a spreadsheet string to an array of strings."
  # "0: No of rows of array\n1: No of cols"
  # "Dimitrios Simatos\nv. 7.2"
  # "Changes from original textcontrol.vi:\n\n- Timestamp appears in filename.\n- (Only) transfer and output curves are plotted.\n- Communication with serial port.\n- Can execute any command, as all pattern matching functions were replaced. Previously, commands with special LabVIEW characters could not be executed.\n- Replaced write to file function with write to text file.\n- Replaced while loop with for loop.\n- Replaced 4155C \"Save File\" function and now the vi can save time-dependent variables.\n- Added clock with start time control and various units.\n- Changed filepath in which the program is saved.\n- Added a serial output log that keeps a history.\n- Tab control.\n- Addition of specialized serial read/write file for the SPM OEM pump.\n- Added halt and hard stop.\n- Added option for plotting transfer and output curve extrema vs time.\n- Corrected bug of \"itime\" command. The command did not allow for settting the integration time value, it allowed to set the category of the integration time (short, medium, long). If the time value was beyond the range of the category, then the SPA used the closest value allowed, whilst staying in the category. So, if the integration time was changed to long, but the integration time value was a short one, then the SPA would measure using the minimum long integration time value and not the value that the user intended.\n- Added Probe4 command.\n- Added plotting of \"sample\" plots.\n- Added SMU control.\n- Added universal SMU/VSU selector."
  # "Search and replace LF with EOL"
  n1 = Equal?(x="integration time", y=u32 0) -> (x = y?=w62:bool)
  n2 = Select(t="Integration time (short)", s=w62, f="Integration time (long)") -> (s? t:f=w16:dbl)
  n3 = call "4155C Get Filename.vi"("error in (no error)"=errorcluster {"status"=FALSE, "code"=0, "source"=""}) -> ("error out"=w56:errorcluster, "path"=w31:path)  [unwired: 2 in, 1 out]
  "Path" <- w31
  n4 = Bundle By Name(cluster="Timings (overwritten by the Front Panel)", "integration time"="integration time", "Short/Long integration time"=w16) -> (w54:T5)
  n5 = Path To String(path=w31) -> (string=w32:string)
  n6 = Search and Replace String(replace all?=TRUE ("replace all? (F)"), input string="Script", search string="\n", replace string="\r\n") -> (result string=w44:string)  [unwired: 4 in, 3 out]
  n7 = Match Pattern(string=w32, regular expression=".txt") -> (before substring=w28:string)  [unwired: 1 in, 3 out]
  n8 = call "4155C Initialise.vi"("VISA resource name in"="VISA resource name in", "Reset"="Full Reset", "Type of reset"=w61, "error in (no error)"=w56, "VISA Timeout Value"=u32 10000) -> ("VISA Resource Name out"=w55:refnum<visa-resource-name>, "error out"=w5:errorcluster)
  n9 = Concatenate Strings(w28, "Suffix (script)") -> (w27:string)
  n10 = Spreadsheet String To Array(delimiter (Tab)="\r\n", format string="%s", spreadsheet string="Script", array type (2D Dbl)="") -> (array=w35:string[][])
  n11 = String To Path(string=w27) -> (path=w8:path)
  n12 = Array Size(array=w35) -> (size(s)=w39:i32[])
  n13 = Initialize Array("") -> (w20:string[])  [unwired: 1 in]
  n14 = Open/Create/Replace File(file path (use dialog)=w8, error in=w5, operation (0:open)=T8."replace or create with confirmation") -> (refnum out=w7:refnum<file>, error out=w6:errorcluster)  [unwired: 3 in, 1 out]
  n15 = Initialize Array(0 ("element")) -> (w22:i32[])  [unwired: 1 in]
  n16 = Initialize Array("") -> (w18:string[][])  [unwired: 2 in]
  n17 = Initialize Array(0.0 ("element")) -> (w1:dbl[])  [unwired: 1 in]
  n18 = Index Array(array=w39, index=0) -> (element=w37:i32)
  n19 = Write to Text File(file (use dialog)=w7, text=w44, error in=w6) -> (error out=w26:errorcluster)  [unwired: 1 in, 2 out]
  n20 = for {
    N: w37 -> [w215]
    shift-left: "Source/Drain Range" -> [w255]
    shift-right: [w251] -> _
    shift-left: "Source/Drain\nRange mode" -> [w256]
    shift-right: [w252] -> _
    shift-left: "Gate Range" -> [w257]
    shift-right: [w253] -> _
    shift-left: "Gate Range\nmode" -> [w258]
    shift-right: [w254] -> _
    shift-left: "Gate: Compliance" -> [w266]
    shift-right: [w263] -> _
    shift-left: "Drain: Compliance" -> [w267]
    shift-right: [w264] -> _
    shift-left: w54 -> [w268]
    shift-right: [w77] -> _
    shift-left: w26 -> [w269]
    shift-right: [w76] -> _
    shift-left: w55 -> [w270]
    shift-right: [w265] -> _
    shift-left: w28 -> [w271]
    shift-right: [w86] -> _
    tunnel: "Panel Controls 2" -> [w249]
    shift-right: [w127] -> _
    shift-left: w1 -> [w248]
    shift-right: [w185] -> _
    shift-left: i32[] [] -> [w244]
    tunnel: w35 -> [w243] mode=indexing
    shift-right: [w126] -> _
    shift-left: w1 -> [w220]
    shift-right: [w158] -> _
    shift-left: w20 -> [w207]
    shift-right: [w186] -> _
    shift-left: w22 -> [w202]
    shift-right: [w168] -> _
    shift-left: w22 -> [w201]
    shift-right: [w200] -> _
    shift-left: "" -> [w199]
    shift-right: [w163] -> _
    shift-left: w22 -> [w183]
    shift-right: [w162] -> _
    shift-left: w22 -> [w167]
    shift-right: [w159] -> _
    shift-left: w18 -> [w161]
    shift-right: [w120] -> _
    shift-left: w1 -> [w148]
    shift-right: [w121] -> _
    shift-left: w1 -> [w147]
    shift-right: [w125] -> _
    shift-left: w1 -> [w136]
    shift-right: [w124] -> _
    shift-left: w1 -> [w135]
    shift-right: [w118] -> _
    shift-left: w1 -> [w134]
    shift-right: [w128] -> _
    shift-left: w1 -> [w133]
    shift-right: [w119] -> _
    shift-left: w1 -> [w132]
    shift-right: [w117] -> _
    shift-left: w1 -> [w131]
    shift-right: [w123] -> _
    shift-left: w1 -> [w130]
    shift-right: [w122] -> _
    shift-left: w1 -> [w129]
    shift-right: [w85] -> _
    shift-left: "Filename (variable part)" -> [w112]
    shift-right: [w78] -> _
    shift-left: "Probe 4" -> [w250]
    shift-right: [w81] -> _
    shift-left: w1 -> [w107]
    shift-right: [w82] -> _
    shift-left: w1 -> [w106]
    shift-right: [w83] -> _
    shift-left: w1 -> [w105]
    shift-right: [w84] -> _
    shift-left: w1 -> [w104]
    shift-right: [w72] -> _
    shift-left: w1 -> [w75]
    shift-right: [w73] -> _
    shift-left: w1 -> [w74]
    shift-right: [w68] -> _
    shift-left: w1 -> [w69]
    shift-right: [w67] -> _
    shift-left: w1 -> [w70]
    i -> [w210]
    stop <- "Interrupt program" stop-if-true
    w71 = FALSE
    # "Vdg for bias stress plots"
    # "Idg for bias stress plots"
    # "Vp2 for FPP bias stress plots"
    # "Vp1 for FPP bias stress plots"
    # "Ig for bias stress plots"
    # "Id for bias stress plots"
    # "Is for bias stress plots"
    # "Time axis for bias stress plots"
    # "Save bias stress curves in file."
    # "Filename prefix"
    # "Is off"
    # "Is on"
    # "Ig off"
    # "Ig on"
    # "Is min"
    # "Is max"
    # "Ig min"
    # "Ig max"
    # "Id min"
    # "Id max"
    # "Id off"
    # "Id on"
    # "Pump status"
    # "Filepath and name"
    # "Pump status"
    # "Limit of command arguments (array columns). Raise if needed."
    # "Serial port data (string)"
    # "Serial port data (table)"
    # "Time array for valve position"
    # "Time array for absolute plunger position"
    # "Valve position"
    # "Absolute plunger position"
    # "Serial port data"
    # "For loop counter"
    # "<-----Equivalent to the 4155C \"Write\" subvi.----->"
    # "Headers"
    # "Save transfer curves in file."
    # "Filepath and name"
    # "Save time-dependent data."
    # "Use the time offset if your measurements do not start at t=0."
    # "Time for Imax, Imin, Ion, Ioff"
    # "Rest of elements of command"
    # "First element of command\n(case select)"
    n21 = Add(x=w210, y=1) -> (x+y=→"Line running":i32)
    n22 = Add(x=w215, y=1) -> (x+y=→"Total lines":i32)
    n23 = Index Array(array=w243, index=0 ("line index")) -> (element=w238:string)
    "Command running:" <- w238
    n24 = control-ref of="Interrupt scan"() -> (w262:refnum<vi>)
    n25 = Spreadsheet String To Array(delimiter (Tab)=" ", format string="%s", spreadsheet string=w238, array type (2D Dbl)=string[] []) -> (array=w236:string[])
    n26 = Delete From Array(array=w236, index=0) -> (deleted portion=w149:string, array with subset deleted=w235:string[])  [unwired: 1 in]
    n27 = call "Elapsed Time"("Reset"="Reset", "Auto Reset"="Auto Reset") -> ("Elapsed Time (s)"=w245:dbl)  [unwired: 10 in, 7 out]
    n28 = case shown="1" "Time Units" {
      tunnel: ["-sec" "-min" "-h"] -> w246
      tunnel: [w275 w279 w282] -> w216
      tunnel: w245 -> [w275 w278 w283]
      frame 0, Default {
      }
      frame 1 {
        n29 = Divide(x=w278, y=60.0) -> (x/y=w279:dbl)
      }
      frame 2 {
        n30 = Divide(x=w283, y=3600.0) -> (x/y=w282:dbl)
      }
    }
    n31 = Add(x=w216, y="Time Offset") -> (x+y=w108:dbl)
    n32 = To Long Integer(number=w108) -> (32bit integer=w109:i32)
    "Elapsed Time" <- w109
    n33 = case shown="\"transfer\"" w149 {
      tunnel: w235 -> [w329 w376 w422 w434 w583 w705 w869 w1000 w1181 w1216 w1305 w1360 w1413 w1462 w1504 _ _ w1727 w1883 _ w2016 w2090 w2161 w2288 w2446 w2538 w2615 w2672]
      tunnel: w271 -> [w324 w372 w420 w456 w590 w769 w876 w1007 w1188 w1239 w1294 w1352 w1406 w1456 w1497 w1544 w1614 w1654 w1867 w1933 w2003 w2077 w2149 w2282 w2442 w2540 w2617 w2674]
      tunnel: w270 -> [w323 w371 w411 w454 w561 w754 w846 w978 w1157 w1240 w1295 w1353 w1407 w1457 w1498 w1549 w1616 w1732 w1889 w1937 w2022 w2096 w2167 w2294 w2406 w2544 w2621 w2676]
      tunnel: w269 -> [w322 w370 w410 w453 w560 w753 w845 w977 w1154 w1241 w1296 w1354 w1408 w1458 w1499 w1548 w1587 w1731 w1888 w1936 w2021 w2095 w2166 w2293 w2405 w2543 w2620 w2677]
      tunnel: w268 -> [w321 w369 w419 w451 w586 w730 w872 w1003 w1184 w1249 w1304 w1351 w1405 w1455 w1496 w1547 w1611 w1702 w1859 w1942 w1996 w2070 w2142 w2281 w2441 w2545 w2622 w2679]
      tunnel: w267 -> [w320 w368 w418 w450 w588 w767 w874 w1005 w1186 w1248 w1303 w1359 w1412 w1461 w1503 w1546 w1596 w1730 w1887 w1945 w2020 w2094 w2165 w2292 w2450 w2546 w2623 w2680]
      tunnel: w266 -> [w319 w367 w417 w448 w587 w766 w873 w1004 w1185 w1247 w1302 w1358 w1411 w1460 w1502 w1545 w1597 w1710 w1868 w1944 w2004 w2078 w2150 w2283 w2443 w2548 w2624 w2682]
      tunnel: [w323 w371 w409 w454 w585 w764 w871 w1002 w1183 w1240 w1295 w1353 w1407 w1457 w1498 w1549 w1616 w1703 w1841 w1935 w1997 w2071 w2143 w2241 w2408 w2544 w2621 w2676] -> w265
      tunnel: [w322 w370 w408 w453 w584 w763 w870 w1001 w1182 w1241 w1296 w1354 w1408 w1458 w1499 w1548 w1586 w1711 w1842 w1934 w2005 w2079 w2151 w2240 w2407 w2542 w2619 w2677] -> w182
      tunnel: [w321 w369 w419 w451 w586 w726 w872 w1003 w1184 w1242 w1297 w1351 w1405 w1455 w1496 w1547 w1611 w1702 w1859 w1942 w1996 w2070 w2142 w2281 w2441 w2545 w2622 w2679] -> w77
      tunnel: [w320 w368 w418 w450 w588 w767 w874 w1005 w1186 w1248 w1303 w1359 w1412 w1461 w1503 w1546 w1596 w1730 w1887 w1945 w2020 w2094 w2165 w2292 w2450 w2546 w2623 w2680] -> w264
      tunnel: [w319 w367 w417 w448 w587 w766 w873 w1004 w1185 w1247 w1302 w1358 w1411 w1460 w1502 w1545 w1597 w1710 w1868 w1944 w2004 w2078 w2150 w2283 w2443 w2548 w2624 w2682] -> w263
      tunnel: [w324 w372 w420 w456 w590 w769 w876 w1007 w1188 w1239 w1294 w1352 w1406 w1456 w1497 w1544 w1614 w1654 w1867 w1933 w2003 w2077 w2149 w2282 w2442 w2540 w2617 w2674] -> w86
      tunnel: w262 -> [_ _ _ _ w592 w773 w880 w1009 w1192 _ _ _ _ _ _ _ _ w1707 w1864 _ w2002 w2076 w2148 w2260 w2424 _ _ _]
      tunnel: "Gate" -> [_ _ _ _ w570 w757 w856 w987 w1168 _ _ _ _ _ _ _ _ _ _ _ _ _ _ _ _ _ _ _]
      tunnel: "Drain 2" -> [_ _ _ _ w569 w756 w855 w986 w1167 _ _ _ _ _ _ _ _ _ _ _ _ _ _ _ _ _ _ _]
      tunnel: "Panel Controls" -> [_ _ _ _ _ _ w854 w907 w1166 _ _ _ _ _ _ _ _ _ _ _ _ _ _ _ _ _ _ _]
      tunnel: w258 -> [w318 w366 w416 w447 w554 w747 w839 w971 w1152 w1246 w1301 _ w1404 w1454 w1495 w1543 w1598 w1698 w1855 w1938 w1992 w2066 w2138 w2277 w2437 w2549 w2625 w2683]
      tunnel: w257 -> [w317 w365 w415 w446 w553 w746 w838 w970 w1151 w1245 w1300 w1357 _ w1445 w1501 w1542 w1599 w1699 w1856 w1939 w1993 w2067 w2139 w2278 w2438 w2550 w2626 w2684]
      tunnel: w256 -> [w316 w364 w414 w445 w552 w745 w837 w969 w1150 w1244 w1299 w1356 w1410 w1459 _ w1541 w1600 w1700 w1857 w1940 w1994 w2068 w2140 w2279 w2439 w2551 w2627 w2685]
      tunnel: w255 -> [w315 w363 w413 w444 w551 w744 w836 w968 w1153 w1243 w1298 w1355 w1409 _ w1500 w1540 w1601 w1701 w1858 w1941 w1995 w2069 w2141 w2280 w2440 w2552 w2628 w2686]
      tunnel: [w318 w366 w416 w447 w554 w747 w839 w971 w1152 w1246 w1301 w1350 w1404 w1454 w1495 w1543 w1598 w1698 w1855 w1938 w1992 w2066 w2138 w2277 w2437 w2549 w2625 w2683] -> w254
      tunnel: [w317 w365 w415 w446 w553 w746 w838 w970 w1151 w1245 w1300 w1357 w1396 w1445 w1501 w1542 w1599 w1699 w1856 w1939 w1993 w2067 w2139 w2278 w2438 w2550 w2626 w2684] -> w253
      tunnel: [w316 w364 w414 w445 w552 w745 w837 w969 w1150 w1244 w1299 w1356 w1410 w1459 w1494 w1541 w1600 w1700 w1857 w1940 w1994 w2068 w2140 w2279 w2439 w2551 w2627 w2685] -> w252
      tunnel: [w315 w363 w413 w444 w551 w744 w836 w968 w1153 w1243 w1298 w1355 w1409 w1446 w1500 w1540 w1601 w1701 w1858 w1941 w1995 w2069 w2141 w2280 w2440 w2552 w2628 w2686] -> w251
      tunnel: w250 -> [w293 w338 w385 _ w487 w693 w805 w904 w1121 w1213 w1271 w1328 w1374 w1423 w1472 w1518 w1558 w1675 w1816 w1911 w1957 w2035 w2108 w2221 w2384 w2503 w2564 w2670]
      tunnel: w249 -> [_ _ _ _ w545 w741 _ _ _ _ _ _ _ _ _ _ _ _ _ _ _ _ _ _ _ _ _ _]
      tunnel: [w314 w359 w406 w461 w502 w718 w829 w920 w1145 w1238 w1292 w1349 w1395 w1444 w1493 w1539 w1582 w1664 w1821 w1932 w1981 w2059 w2132 w2196 w2365 w2541 w2618 w2691] -> w127
      tunnel: w248 -> [w314 w359 w406 w461 w542 w718 w829 w960 w1145 w1238 w1292 w1349 w1395 w1444 w1493 w1539 w1582 w1671 w1821 w1932 w1981 w2059 w2132 w2202 w2369 w2541 w2618 w2691]
      tunnel: w108 -> [_ _ _ _ w541 w715 w827 w959 w1142 _ _ _ _ _ _ _ w1580 w1691 w1838 _ w1978 w2056 w2129 w2237 w2399 _ _ _]
      tunnel: w246 -> [_ _ _ _ w538 w714 w825 w956 w1141 _ _ _ _ _ _ _ w1578 w1689 w1837 _ w1977 w2055 w2128 w2236 w2400 _ w2591 _]
      tunnel: w109 -> [_ _ _ _ w534 _ _ w952 _ _ _ _ _ _ _ _ _ _ _ _ _ _ _ _ _ _ w2594 _]
      tunnel: [w313 w358 w405 w449 w506 w717 w828 w924 w1144 w1237 w1291 w1348 w1394 w1443 w1492 w1538 w1581 w1656 w1804 w1931 w1980 w2058 w2131 w2190 w2359 w2547 w2598 w2681] -> w185
      tunnel: w244 -> [w313 w358 w405 w449 w537 w717 w828 w955 w1144 w1237 w1291 w1348 w1394 w1443 w1492 w1538 w1581 w1660 w1805 w1931 w1980 w2058 w2131 w2191 w2360 w2547 w2598 w2681]
      tunnel: [w312 w357 w404 w460 w501 w713 w824 w919 w1140 w1236 w1290 w1347 w1393 w1442 w1491 w1537 w1577 w1663 w1820 w1930 w1976 w2054 w2127 w2195 w2364 w2536 w2614 w2690] -> w126
      tunnel: w220 -> [w312 w357 w404 w460 w533 w713 w824 w951 w1140 w1236 w1290 w1347 w1393 w1442 w1491 w1537 w1577 w1670 w1820 w1930 w1976 w2054 w2127 w2201 w2368 w2536 w2614 w2690]
      tunnel: [w311 w356 w403 w443 w526 w712 w823 w944 w1139 w1235 w1289 w1346 w1392 w1441 w1490 w1536 w1576 w1688 w1836 w1929 w1975 w2053 w2126 w2235 w2398 w2535 w2613 w2687] -> w158
      tunnel: w207 -> [w311 w356 w403 w443 w526 w712 w823 w944 w1139 w1235 w1289 w1346 w1392 w1441 w1490 w1536 w1576 w1688 w1836 w1929 w1975 w2053 w2126 w2235 w2398 w2534 w2592 w2687]
      tunnel: [w310 w355 w402 w471 w525 w711 w822 w943 w1138 w1234 w1288 w1345 w1391 w1440 w1489 w1535 w1575 w1687 w1835 w1928 w1974 w2052 w2125 w2234 w2397 w2520 w2600 w2701] -> w186
      tunnel: w202 -> [w310 w355 w402 w471 w525 w711 w822 w943 w1138 w1234 w1288 w1345 w1391 w1440 w1489 w1535 w1575 w1687 w1835 w1928 w1974 w2052 w2125 w2234 w2397 w2520 w2599 w2701]
      tunnel: [w309 w354 w401 w473 w524 w710 w821 w942 w1137 w1233 w1287 w1344 w1390 w1439 w1488 w1534 w1574 w1686 w1834 w1927 w1973 w2051 w2124 w2233 w2396 w2519 w2587 w2703] -> w168
      tunnel: w201 -> [w309 w354 w401 w473 w524 w710 w821 w942 w1137 w1233 w1287 w1344 w1390 w1439 w1488 w1534 w1574 w1686 w1834 w1927 w1973 w2051 w2124 w2233 w2396 w2519 w2585 w2703]
      tunnel: [w308 w353 w400 w457 w523 w709 w820 w941 w1136 w1232 w1286 w1343 w1389 w1438 w1487 w1533 w1573 w1685 w1833 w1926 w1972 w2050 w2123 w2232 w2395 w2518 w2584 w2675] -> w200
      tunnel: w199 -> [w308 w353 w400 w457 w523 w709 w820 w941 w1136 w1232 w1286 w1343 w1389 w1438 w1487 w1533 w1573 w1685 w1833 w1926 w1972 w2050 w2123 w2232 w2395 w2518 w2595 w2675]
      tunnel: w109 -> [_ _ _ _ _ _ _ _ _ _ _ _ _ _ _ _ _ _ _ _ _ _ _ _ _ _ w2583 _]
      tunnel: w183 -> [w307 w352 w399 w472 w522 w708 w819 w940 w1135 w1231 w1285 w1342 w1388 w1437 w1486 w1532 w1572 w1684 w1832 w1925 w1971 w2049 w2122 w2231 w2394 w2517 w2582 w2702]
      tunnel: [w307 w352 w399 w472 w522 w708 w819 w940 w1135 w1231 w1285 w1342 w1388 w1437 w1486 w1532 w1572 w1684 w1832 w1925 w1971 w2049 w2122 w2231 w2394 w2517 w2581 w2702] -> w163
      tunnel: [w306 w351 w398 w470 w521 w707 w818 w939 w1134 w1230 w1284 w1341 w1387 w1436 w1485 w1531 w1571 w1683 w1831 w1924 w1970 w2048 w2121 w2230 w2393 w2516 w2580 w2700] -> w162
      tunnel: w167 -> [w306 w351 w398 w470 w521 w707 w818 w939 w1134 w1230 w1284 w1341 w1387 w1436 w1485 w1531 w1571 w1683 w1831 w1924 w1970 w2048 w2121 w2230 w2393 w2516 w2579 w2700]
      tunnel: [w305 w350 w397 w452 w520 w706 w817 w938 w1133 w1229 w1283 w1340 w1386 w1435 w1484 w1530 w1570 w1682 w1830 w1923 w1969 w2047 w2120 w2229 w2392 w2515 w2577 w2678] -> w159
      tunnel: w161 -> [w305 w350 w397 w452 w520 w706 w817 w938 w1133 w1229 w1283 w1340 w1386 w1435 w1484 w1530 w1570 w1682 w1830 w1923 w1969 w2047 w2120 w2229 w2392 w2515 w2576 w2678]
      tunnel: [w303 w348 w395 w466 w495 w703 w815 w913 w1131 w1227 w1282 w1339 w1384 w1433 w1482 w1528 w1568 w1681 w1829 w1922 w1968 w2046 w2118 w2228 w2391 w2514 w2575 w2696] -> w120
      tunnel: w148 -> [w303 w348 w395 w466 w519 w703 w815 w937 w1131 w1227 w1282 w1339 w1384 w1433 w1482 w1528 w1568 w1681 w1829 w1922 w1968 w2046 w2118 w2228 w2391 w2514 w2575 w2696]
      tunnel: [w304 w349 w396 w467 w496 w704 w816 w914 w1132 w1228 w1281 w1338 w1385 w1434 w1483 w1529 w1569 w1680 w1828 w1921 w1967 w2045 w2119 w2227 w2390 w2513 w2574 w2697] -> w121
      tunnel: w147 -> [w304 w349 w396 w467 w518 w704 w816 w936 w1132 w1228 w1281 w1338 w1385 w1434 w1483 w1529 w1569 w1680 w1828 w1921 w1967 w2045 w2119 w2227 w2390 w2513 w2574 w2697]
      tunnel: [w296 w341 w388 w459 w500 w700 w813 w918 w1129 w1220 w1279 w1336 w1382 w1431 w1480 w1526 w1561 w1662 w1819 w1920 w1960 w2038 w2111 w2194 w2363 w2506 w2573 w2689] -> w125
      tunnel: w136 -> [w296 w341 w388 w459 w514 w700 w813 w932 w1129 w1220 w1279 w1336 w1382 w1431 w1480 w1526 w1561 w1669 w1819 w1920 w1960 w2038 w2111 w2200 w2367 w2506 w2573 w2689]
      tunnel: [w295 w340 w387 w458 w499 w701 w814 w917 w1130 w1219 w1280 w1337 w1383 w1432 w1481 w1527 w1560 w1661 w1818 w1919 w1959 w2037 w2110 w2193 w2362 w2505 w2572 w2688] -> w124
      tunnel: w135 -> [w295 w340 w387 w458 w513 w701 w814 w931 w1130 w1219 w1280 w1337 w1383 w1432 w1481 w1527 w1560 w1668 w1818 w1919 w1959 w2037 w2110 w2199 w2366 w2505 w2572 w2688]
      tunnel: [w298 w343 w390 w463 w505 w699 w811 w923 w1127 w1225 w1277 w1334 w1380 w1429 w1478 w1524 w1563 w1666 w1823 w1914 w1962 w2040 w2113 w2198 w2372 w2510 w2570 w2693] -> w118
      tunnel: w134 -> [w298 w343 w390 w463 w512 w699 w811 w930 w1127 w1225 w1277 w1334 w1380 w1429 w1478 w1524 w1563 w1673 w1823 w1914 w1962 w2040 w2113 w2204 w2373 w2510 w2570 w2693]
      tunnel: [w297 w342 w389 w462 w503 w702 w812 w921 w1128 w1226 w1278 w1335 w1381 w1430 w1479 w1525 w1562 w1665 w1822 w1913 w1961 w2039 w2112 w2197 w2370 w2509 w2571 w2692] -> w128
      tunnel: w133 -> [w297 w342 w389 w462 w511 w702 w812 w929 w1128 w1226 w1278 w1335 w1381 w1430 w1479 w1525 w1562 w1672 w1822 w1913 w1961 w2039 w2112 w2203 w2371 w2509 w2571 w2692]
      tunnel: [w300 w345 w392 w465 w494 w698 w809 w912 w1125 w1223 w1275 w1332 w1378 w1427 w1476 w1522 w1565 w1677 w1825 w1916 w1964 w2042 w2115 w2224 w2387 w2512 w2568 w2695] -> w119
      tunnel: w132 -> [w300 w345 w392 w465 w510 w698 w809 w928 w1125 w1223 w1275 w1332 w1378 w1427 w1476 w1522 w1565 w1677 w1825 w1916 w1964 w2042 w2115 w2224 w2387 w2512 w2568 w2695]
      tunnel: [w299 w344 w391 w464 w493 w697 w810 w911 w1126 w1224 w1276 w1333 w1379 w1428 w1477 w1523 w1564 w1676 w1824 w1915 w1963 w2041 w2114 w2223 w2386 w2511 w2569 w2694] -> w117
      tunnel: w131 -> [w299 w344 w391 w464 w509 w697 w810 w927 w1126 w1224 w1276 w1333 w1379 w1428 w1477 w1523 w1564 w1676 w1824 w1915 w1963 w2041 w2114 w2223 w2386 w2511 w2569 w2694]
      tunnel: [w302 w347 w394 w469 w498 w696 w807 w916 w1123 w1221 w1273 w1330 w1376 w1425 w1474 w1520 w1567 w1679 w1827 w1918 w1966 w2044 w2117 w2226 w2389 w2508 w2566 w2699] -> w123
      tunnel: w130 -> [w302 w347 w394 w469 w508 w696 w807 w926 w1123 w1221 w1273 w1330 w1376 w1425 w1474 w1520 w1567 w1679 w1827 w1918 w1966 w2044 w2117 w2226 w2389 w2508 w2566 w2699]
      tunnel: [w301 w346 w393 w468 w497 w695 w808 w915 w1124 w1222 w1274 w1331 w1377 w1426 w1475 w1521 w1566 w1678 w1826 w1917 w1965 w2043 w2116 w2225 w2388 w2507 w2567 w2698] -> w122
      tunnel: w129 -> [w301 w346 w393 w468 w507 w695 w808 w925 w1124 w1222 w1274 w1331 w1377 w1426 w1475 w1521 w1566 w1678 w1826 w1917 w1965 w2043 w2116 w2225 w2388 w2507 w2567 w2698]
      tunnel: w112 -> [w294 w339 w386 w455 w490 w694 w806 w908 w1122 w1218 w1272 w1329 w1375 w1424 w1473 w1519 w1559 w1653 w1817 w1912 w1958 w2036 w2109 w2222 w2385 w2504 w2565 _]
      tunnel: [w294 w339 w386 w455 w490 w694 w806 w908 w1122 w1218 w1272 w1329 w1375 w1424 w1473 w1519 w1559 w1653 w1817 w1912 w1958 w2036 w2109 w2222 w2385 w2504 w2565 w2671] -> w85
      tunnel: [w293 w338 w385 w433 w487 w693 w805 w904 w1121 w1213 w1271 w1328 w1374 w1423 w1472 w1518 w1558 w1675 w1816 w1911 w1957 w2035 w2108 w2221 w2384 w2503 w2564 w2670] -> w78
      tunnel: w108 -> [_ _ _ _ _ _ _ _ _ _ _ _ _ _ _ _ _ w1623 w1800 _ _ _ _ w2206 w2376 _ _ _]
      tunnel: [w292 w337 w384 w432 w486 w692 w804 w903 w1120 w1212 w1270 w1327 w1373 w1422 w1471 w1517 w1557 w1637 w1815 w1910 w1956 w2034 w2107 w2211 w2380 w2502 w2563 w2669] -> w81
      tunnel: [w291 w336 w383 w431 w485 w691 w803 w902 w1119 w1211 w1269 w1326 w1372 w1421 w1470 w1516 w1556 w1636 w1814 w1909 w1955 w2033 w2106 w2172 w2341 w2501 w2562 w2668] -> w82
      tunnel: [w290 w335 w382 w430 w484 w690 w802 w901 w1118 w1210 w1268 w1325 w1371 w1420 w1469 w1515 w1555 w1638 w1787 w1908 w1954 w2032 w2105 w2184 w2353 w2500 w2561 w2667] -> w83
      tunnel: [w289 w334 w381 w429 w483 w689 w801 w900 w1117 w1209 w1267 w1324 w1370 w1419 w1468 w1514 w1554 w1635 w1794 w1907 w1953 w2031 w2104 w2181 w2350 w2499 w2560 w2666] -> w84
      tunnel: w107 -> [w292 w337 w384 w432 w486 w692 w804 w903 w1120 w1212 w1270 w1327 w1373 w1422 w1471 w1517 w1557 w1634 w1815 w1910 w1956 w2034 w2107 w2214 w2383 w2502 w2563 w2669]
      tunnel: w106 -> [w291 w336 w383 w431 w485 w691 w803 w902 w1119 w1211 w1269 w1326 w1372 w1421 w1470 w1516 w1556 w1633 w1814 w1909 w1955 w2033 w2106 w2213 w2382 w2501 w2562 w2668]
      tunnel: w105 -> [w290 w335 w382 w430 w484 w690 w802 w901 w1118 w1210 w1268 w1325 w1371 w1420 w1469 w1515 w1555 w1632 w1788 w1908 w1954 w2032 w2105 w2184 w2353 w2500 w2561 w2667]
      tunnel: w104 -> [w289 w334 w381 w429 w483 w689 w801 w900 w1117 w1209 w1267 w1324 w1370 w1419 w1468 w1514 w1554 w1631 w1796 w1907 w1953 w2031 w2104 w2212 w2381 w2499 w2560 w2666]
      tunnel: "Standby" -> [_ _ _ _ w482 w688 _ w899 _ _ _ _ _ _ _ _ _ w1629 w1813 _ _ _ _ w2220 _ _ _ _]
      tunnel: w75 -> [w288 w333 w380 w428 w476 w682 w795 w893 w1110 w1208 w1266 w1323 w1369 w1418 w1467 w1513 w1553 w1620 w1808 w1906 w1949 w2028 w2102 w2178 w2347 w2498 w2559 w2665]
      tunnel: [w288 w333 w380 w428 w476 w682 w795 w893 w1110 w1208 w1266 w1323 w1369 w1418 w1467 w1513 w1553 w1620 w1808 w1906 w1949 w2028 w2102 w2173 w2342 w2498 w2559 w2665] -> w72
      tunnel: w74 -> [w287 w332 w379 w427 w477 w681 w794 w894 w1111 w1207 w1265 w1322 w1368 w1417 w1466 w1512 w1552 w1619 w1807 w1905 w1948 w2027 w2101 w2177 w2346 w2497 w2558 w2664]
      tunnel: [w287 w332 w379 w427 w477 w681 w794 w894 w1111 w1207 w1265 w1322 w1368 w1417 w1466 w1512 w1552 w1619 w1807 w1905 w1948 w2027 w2101 w2176 w2345 w2497 w2558 w2664] -> w73
      tunnel: w70 -> [w285 w330 w377 w425 w475 w680 w785 w892 w1097 w1206 w1264 w1321 w1367 w1415 w1464 w1510 w1550 w1617 w1793 w1903 w1946 w2025 w2099 w2170 w2339 w2495 w2553 w2662]
      tunnel: w69 -> [w286 w331 w378 w426 w474 w679 w784 w891 w1096 w1205 w1263 w1320 w1366 w1416 w1465 w1511 w1551 w1618 w1791 w1904 w1947 w2026 w2100 w2171 w2340 w2496 w2554 w2663]
      tunnel: [w286 w331 w378 w426 w474 w679 w784 w891 w1096 w1205 w1263 w1320 w1366 w1416 w1465 w1511 w1551 w1618 w1785 w1904 w1947 w2026 w2100 w2171 w2340 w2496 w2554 w2663] -> w68
      tunnel: [w285 w330 w377 w425 w475 w680 w785 w892 w1097 w1206 w1264 w1321 w1367 w1415 w1464 w1510 w1550 w1617 w1792 w1903 w1946 w2025 w2099 w2170 w2339 w2495 w2553 w2662] -> w67
      frame "wait" {
        n34 = Index Array(array=w329, index=0 ("Index")) -> (element=w327:string)
        n35 = Decimal String To Number(string=w327, default (0L)=u32 0) -> (number=w326:u32)  [unwired: 1 in, 1 out]
        n36 = Wait (ms)(milliseconds to wait=w326) -> ()  [unwired: 1 out]
      }
      frame "wait-min" {
        n37 = Index Array(array=w376, index=0 ("Index")) -> (element=w374:string)
        n38 = Decimal String To Number(string=w374, default (0L)=u32 0) -> (number=w362:u32)  [unwired: 1 in, 1 out]
        n39 = Multiply(x=w362, y=u32 60000) -> (x*y=w361:u32)
        n40 = Wait (ms)(milliseconds to wait=w361) -> ()  [unwired: 1 out]
      }
      frame "standby" {
        n41 = Index Array(array=w422, index=0 ("Index")) -> (element=w412:string)
        n42 = case shown="\"off\", Default" w412 {
          tunnel: [":PAGE:SCON:STAN 0" ":PAGE:SCON:STAN 1"] -> w407
          frame "off", Default {
          }
          frame "on" {
          }
        }
        n43 = VISA Write(VISA resource name=w411, write buffer=w407, error in (no error)=w410) -> (VISA resource name out=w409:refnum<visa-resource-name>, error out=w408:errorcluster)  [unwired: 1 out]
      }
      frame "Probe4" {
        n44 = Delete From Array(array=w434, index=0) -> (deleted portion=w437:string, array with subset deleted=w440:string[])  [unwired: 1 in]
        n45 = Equal?(x=w437, y="ON") -> (x = y?=w435:bool)
        n46 = Delete From Array(array=w440, index=0) -> (deleted portion=w439:string)  [unwired: 1 in, 1 out]
        n47 = Fract/Exp String To Number(string=w439) -> (number=w436:dbl)  [unwired: 3 in, 1 out]
        n48 = Bundle(w435, w436) -> (w433:cluster{bool, dbl})  [unwired: 1 in]
      }
      frame "transfer" {
        # "Is off"
        # "Is on"
        # "Ig off"
        # "Ig on"
        # "Is min"
        # "Is max"
        # "Ig min"
        # "Ig max"
        # "Id min"
        # "Id max"
        # "Id off"
        # "Id on"
        n49 = Delete From Array(array=w583, index=0 ("Index")) -> (deleted portion=w581:string, array with subset deleted=w580:string[])  [unwired: 1 in]
        n50 = Bundle By Name(cluster=w545, "Emergency Stop"=w592) -> (w546:T2)
        n51 = local read "Transfer/Output - Source/Common"() -> (w481:u32)
        n52 = Number To Decimal String(number=w541) -> (decimal integer string=w540:string)  [unwired: 1 in]
        n53 = case shown="\"d\", Default" w581 {
          tunnel: [w677 w678] -> w579
          frame "s" {
            w677 = u16 0 items=["Single", "Double"] ("sweep mode")
          }
          frame "d", Default {
            w678 = u16 1 items=["Single", "Double"] ("sweep mode")
          }
        }
        n54 = Fract/Exp String To Number(string=w580) -> (number=w565:dbl[])  [unwired: 3 in, 1 out]
        n55 = Concatenate Strings(w590, w490, w540, w538, "_T_1_C_L.txt" ("Suffix (transfer)")) -> (w591:string)
        n56 = VISA Write(VISA resource name=w561, write buffer=":PAGE:CHAN:MODE SWE;" ("write buffer (\"\")"), error in (no error)=w560) -> (VISA resource name out=w558:refnum<visa-resource-name>, error out=w559:errorcluster)  [unwired: 1 out]
        n57 = local read "Plot transfer curve extrema vs time"() -> (w488:bool)
        n58 = local read "Transfer/Output - Gate"() -> (w479:u32)
        n59 = local read "Transfer/Output - Drain"() -> (w480:u32)
        n60 = String To Path(string=w591) -> (path=w589:path)
        n61 = local read "Transfer/Output - Probe 4"() -> (w478:u32)
        n62 = Index Array(array=w565, index #1=0 ("Index")) -> (element #1=w578:dbl, element #2=w577:dbl, element #3=w576:dbl)  [unwired: 2 in]
        n63 = Delete From Array(array=w565, length=3 ("Length"), index=0 ("Index")) -> (array with subset deleted=w563:dbl[])  [unwired: 1 out]
        n64 = case shown="True" w488 {
          tunnel: w537 -> [w594 w597]
          tunnel: w534 -> [_ w596]
          tunnel: [w594 w595] -> w506
          frame False {
          }
          frame True {
            n65 = Build Array (concatenate)(w597, w596) -> (w595:i32[])
          }
        }
        n66 = Bundle By Name(cluster=w570, "Gate Start"=w578, "Gate Stop"=w577, "Gate Step (linear only)"=w576, "Gate Compliance"=w587, "Range mode"=w554, "Range"=w553) -> (w555:T6)
        n67 = Index Array(array=w563, index #1=0 ("Index")) -> (element #1=w573:dbl, element #2=w572:dbl, element #3=w571:dbl)  [unwired: 2 in]
        n68 = call <vilib>:"compatOverwrite.vi"("overwrite (F)"=TRUE) -> ("overwrite?"=w544:T8)
        n69 = Bundle By Name(cluster=w569, "Drain Start"=w573, "Drain Stop"=w572, "Drain Step"=w571, "Drain Compliance"=w588, "Range mode"=w552, "Range"=w551) -> (w556:T7)
        n70 = call "4155C Transfer v3.0.vi"("VISA resource name in"=w558, "Source/Common"=w481, 2:"Gate"=w555, 3:"Drain"=w556, 4:"Drain"=w480, "Timings"=w586, "error in (no error)"=w559, 7:"Probe 4"=w487, 8:"Gate"=w479, 9:"Probe 4"=w478, "sweep mode"=w579, "Panel Controls"=w546, "Standby"=w482) -> ("VG"=w543:dbl[], "Outparams"=w550:T9, "VISA Resource Name out"=w585:refnum<visa-resource-name>, "IS"=w516:dbl[], "ID"=w517:dbl[], "IG"=w515:dbl[], "error out"=w535:errorcluster, "Probe 4"=w547:dbl[])  [unwired: 7 in]
        n71 = Unbundle By Name(w550) -> ("V2 Step"=w549:dbl, "V2 Start"=w548:dbl, "Number of points"=w504:i32)
        n72 = call "4155C Split array.vi"("Number of VAR2 steps"=w504, "Y2 data in"=w517, "X data in"=w543, "Y1 data in"=w516, "Y3 data in"=w515, "error in (no error)"=w535) -> ("Array of clusters"=w536:cluster{"Y data in":dbl[], "X data in":dbl[]}[], "error out"=w492:errorcluster)  [unwired: 1 in]
        n73 = case shown="True" "Plot transfer curve extrema vs time" {
          tunnel: w542 -> [w606 w676]
          tunnel: w533 -> [w607 w671]
          tunnel: w519 -> [w600 w667]
          tunnel: w518 -> [w601 w666]
          tunnel: w517 -> [_ w663]
          tunnel: w516 -> [_ w661]
          tunnel: w515 -> [_ w660]
          tunnel: w514 -> [w608 w656]
          tunnel: w513 -> [w609 w655]
          tunnel: w512 -> [w604 w652]
          tunnel: w511 -> [w605 w651]
          tunnel: w510 -> [w599 w648]
          tunnel: w509 -> [w598 w647]
          tunnel: w508 -> [w603 w644]
          tunnel: w507 -> [w602 w643]
          tunnel: w506 -> [_ w636]
          tunnel: [w604 w631] -> w505
          tunnel: w504 -> [_ w630]
          tunnel: [w605 w629] -> w503
          tunnel: [w606 w628] -> w502
          tunnel: [w607 w627] -> w501
          tunnel: [w608 w626] -> w500
          tunnel: [w609 w625] -> w499
          tunnel: [w603 w624] -> w498
          tunnel: [w602 w623] -> w497
          tunnel: [w601 w622] -> w496
          tunnel: [w600 w621] -> w495
          tunnel: [w599 w620] -> w494
          tunnel: [w598 w619] -> w493
          tunnel: w492 -> [w610 w618]
          tunnel: [w610 w614] -> w491
          frame False {
          }
          frame True {
            # "Adjusts graph colors."
            # "Adjusts graph colors."
            # "Ion will be the middle element of the array. The calculation of the index is done only once, since Is, Id, and Ig have the same dimensions."
            # "abs(Ig)"
            # "abs(Is)"
            # "Y1: Is\nY2: Id\nY3: Ig"
            # "abs(Id)"
            # "Adjusts graph colors."
            # "Adjusts graph colors."
            # "Adjusts graph colors."
            n74 = Absolute Value(x=w661) -> (abs(x)=w646:dbl[])
            n75 = Absolute Value(x=w663) -> (abs(x)=w662:dbl[])
            n76 = Absolute Value(x=w660) -> (abs(x)=w649:dbl[])
            n77 = Array Size(array=w662) -> (size(s)=w670:i32)
            n78 = Divide(x=w670, y=2) -> (x/y=w613:dbl)
            n79 = Subtract(x=w613, y=1) -> (x-y=w612:dbl)
            n80 = Array Max & Min(array=w646) -> (max value=w653:dbl, min value=w654:dbl)  [unwired: 2 out]
            n81 = Array Max & Min(array=w662) -> (max value=w675:dbl, min value=w659:dbl)  [unwired: 2 out]
            n82 = Array Max & Min(array=w649) -> (max value=w658:dbl, min value=w657:dbl)  [unwired: 2 out]
            n83 = Index Array(array=w646, index=w612) -> (element=w637:dbl)
            n84 = Index Array(array=w646, index=0) -> (element=w638:dbl)
            n85 = Index Array(array=w662, index=w612) -> (element=w639:dbl)
            n86 = Index Array(array=w662, index=0) -> (element=w640:dbl)
            n87 = Index Array(array=w649, index=w612) -> (element=w642:dbl)
            n88 = Index Array(array=w649, index=0) -> (element=w641:dbl)
            n89 = local write "Ig max"(w658) -> ()
            n90 = local write "Ig min"(w657) -> ()
            n91 = local write "Is max"(w653) -> ()
            n92 = local write "Is min"(w654) -> ()
            n93 = local write "Id max"(w675) -> ()
            n94 = local write "Id min"(w659) -> ()
            n95 = Build Array (concatenate)(w652, w653) -> (w631:dbl[])
            n96 = Build Array (concatenate)(w651, w654) -> (w629:dbl[])
            n97 = local write "Is off"(w638) -> ()
            n98 = local write "Is on"(w637) -> ()
            n99 = Build Array (concatenate)(w676, w675) -> (w628:dbl[])
            n100 = Build Array (concatenate)(w671, w659) -> (w627:dbl[])
            n101 = Build Array (concatenate)(w656, w658) -> (w626:dbl[])
            n102 = Build Array (concatenate)(w655, w657) -> (w625:dbl[])
            n103 = Build Array (concatenate)(w644, w637) -> (w624:dbl[])
            n104 = Build Array (concatenate)(w643, w638) -> (w623:dbl[])
            n105 = Build Array (concatenate)(w666, w639) -> (w622:dbl[])
            n106 = Build Array (concatenate)(w667, w640) -> (w621:dbl[])
            n107 = Build Array (concatenate)(w648, w642) -> (w620:dbl[])
            n108 = Build Array (concatenate)(w647, w641) -> (w619:dbl[])
            n109 = local write "Ig off"(w641) -> ()
            n110 = local write "Ig on"(w642) -> ()
            n111 = local write "Id off"(w640) -> ()
            n112 = local write "Id on"(w639) -> ()
            n113 = control-ref of="Imax vs time"() -> (w665:refnum<vi>)
            n114 = control-ref of="Imin vs time"() -> (w664:refnum<vi>)
            n115 = control-ref of="Ion vs time"() -> (w633:refnum<vi>)
            n116 = control-ref of="Ioff vs time"() -> (w632:refnum<vi>)
            n117 = control-ref of="I vs Vg"() -> (w674:refnum<vi>)
            n118 = call "4155C Split array.vi"("Number of VAR2 steps"=w630, "Y2 data in"=w622, "X data in"=w636, "Y1 data in"=w624, "Y3 data in"=w620, "error in (no error)"=w618) -> ("Array of clusters"=w634:cluster{"Y data in":dbl[], "X data in":dbl[]}[], "error out"=w617:errorcluster)  [unwired: 1 in]
            n119 = call "4155C Split array.vi"("Number of VAR2 steps"=w630, "Y2 data in"=w621, "X data in"=w636, "Y1 data in"=w623, "Y3 data in"=w619, "error in (no error)"=w617) -> ("Array of clusters"=w635:cluster{"Y data in":dbl[], "X data in":dbl[]}[], "error out"=w616:errorcluster)  [unwired: 1 in]
            n120 = call "4155C Split array.vi"("Number of VAR2 steps"=w630, "Y2 data in"=w628, "X data in"=w636, "Y1 data in"=w631, "Y3 data in"=w626, "error in (no error)"=w616) -> ("Array of clusters"=w673:cluster{"Y data in":dbl[], "X data in":dbl[]}[], "error out"=w615:errorcluster)  [unwired: 1 in]
            n121 = call "4155C Split array.vi"("Number of VAR2 steps"=w630, "Y2 data in"=w627, "X data in"=w636, "Y1 data in"=w629, "Y3 data in"=w625, "error in (no error)"=w615) -> ("Array of clusters"=w672:cluster{"Y data in":dbl[], "X data in":dbl[]}[], "error out"=w614:errorcluster)  [unwired: 1 in]
            n122 = call "4155C Config Chart Colours.vi"("Numeric"=w630, "XY Graph 2"=w665) -> ()  [unwired: 6 in]
            n123 = call "4155C Config Chart Colours.vi"("Numeric"=w630, "XY Graph 2"=w664) -> ()  [unwired: 6 in]
            n124 = call "4155C Config Chart Colours.vi"("Numeric"=w630, "XY Graph 2"=w633) -> ()  [unwired: 6 in]
            n125 = call "4155C Config Chart Colours.vi"("Numeric"=w630, "XY Graph 2"=w632) -> ()  [unwired: 6 in]
            n126 = call "4155C Config Chart Colours.vi"("Numeric"=w630, "XY Graph 2"=w674) -> ()  [unwired: 6 in]
            n127 = local write "Imax vs time"(w673) -> ()
            n128 = local write "Imin vs time"(w672) -> ()
            n129 = local write "Ion vs time"(w634) -> ()
            n130 = local write "Ioff vs time"(w635) -> ()
          }
        }
        n131 = local write "I vs Vg"(w536) -> ()
        n132 = Open/Create/Replace File(file path (use dialog)=w589, error in=w491, operation (0:open)=w544) -> (refnum out=w531:refnum<file>, error out=w529:errorcluster)  [unwired: 3 in, 1 out]
        n133 = call "4155C Make Big 2d array.vi"("1D Var1"=w543, "1d IS"=w516, "1d ID"=w517, "1d IG"=w515, "1d SMU4"=w547, "SMU4"=w487, "VAR2 START"=w548, "Number of VAR2 steps"=w504, "VAR2 STEP"=w549, "VAR1 Name"="Vg", "Decimal places in header"=i8 1, "VAR2 Name"="Vd") -> ("Header array"=w532:string[], "Data array"=w530:dbl[][])  [unwired: 14 in]
        n134 = call "4155C Write array to file.vi"("Byte Stream File Refnum"=w531, "Header"=w532, "Data Array"=w530, "error in (no error)"=w529) -> ("dup refnum"=w528:refnum<file>, "error out"=w527:errorcluster)  [unwired: 1 in]
        n135 = Close File(refnum=w528, error in=w527) -> (error out=w584:errorcluster)  [unwired: 1 out]
      }
      frame "pulsedstressV" {
        w724 = 0
        n136 = local read "Pulsed Stress V - Source/Common"() -> (w687:u32)
        n137 = local read "Pulsed Stress V - Probe 4"() -> (w684:u32)
        n138 = Number To Decimal String(number=w715) -> (decimal integer string=w770:string)  [unwired: 1 in]
        n139 = local read "Pulsed Stress V - Vextra"() -> (w683:u32)
        n140 = local read "Pulsed Stress V - Drain"() -> (w686:u32)
        n141 = local read "Pulsed Stress V - Gate"() -> (w685:u32)
        n142 = Delete From Array(array=w705, index=0 ("Index")) -> (deleted portion=w761:string, array with subset deleted=w760:string[])  [unwired: 1 in]
        n143 = Bundle By Name(cluster=w741, "Emergency Stop"=w773) -> (w742:T2)
        n144 = VISA Write(VISA resource name=w754, write buffer=":PAGE:CHAN:MODE SWE;" ("write buffer (\"\")"), error in (no error)=w753) -> (VISA resource name out=w751:refnum<visa-resource-name>, error out=w752:errorcluster)  [unwired: 1 out]
        n145 = Concatenate Strings(w769, "-pulsedstressV-" ("Substring"), w770, w714, ".txt" ("Substring")) -> (w772:string)
        n146 = case shown="\"d\", Default" w761 {
          tunnel: [w782 w783] -> w759
          frame "s" {
            w782 = u16 0 items=["Single", "Double"] ("sweep mode")
          }
          frame "d", Default {
            w783 = u16 1 items=["Single", "Double"] ("sweep mode")
          }
        }
        n147 = Fract/Exp String To Number(string=w760) -> (number=w755:dbl[])  [unwired: 3 in, 1 out]
        n148 = String To Path(string=w772) -> (path=w768:path)
        n149 = Index Array(array=w755, index #1=0 ("Index")) -> (element #1=w733:dbl, element #2=w732:dbl, element #3=w729:dbl, element #4=w728:dbl, element #5=w727:dbl, element #6=w731:dbl)  [unwired: 5 in]
        n150 = Bundle By Name(cluster=w730, "Pulse period"=w728, "Base voltage"=w729, "Pulse width"=w727) -> (w726:T5)
        n151 = Unbundle By Name(w726) -> ("Pulse period"=w734:dbl)
        n152 = Bundle By Name(cluster=w757, "Gate Start"=w732, "Gate Stop"=w733, "Gate Step (linear only)"=0, "Gate Compliance"=w766, "Range mode"=w747, "Range"=w746) -> (w748:T6)
        n153 = call <vilib>:"compatOverwrite.vi"("overwrite (F)"=TRUE) -> ("overwrite?"=w719:T8)
        n154 = Bundle By Name(cluster=w756, "Drain Start"=w731, "Drain Stop"=w724, "Drain Step"=w724, "Drain Compliance"=w767, "Range mode"=w745, "Range"=w744) -> (w749:T7)
        n155 = call "4155C PulsedStressV v3.0.vi"("VISA resource name in"=w751, "Gate"=w748, "Pulsed Stress V - Source/Common"=w687, "Drain"=w749, "Timings"=w726, "error in (no error)"=w752, "sweep mode"=w759, "Probe 4"=w693, "Pulsed Stress V - Drain"=w686, "Pulsed Stress V - Gate"=w685, "Panel Controls"=w742, "Standby"=w688, "Pulsed Stress V - Probe 4"=w684, "Pulsed Stress V - Vextra"=w683) -> ("Outparams"=w743:T9, "VISA Resource Name out"=w764:refnum<visa-resource-name>, "ID"=w722:dbl[], "IG"=w720:dbl[], "error out"=w765:errorcluster)  [unwired: 1 in]
        n156 = Unbundle By Name(w743) -> ("Number of points"=w721:i32)  [unwired: 2 out]
        n157 = for {
          N: w721 -> [_]
          tunnel: [w779] -> w723 mode=indexing
          tunnel: w734 -> [w781]
          i -> [w780]
          n158 = Multiply(x=w781, y=w780) -> (x*y=w779:dbl)
        }
        n159 = Insert Into Array(array=dbl[][] [] ("Input Array"), new element=w723) -> (w735:dbl[][])  [unwired: 2 in]
        n160 = Insert Into Array(array=w735, new element=w722) -> (w740:dbl[][])  [unwired: 2 in]
        n161 = Insert Into Array(array=w740, new element=w720) -> (w739:dbl[][])  [unwired: 2 in]
        n162 = Transpose 2D Array(2D array=w739) -> (transposed array=w738:dbl[][])
        n163 = Open/Create/Replace File(file path (use dialog)=w768, error in=w765, operation (0:open)=w719) -> (refnum out=w776:refnum<file>, error out=w777:errorcluster)  [unwired: 3 in, 1 out]
        n164 = call "4155C Write array to file.vi"("Byte Stream File Refnum"=w776, "Header"=string[] ["Time /s", "Id /A", "Ig /A"], "Data Array"=w738, "error in (no error)"=w777) -> ("dup refnum"=w774:refnum<file>, "error out"=w775:errorcluster)  [unwired: 1 in]
        n165 = Close File(refnum=w774, error in=w775) -> (error out=w763:errorcluster)  [unwired: 1 out]
      }
      frame "transfer-fpp" {
        # "Adjusts graph colors."
        # "Y1 = Y2 = ID\nY3 = IG"
        n166 = local read "FPP - Source"() -> (w800:u32)
        n167 = local read "FPP - Drain"() -> (w798:u32)
        n168 = local read "FPP - Gate"() -> (w799:u32)
        n169 = local read "FPP - Probe 1"() -> (w797:u32)
        n170 = local read "FPP - Probe 2"() -> (w796:u32)
        n171 = Number To Decimal String(number=w827) -> (decimal integer string=w877:string)  [unwired: 1 in]
        n172 = Bundle By Name(cluster=w854, "Emergency Stop"=w880) -> (w888:T1)
        n173 = Delete From Array(array=w869, index=0 ("Index")) -> (deleted portion=w867:string, array with subset deleted=w866:string[])  [unwired: 1 in]
        n174 = Concatenate Strings(w876, "-transferfpp-" ("Substring"), w877, w825, ".txt" ("Substring")) -> (w879:string)
        n175 = VISA Write(VISA resource name=w846, write buffer=":PAGE:CHAN:MODE SWE;" ("write buffer (\"\")"), error in (no error)=w845) -> (VISA resource name out=w843:refnum<visa-resource-name>, error out=w844:errorcluster)  [unwired: 1 out]
        n176 = case shown="\"d\", Default" w867 {
          tunnel: [w889 w890] -> w865
          frame "s" {
            w889 = u16 0 items=["Single", "Double"] ("sweep mode")
          }
          frame "d", Default {
            w890 = u16 1 items=["Single", "Double"] ("sweep mode")
          }
        }
        n177 = Fract/Exp String To Number(string=w866) -> (number=w850:dbl[])  [unwired: 3 in, 1 out]
        n178 = String To Path(string=w879) -> (path=w875:path)
        n179 = Index Array(array=w850, index #1=0 ("Index")) -> (element #1=w864:dbl, element #2=w863:dbl, element #3=w862:dbl)  [unwired: 2 in]
        n180 = Delete From Array(array=w850, length=3 ("Length"), index=0 ("Index")) -> (array with subset deleted=w848:dbl[])  [unwired: 1 out]
        n181 = control-ref of="I vs Vg"() -> (w787:refnum<vi>)
        n182 = Bundle By Name(cluster=w856, "Gate Start"=w864, "Gate Stop"=w863, "Gate Step (linear only)"=w862, "Gate Compliance"=w873, "Range mode"=w839, "Range"=w838) -> (w840:T6)
        n183 = Index Array(array=w848, index #1=0 ("Index")) -> (element #1=w859:dbl, element #2=w858:dbl, element #3=w857:dbl)  [unwired: 2 in]
        n184 = call <vilib>:"compatOverwrite.vi"("overwrite (F)"=TRUE) -> ("overwrite?"=w830:T8)
        n185 = Bundle By Name(cluster=w855, "Drain Start"=w859, "Drain Stop"=w858, "Drain Step"=w857, "Drain Compliance"=w874, "Range mode"=w837, "Range"=w836) -> (w841:T7)
        n186 = call "4155C Transfer-FPP v3.0.vi"("VISA resource name in"=w843, "FPP - Source"=w800, "Gate"=w840, "Drain"=w841, "FPP - Drain"=w798, "Timings"=w872, "error in (no error)"=w844, "FPP - Gate"=w799, "FPP - Probe 1"=w797, "sweep mode"=w865, "FPP - Probe 2"=w796, "Panel Controls"=w888) -> ("VG"=w790:dbl[], "Outparams"=w835:T9, "VISA Resource Name out"=w871:refnum<visa-resource-name>, "Vprobe2"=w832:dbl[], "ID"=w789:dbl[], "IG"=w788:dbl[], "Vprobe1"=w831:dbl[], "error out"=w791:errorcluster)  [unwired: 8 in]
        n187 = Unbundle By Name(w835) -> ("V2 Step"=w834:dbl, "V2 Start"=w833:dbl, "Number of points"=w786:i32)
        n188 = call "4155C Split array.vi"("Number of VAR2 steps"=w786, "Y2 data in"=w789, "X data in"=w790, "Y1 data in"=w789, "Y3 data in"=w788, "error in (no error)"=w791) -> ("Array of clusters"=w793:cluster{"Y data in":dbl[], "X data in":dbl[]}[], "error out"=w792:errorcluster)  [unwired: 1 in]
        n189 = call "4155C Config Chart Colours.vi"("Numeric"=w786, "XY Graph 2"=w787) -> ()  [unwired: 6 in]
        n190 = local write "I vs Vg"(w793) -> ()
        n191 = Open/Create/Replace File(file path (use dialog)=w875, error in=w792, operation (0:open)=w830) -> (refnum out=w885:refnum<file>, error out=w886:errorcluster)  [unwired: 3 in, 1 out]
        n192 = call "4155C Make Big 2d array FPP.vi"("1D Var1"=w790, "1d ID"=w789, "1d Vp2"=w832, "1d IG"=w788, "1d Vp1"=w831, "VAR2 START"=w833, "Number of VAR2 steps"=w786, "VAR2 STEP"=w834, "VAR1 Name"="Vg", "Decimal places in header"=i8 1, "VAR2 Name"="Vd") -> ("Header array"=w881:string[], "Data array"=w882:dbl[][])  [unwired: 15 in]
        n193 = call "4155C Write array to file.vi"("Byte Stream File Refnum"=w885, "Header"=w881, "Data Array"=w882, "error in (no error)"=w886) -> ("dup refnum"=w883:refnum<file>, "error out"=w884:errorcluster)  [unwired: 1 in]
        n194 = Close File(refnum=w883, error in=w884) -> (error out=w870:errorcluster)  [unwired: 1 out]
      }
      frame "output" {
        # "Is off"
        # "Is on"
        # "Ig off"
        # "Ig on"
        # "Is min"
        # "Is max"
        # "Ig min"
        # "Ig max"
        # "Id min"
        # "Id max"
        # "Id off"
        # "Id on"
        n195 = local read "Transfer/Output - Probe 4"() -> (w895:u32)
        n196 = Delete From Array(array=w1000, index=0 ("Index")) -> (deleted portion=w998:string, array with subset deleted=w997:string[])  [unwired: 1 in]
        n197 = Bundle By Name(cluster=w907, "Emergency Stop"=w1009) -> (w963:T1)
        n198 = Number To Decimal String(number=w959) -> (decimal integer string=w958:string)  [unwired: 1 in]
        n199 = case shown="\"d\", Default" w998 {
          tunnel: [w1094 w1095] -> w996
          frame "s" {
            w1094 = u16 0 items=["Single", "Double"] ("sweep mode")
          }
          frame "d", Default {
            w1095 = u16 1 items=["Single", "Double"] ("sweep mode")
          }
        }
        n200 = Fract/Exp String To Number(string=w997) -> (number=w982:dbl[])  [unwired: 3 in, 1 out]
        n201 = Concatenate Strings(w1007, w908, w958, w956, "_O_1_C_L.txt" ("Suffix (transfer)")) -> (w1008:string)
        n202 = local read "Transfer/Output - Drain"() -> (w897:u32)
        n203 = local read "Transfer/Output - Source/Common"() -> (w898:u32)
        n204 = VISA Write(VISA resource name=w978, write buffer=":PAGE:CHAN:MODE SWE;" ("write buffer (\"\")"), error in (no error)=w977) -> (VISA resource name out=w975:refnum<visa-resource-name>, error out=w976:errorcluster)  [unwired: 1 out]
        n205 = String To Path(string=w1008) -> (path=w1006:path)
        n206 = local read "Plot output curve extrema vs time"() -> (w905:bool)
        n207 = Index Array(array=w982, index #1=0 ("Index")) -> (element #1=w995:dbl, element #2=w994:dbl, element #3=w993:dbl)  [unwired: 2 in]
        n208 = Delete From Array(array=w982, length=3 ("Length"), index=0 ("Index")) -> (array with subset deleted=w980:dbl[])  [unwired: 1 out]
        n209 = local read "Transfer/Output - Gate"() -> (w896:u32)
        n210 = case shown="True" w905 {
          tunnel: w955 -> [w1011 w1014]
          tunnel: w952 -> [_ w1013]
          tunnel: [w1011 w1012] -> w924
          frame False {
          }
          frame True {
            n211 = Build Array (concatenate)(w1014, w1013) -> (w1012:i32[])
          }
        }
        n212 = Bundle By Name(cluster=w987, "Gate Start"=w995, "Gate Stop"=w994, "Gate Step (linear only)"=w993, "Gate Compliance"=w1004, "Range mode"=w971, "Range"=w970) -> (w972:T6)
        n213 = Index Array(array=w980, index #1=0 ("Index")) -> (element #1=w990:dbl, element #2=w989:dbl, element #3=w988:dbl)  [unwired: 2 in]
        n214 = call <vilib>:"compatOverwrite.vi"("overwrite (F)"=TRUE) -> ("overwrite?"=w962:T8)
        n215 = Bundle By Name(cluster=w986, "Drain Start"=w990, "Drain Stop"=w989, "Drain Step"=w988, "Drain Compliance"=w1005, "Range mode"=w969, "Range"=w968) -> (w973:T7)
        n216 = call "4155C Output v3.0.vi"("VISA resource name in"=w975, "Source/Common"=w898, 2:"Gate"=w972, 3:"Drain"=w973, 4:"Drain"=w897, "Timings"=w1003, "error in (no error)"=w976, 7:"Probe 4"=w904, 8:"Gate"=w896, 9:"Probe 4"=w895, "sweep mode"=w996, "Panel controls"=w963, "Standby"=w899) -> ("VD"=w961:dbl[], "Outparams"=w967:T9, "VISA Resource Name out"=w1002:refnum<visa-resource-name>, "IS"=w934:dbl[], "ID"=w935:dbl[], "IG"=w933:dbl[], "error out"=w953:errorcluster, "Probe 4"=w964:dbl[])  [unwired: 7 in]
        n217 = Unbundle By Name(w967) -> ("V2 Step"=w966:dbl, "V2 Start"=w965:dbl, "Number of points"=w922:i32)
        n218 = call "4155C Split array.vi"("Number of VAR2 steps"=w922, "Y2 data in"=w935, "X data in"=w961, "Y1 data in"=w934, "Y3 data in"=w933, "error in (no error)"=w953) -> ("Array of clusters"=w954:cluster{"Y data in":dbl[], "X data in":dbl[]}[], "error out"=w910:errorcluster)  [unwired: 1 in]
        n219 = case shown="True" "Plot output curve extrema vs time" {
          tunnel: w960 -> [w1018 w1093]
          tunnel: w951 -> [w1017 w1088]
          tunnel: w937 -> [w1023 w1084]
          tunnel: w936 -> [w1024 w1083]
          tunnel: w935 -> [_ w1080]
          tunnel: w934 -> [_ w1078]
          tunnel: w933 -> [_ w1077]
          tunnel: w932 -> [w1016 w1073]
          tunnel: w931 -> [w1015 w1072]
          tunnel: w930 -> [w1020 w1069]
          tunnel: w929 -> [w1019 w1068]
          tunnel: w928 -> [w1022 w1065]
          tunnel: w927 -> [w1021 w1064]
          tunnel: w926 -> [w1026 w1061]
          tunnel: w925 -> [w1025 w1060]
          tunnel: w924 -> [_ w1053]
          tunnel: [w1020 w1048] -> w923
          tunnel: w922 -> [_ w1047]
          tunnel: [w1019 w1046] -> w921
          tunnel: [w1018 w1045] -> w920
          tunnel: [w1017 w1044] -> w919
          tunnel: [w1016 w1043] -> w918
          tunnel: [w1015 w1042] -> w917
          tunnel: [w1026 w1041] -> w916
          tunnel: [w1025 w1040] -> w915
          tunnel: [w1024 w1039] -> w914
          tunnel: [w1023 w1038] -> w913
          tunnel: [w1022 w1037] -> w912
          tunnel: [w1021 w1036] -> w911
          tunnel: w910 -> [w1027 w1035]
          tunnel: [w1027 w1031] -> w909
          frame False {
          }
          frame True {
            # "Adjusts graph colors."
            # "Adjusts graph colors."
            # "Ion will be the middle element of the array. The calculation of the index is done only once, since Is, Id, and Ig have the same dimensions."
            # "abs(Ig)"
            # "abs(Is)"
            # "Y1: Is\nY2: Id\nY3: Ig"
            # "abs(Id)"
            # "Adjusts graph colors."
            # "Adjusts graph colors."
            # "Adjusts graph colors."
            n220 = Absolute Value(x=w1078) -> (abs(x)=w1063:dbl[])
            n221 = Absolute Value(x=w1080) -> (abs(x)=w1079:dbl[])
            n222 = Absolute Value(x=w1077) -> (abs(x)=w1066:dbl[])
            n223 = Array Size(array=w1079) -> (size(s)=w1087:i32)
            n224 = Divide(x=w1087, y=2) -> (x/y=w1030:dbl)
            n225 = Subtract(x=w1030, y=1) -> (x-y=w1029:dbl)
            n226 = Array Max & Min(array=w1063) -> (max value=w1070:dbl, min value=w1071:dbl)  [unwired: 2 out]
            n227 = Array Max & Min(array=w1079) -> (max value=w1092:dbl, min value=w1076:dbl)  [unwired: 2 out]
            n228 = Array Max & Min(array=w1066) -> (max value=w1075:dbl, min value=w1074:dbl)  [unwired: 2 out]
            n229 = Index Array(array=w1063, index=w1029) -> (element=w1054:dbl)
            n230 = Index Array(array=w1063, index=0) -> (element=w1055:dbl)
            n231 = Index Array(array=w1079, index=w1029) -> (element=w1056:dbl)
            n232 = Index Array(array=w1079, index=0) -> (element=w1057:dbl)
            n233 = Index Array(array=w1066, index=w1029) -> (element=w1059:dbl)
            n234 = Index Array(array=w1066, index=0) -> (element=w1058:dbl)
            n235 = local write "Ig max"(w1075) -> ()
            n236 = local write "Ig min"(w1074) -> ()
            n237 = local write "Is max"(w1070) -> ()
            n238 = local write "Is min"(w1071) -> ()
            n239 = local write "Id max"(w1092) -> ()
            n240 = local write "Id min"(w1076) -> ()
            n241 = Build Array (concatenate)(w1069, w1070) -> (w1048:dbl[])
            n242 = Build Array (concatenate)(w1068, w1071) -> (w1046:dbl[])
            n243 = local write "Is off"(w1055) -> ()
            n244 = local write "Is on"(w1054) -> ()
            n245 = Build Array (concatenate)(w1093, w1092) -> (w1045:dbl[])
            n246 = Build Array (concatenate)(w1088, w1076) -> (w1044:dbl[])
            n247 = Build Array (concatenate)(w1073, w1075) -> (w1043:dbl[])
            n248 = Build Array (concatenate)(w1072, w1074) -> (w1042:dbl[])
            n249 = Build Array (concatenate)(w1061, w1054) -> (w1041:dbl[])
            n250 = Build Array (concatenate)(w1060, w1055) -> (w1040:dbl[])
            n251 = Build Array (concatenate)(w1083, w1056) -> (w1039:dbl[])
            n252 = Build Array (concatenate)(w1084, w1057) -> (w1038:dbl[])
            n253 = Build Array (concatenate)(w1065, w1059) -> (w1037:dbl[])
            n254 = Build Array (concatenate)(w1064, w1058) -> (w1036:dbl[])
            n255 = local write "Ig off"(w1058) -> ()
            n256 = local write "Ig on"(w1059) -> ()
            n257 = local write "Id off"(w1057) -> ()
            n258 = local write "Id on"(w1056) -> ()
            n259 = control-ref of="Imax vs time"() -> (w1082:refnum<vi>)
            n260 = control-ref of="Imin vs time"() -> (w1081:refnum<vi>)
            n261 = control-ref of="Ion vs time"() -> (w1050:refnum<vi>)
            n262 = control-ref of="Ioff vs time"() -> (w1049:refnum<vi>)
            n263 = control-ref of="I vs Vg"() -> (w1091:refnum<vi>)
            n264 = call "4155C Split array.vi"("Number of VAR2 steps"=w1047, "Y2 data in"=w1039, "X data in"=w1053, "Y1 data in"=w1041, "Y3 data in"=w1037, "error in (no error)"=w1035) -> ("Array of clusters"=w1051:cluster{"Y data in":dbl[], "X data in":dbl[]}[], "error out"=w1034:errorcluster)  [unwired: 1 in]
            n265 = call "4155C Split array.vi"("Number of VAR2 steps"=w1047, "Y2 data in"=w1038, "X data in"=w1053, "Y1 data in"=w1040, "Y3 data in"=w1036, "error in (no error)"=w1034) -> ("Array of clusters"=w1052:cluster{"Y data in":dbl[], "X data in":dbl[]}[], "error out"=w1033:errorcluster)  [unwired: 1 in]
            n266 = call "4155C Split array.vi"("Number of VAR2 steps"=w1047, "Y2 data in"=w1045, "X data in"=w1053, "Y1 data in"=w1048, "Y3 data in"=w1043, "error in (no error)"=w1033) -> ("Array of clusters"=w1090:cluster{"Y data in":dbl[], "X data in":dbl[]}[], "error out"=w1032:errorcluster)  [unwired: 1 in]
            n267 = call "4155C Split array.vi"("Number of VAR2 steps"=w1047, "Y2 data in"=w1044, "X data in"=w1053, "Y1 data in"=w1046, "Y3 data in"=w1042, "error in (no error)"=w1032) -> ("Array of clusters"=w1089:cluster{"Y data in":dbl[], "X data in":dbl[]}[], "error out"=w1031:errorcluster)  [unwired: 1 in]
            n268 = call "4155C Config Chart Colours.vi"("Numeric"=w1047, "XY Graph 2"=w1082) -> ()  [unwired: 6 in]
            n269 = call "4155C Config Chart Colours.vi"("Numeric"=w1047, "XY Graph 2"=w1081) -> ()  [unwired: 6 in]
            n270 = call "4155C Config Chart Colours.vi"("Numeric"=w1047, "XY Graph 2"=w1050) -> ()  [unwired: 6 in]
            n271 = call "4155C Config Chart Colours.vi"("Numeric"=w1047, "XY Graph 2"=w1049) -> ()  [unwired: 6 in]
            n272 = call "4155C Config Chart Colours.vi"("Numeric"=w1047, "XY Graph 2"=w1091) -> ()  [unwired: 6 in]
            n273 = local write "Imax vs time"(w1090) -> ()
            n274 = local write "Imin vs time"(w1089) -> ()
            n275 = local write "Ion vs time"(w1051) -> ()
            n276 = local write "Ioff vs time"(w1052) -> ()
          }
        }
        n277 = local write "I vs Vd"(w954) -> ()
        n278 = Open/Create/Replace File(file path (use dialog)=w1006, error in=w909, operation (0:open)=w962) -> (refnum out=w949:refnum<file>, error out=w947:errorcluster)  [unwired: 3 in, 1 out]
        n279 = call "4155C Make Big 2d array.vi"("1D Var1"=w961, "1d IS"=w934, "1d ID"=w935, "1d IG"=w933, "1d SMU4"=w964, "SMU4"=w904, "VAR2 START"=w965, "Number of VAR2 steps"=w922, "VAR2 STEP"=w966, "VAR1 Name"="Vd", "Decimal places in header"=i8 1, "VAR2 Name"="Vg") -> ("Header array"=w950:string[], "Data array"=w948:dbl[][])  [unwired: 14 in]
        n280 = call "4155C Write array to file.vi"("Byte Stream File Refnum"=w949, "Header"=w950, "Data Array"=w948, "error in (no error)"=w947) -> ("dup refnum"=w946:refnum<file>, "error out"=w945:errorcluster)  [unwired: 1 in]
        n281 = Close File(refnum=w946, error in=w945) -> (error out=w1001:errorcluster)  [unwired: 1 out]
      }
      frame "output-fpp" {
        # "Adjusts graph colors."
        # "Adjusts graph colors."
        # "Y1 = Vp2\nY2 = Y3 = Vp1"
        n282 = local read "FPP - Source"() -> (w1116:u32)
        n283 = local read "FPP - Drain"() -> (w1115:u32)
        n284 = local read "FPP - Gate"() -> (w1114:u32)
        n285 = local read "FPP - Probe 1"() -> (w1113:u32)
        n286 = local read "FPP - Probe 2"() -> (w1112:u32)
        n287 = Number To Decimal String(number=w1142) -> (decimal integer string=w1189:string)  [unwired: 1 in]
        n288 = Bundle By Name(cluster=w1166, "Emergency Stop"=w1192) -> (w1202:T1)
        n289 = Delete From Array(array=w1181, index=0 ("Index")) -> (deleted portion=w1179:string, array with subset deleted=w1178:string[])  [unwired: 1 in]
        n290 = VISA Write(VISA resource name=w1157, write buffer=":PAGE:CHAN:MODE SWE;" ("write buffer (\"\")"), error in (no error)=w1154) -> (VISA resource name out=w1156:refnum<visa-resource-name>, error out=w1155:errorcluster)  [unwired: 1 out]
        n291 = Concatenate Strings(w1188, "-outputfpp-" ("Substring"), w1189, w1141, ".txt" ("Substring")) -> (w1191:string)
        n292 = case shown="\"d\", Default" w1179 {
          tunnel: [w1203 w1204] -> w1177
          frame "s" {
            w1203 = u16 0 items=["Single", "Double"] ("sweep mode")
          }
          frame "d", Default {
            w1204 = u16 1 items=["Single", "Double"] ("sweep mode")
          }
        }
        n293 = Fract/Exp String To Number(string=w1178) -> (number=w1160:dbl[])  [unwired: 3 in, 1 out]
        n294 = String To Path(string=w1191) -> (path=w1187:path)
        n295 = Index Array(array=w1160, index #1=0 ("Index")) -> (element #1=w1176:dbl, element #2=w1175:dbl, element #3=w1174:dbl)  [unwired: 2 in]
        n296 = Delete From Array(array=w1160, length=3 ("Length"), index=0 ("Index")) -> (array with subset deleted=w1159:dbl[])  [unwired: 1 out]
        n297 = control-ref of="I vs Vd"() -> (w1100:refnum<vi>)
        n298 = control-ref of="Vp vs Vg (FPP)"() -> (w1099:refnum<vi>)
        n299 = Bundle By Name(cluster=w1168, "Gate Start"=w1176, "Gate Stop"=w1175, "Gate Step (linear only)"=w1174, "Gate Compliance"=w1185, "Range mode"=w1152, "Range"=w1151) -> (w1201:T6)
        n300 = Index Array(array=w1159, index #1=0 ("Index")) -> (element #1=w1171:dbl, element #2=w1170:dbl, element #3=w1169:dbl)  [unwired: 2 in]
        n301 = call <vilib>:"compatOverwrite.vi"("overwrite (F)"=TRUE) -> ("overwrite?"=w1146:T8)
        n302 = Bundle By Name(cluster=w1167, "Drain Start"=w1171, "Drain Stop"=w1170, "Drain Step"=w1169, "Drain Compliance"=w1186, "Range mode"=w1150, "Range"=w1153) -> (w1200:T7)
        n303 = call "4155C Output-FPP v3.0.vi"("VISA resource name in"=w1156, "FPP - Source"=w1116, "Gate"=w1201, "Drain"=w1200, "FPP - Drain"=w1115, "Timings"=w1184, "error in (no error)"=w1155, "FPP - Gate"=w1114, "FPP - Probe 1"=w1113, "sweep mode"=w1177, "FPP - Probe 2"=w1112, "Panel controls"=w1202) -> ("VD"=w1103:dbl[], "Outparams"=w1148:T9, "VISA Resource Name out"=w1183:refnum<visa-resource-name>, "Vprobe2"=w1102:dbl[], "ID"=w1106:dbl[], "IG"=w1105:dbl[], "Vprobe1"=w1101:dbl[], "error out"=w1107:errorcluster)  [unwired: 8 in]
        n304 = Unbundle By Name(w1148) -> ("V2 Step"=w1149:dbl, "V2 Start"=w1147:dbl, "Number of points"=w1098:i32)
        n305 = call "4155C Split array.vi"("Number of VAR2 steps"=w1098, "Y2 data in"=w1106, "X data in"=w1103, "Y1 data in"=w1106, "Y3 data in"=w1105, "error in (no error)"=w1107) -> ("Array of clusters"=w1109:cluster{"Y data in":dbl[], "X data in":dbl[]}[], "error out"=w1108:errorcluster)  [unwired: 1 in]
        n306 = call "4155C Split array.vi"("Number of VAR2 steps"=w1098, "Y2 data in"=w1101, "X data in"=w1103, "Y1 data in"=w1102, "Y3 data in"=w1101) -> ("Array of clusters"=w1104:cluster{"Y data in":dbl[], "X data in":dbl[]}[])  [unwired: 2 in, 1 out]
        n307 = call "4155C Config Chart Colours.vi"("Numeric"=w1098, "XY Graph 2"=w1100) -> ()  [unwired: 6 in]
        n308 = call "4155C Config Chart Colours.vi"("Numeric"=w1098, "XY Graph 2"=w1099) -> ()  [unwired: 6 in]
        n309 = local write "I vs Vd"(w1109) -> ()
        n310 = local write "Vp vs Vg (FPP)"(w1104) -> ()
        n311 = Open/Create/Replace File(file path (use dialog)=w1187, error in=w1108, operation (0:open)=w1146) -> (refnum out=w1197:refnum<file>, error out=w1198:errorcluster)  [unwired: 3 in, 1 out]
        n312 = call "4155C Make Big 2d array FPP.vi"("1D Var1"=w1103, "1d ID"=w1106, "1d Vp2"=w1102, "1d IG"=w1105, "1d Vp1"=w1101, "VAR2 START"=w1147, "Number of VAR2 steps"=w1098, "VAR2 STEP"=w1149, "VAR1 Name"="Vd", "Decimal places in header"=i8 1, "VAR2 Name"="Vg") -> ("Header array"=w1193:string[], "Data array"=w1194:dbl[][])  [unwired: 15 in]
        n313 = call "4155C Write array to file.vi"("Byte Stream File Refnum"=w1197, "Header"=w1193, "Data Array"=w1194, "error in (no error)"=w1198) -> ("dup refnum"=w1195:refnum<file>, "error out"=w1196:errorcluster)  [unwired: 1 in]
        n314 = Close File(refnum=w1195, error in=w1196) -> (error out=w1182:errorcluster)  [unwired: 1 out]
      }
      frame "itime" {
        n315 = Delete From Array(array=w1216, index=1) -> (deleted portion=w1215:string)  [unwired: 1 in, 1 out]
        n316 = Delete From Array(array=w1216, index=0 ("Index")) -> (deleted portion=w1250:string)  [unwired: 1 in, 1 out]
        n317 = Fract/Exp String To Number(string=w1215) -> (number=w1214:dbl)  [unwired: 3 in, 1 out]
        n318 = case shown="\"l\"" w1250 {
          tunnel: w1249 -> [w1255 w1257 w1261]
          tunnel: [w1254 w1256 w1260] -> w1242
          tunnel: w1214 -> [w1252 _ w1259]
          frame "s" {
            w1253 = u32 0 items=["short  ", "medium  ", "long  "] ("integration time 2")
            n319 = Bundle By Name(cluster=w1255, "integration time"=w1253, "Short/Long integration time"=w1252) -> (w1254:T5)
          }
          frame "m", Default {
            w1258 = u32 1 items=["short  ", "medium  ", "long  "] ("integration time 2")
            n320 = Bundle By Name(cluster=w1257, "integration time"=w1258) -> (w1256:T5)
          }
          frame "l" {
            w1262 = u32 2 items=["short  ", "medium  ", "long  "] ("integration time 2")
            n321 = Bundle By Name(cluster=w1261, "integration time"=w1262, "Short/Long integration time"=w1259) -> (w1260:T5)
          }
        }
      }
      frame "pulsed" {
        n322 = Delete From Array(array=w1305, index=0 ("Index")) -> (deleted portion=w1306:string, array with subset deleted=w1293:string[])  [unwired: 1 in]
        n323 = case shown="\"on\", Default" w1306 {
          tunnel: w1304 -> [w1316 w1319]
          tunnel: [w1315 w1318] -> w1297
          tunnel: w1293 -> [w1313 _]
          frame "on", Default {
            w1314 = u16 1 items=["Continuous", "Pulsed"] ("sweep method")
            n324 = Fract/Exp String To Number(string=w1313) -> (number=w1311:dbl[])  [unwired: 3 in, 1 out]
            n325 = Index Array(array=w1311, index #1=0 ("Index")) -> (element #1=w1310:dbl, element #2=w1309:dbl, element #3=w1308:dbl)  [unwired: 2 in]
            n326 = Bundle By Name(cluster=w1316, "sweep method"=w1314, "Pulse period"=w1310, "Base voltage"=w1309, "Pulse width"=w1308) -> (w1315:T5)
          }
          frame "off" {
            w1317 = u16 0 items=["Continuous", "Pulsed"] ("sweep method")
            n327 = Bundle By Name(cluster=w1319, "sweep method"=w1317) -> (w1318:T5)
          }
        }
      }
      frame "gaterangemode" {
        n328 = Delete From Array(array=w1360, index=0 ("Index")) -> (deleted portion=w1361:string)  [unwired: 1 in, 1 out]
        n329 = case shown="\"f\"" w1361 {
          tunnel: [w1363 w1364 w1365] -> w1350
          frame "a", Default {
            w1363 = u16 0 items=["Auto", "Limited", "Fixed"] ("Gate Range\nmode 2")
          }
          frame "f" {
            w1364 = u16 2 items=["Auto", "Limited", "Fixed"] ("Gate Range\nmode 2")
          }
          frame "l" {
            w1365 = u16 1 items=["Auto", "Limited", "Fixed"] ("Gate Range\nmode 2")
          }
        }
      }
      frame "gaterange" {
        (unwired) u8 11 items=["10fA  ", "100fA  ", "1nA  ", "10nA", "100nA", "1uA", "10uA", "100uA", "1mA", "10mA", "100mA", "1A"] ("Gate Range 2")
        n330 = Delete From Array(array=w1413, index=0 ("Index")) -> (deleted portion=w1403:string)  [unwired: 1 in, 1 out]
        n331 = Scan Value(string=w1403, format string="") -> (value=w1401:dbl)  [unwired: 1 in, 1 out]
        n332 = Logarithm Base 10(1:w1401) -> (0:w1400:dbl)
        n333 = Round To Nearest(number=w1400) -> (nearest integer value=w1399:dbl)
        n334 = Add(x=w1399, y=11.0) -> (x+y=w1397:dbl)
        n335 = To Unsigned Byte Integer(number=w1397) -> (unsigned 8bit integer=w1396:u8)
      }
      frame "drainrange" {
        (unwired) u8 11 items=["10fA  ", "100fA  ", "1nA  ", "10nA", "100nA", "1uA", "10uA", "100uA", "1mA", "10mA", "100mA", "1A"] ("Gate Range 2")
        n336 = Delete From Array(array=w1462, index=0 ("Index")) -> (deleted portion=w1453:string)  [unwired: 1 in, 1 out]
        n337 = Scan Value(string=w1453, format string="") -> (value=w1451:dbl)  [unwired: 1 in, 1 out]
        n338 = Logarithm Base 10(1:w1451) -> (0:w1450:dbl)
        n339 = Round To Nearest(number=w1450) -> (nearest integer value=w1449:dbl)
        n340 = Add(x=w1449, y=11.0) -> (x+y=w1447:dbl)
        n341 = To Unsigned Byte Integer(number=w1447) -> (unsigned 8bit integer=w1446:u8)
      }
      frame "drainrangemode" {
        n342 = Delete From Array(array=w1504, index=0 ("Index")) -> (deleted portion=w1505:string)  [unwired: 1 in, 1 out]
        n343 = case shown="\"f\"" w1505 {
          tunnel: [w1507 w1508 w1509] -> w1494
          frame "a", Default {
            w1507 = u16 0 items=["Auto", "Limited", "Fixed"] ("Gate Range\nmode 2")
          }
          frame "f" {
            w1508 = u16 2 items=["Auto", "Limited", "Fixed"] ("Gate Range\nmode 2")
          }
          frame "l" {
            w1509 = u16 1 items=["Auto", "Limited", "Fixed"] ("Gate Range\nmode 2")
          }
        }
      }
      frame "Error", Default {
      }
      frame "logfile" {
        n344 = Number To Decimal String(number=w1580) -> (decimal integer string=w1615:string)  [unwired: 1 in]
        n345 = Concatenate Strings(w1614, "logfile" ("Substring"), w1615, w1578, ".txt" ("Substring")) -> (w1612:string)
        n346 = String To Path(string=w1612) -> (path=w1585:path)
        n347 = Unbundle(w1611) -> ("integration time"=w1610:u32, "Short/Long integration time"=w1609:dbl, "hold time (sec)"=w1608:dbl, "delay time (sec)"=w1607:dbl, "Step Time (0 disables)"=w1606:dbl, "sweep method"=w1605:u16, "Pulse period"=w1604:dbl, "Base voltage"=w1603:dbl, "Pulse width"=w1602:dbl)
        n348 = Build Array(w1610, w1609, w1608, w1607, w1606, w1605, w1604, w1603, w1602, w1596, w1597, w1598, w1599, w1600, w1601) -> (w1589:dbl[])
        n349 = Insert Into Array(array=dbl[][] [] ("Input Array"), new element=w1589) -> (w1588:dbl[][])  [unwired: 2 in]
        n350 = call <vilib>:"compatOverwrite.vi"("overwrite (F)"=TRUE) -> ("overwrite?"=w1583:T8)
        n351 = Open/Create/Replace File(file path (use dialog)=w1585, error in=w1587, operation (0:open)=w1583) -> (refnum out=w1593:refnum<file>, error out=w1592:errorcluster)  [unwired: 3 in, 1 out]
        n352 = call "4155C Write array to file.vi"("Byte Stream File Refnum"=w1593, "Header"=string[] ["Int Time", "Short/Long Itime", "Hold time", "Delay time", "Step time", "Sweep method", "Pulse period", "Base Voltage", "Pulse width", "Drain compliance", "Gate compliance", "Gate range mode", "Gate range", "S/D range mode", "S/D range"], "Data Array"=w1588, "error in (no error)"=w1592) -> ("dup refnum"=w1595:refnum<file>, "error out"=w1594:errorcluster)  [unwired: 1 in]
        n353 = Close File(refnum=w1595, error in=w1594) -> (error out=w1586:errorcluster)  [unwired: 1 out]
      }
      frame "sample" {
        w1657 = 1
        # "The suffix is Vg_Vd_Time."
        # "Add a time offset (elapsed time) to the time axis."
        # "Adjusts graph colors."
        n354 = Number To Decimal String(number=w1691) -> (decimal integer string=w1729:string)  [unwired: 1 in]
        n355 = local read "Sample - Drain"() -> (w1625:u32)
        n356 = Fract/Exp String To Number(string=w1727) -> (number=w1695:dbl[])  [unwired: 3 in, 1 out]
        n357 = Index Array(array=w1695, index=0 ("Index")) -> (element=w1649:dbl)
        n358 = Index Array(array=w1695, index=2 ("Index")) -> (element=w1723:dbl)
        n359 = Index Array(array=w1695, index=3 ("Index")) -> (element=w1646:dbl)
        n360 = Index Array(array=w1695, index=4 ("Index")) -> (element=w1694:dbl)
        n361 = Index Array(array=w1695, index=1 ("Index")) -> (element=w1651:dbl)
        n362 = local read "Sample - Probe 4"() -> (w1628:u32)
        n363 = local read "Sample - Source/Common"() -> (w1626:u32)
        n364 = local read "Time Units"() -> (w1621:u16)
        n365 = local read "Sample - Gate"() -> (w1627:u32)
        n366 = call "4155C Config Sampling Measurements v3.0.vi"("VISA session"=w1732, "Num Points"=w1723, "Sample - Drain"=w1625, "Display on/off"=TRUE, "Gate Compliance"=w1710, "Sampling interval"=w1694, "Sample - Source/Common"=w1626, "Sample - Probe 4"=w1628, "Drain Compliance"=w1730, "Standby"=w1629, "error in (no error)"=w1731, "Timings"=w1702, "Sample - Gate"=w1627, "Sample time"=w1646) -> ("dup VISA resource name"=w1734:refnum<visa-resource-name>, "error out"=w1733:errorcluster)
        n367 = local read "Plot sample extrema vs time"() -> (w1659:bool)
        n368 = Number To Decimal String(number=w1651) -> (decimal integer string=w1652:string)  [unwired: 1 in]
        n369 = Number To Decimal String(number=w1649) -> (decimal integer string=w1648:string)  [unwired: 1 in]
        n370 = Number To Decimal String(number=w1646) -> (decimal integer string=w1645:string)  [unwired: 1 in]
        n371 = call "4155C Take Sample v3.0.vi"("VISA resource name in"=w1734, "Emergency Stop"=w1707, "Sample - Gate"=w1627, "Vg"=w1649, "Sample - Drain"=w1625, "Vd"=w1651, "error in (no error)"=w1733) -> ("Time"=w1622:dbl[], "VISA Resource Name out"=w1704:refnum<visa-resource-name>, "Ig"=w1639:dbl[], "Id"=w1640:dbl[], "Is"=w1641:dbl[], "error out"=w1667:errorcluster)  [unwired: 3 in]
        n372 = Insert Into Array(array=w1633, new element=w1640) -> (w1636:dbl[])  [unwired: 1 in]
        n373 = case shown="2" w1621 {
          tunnel: [w1737 w1738 w1741] -> w1624
          tunnel: w1622 -> [w1736 w1738 w1740]
          frame 2 {
            n374 = Divide(x=w1736, y=3600.0) -> (x/y=w1737:dbl[])
          }
          frame 0, Default {
          }
          frame 1 {
            n375 = Divide(x=w1740, y=60.0) -> (x/y=w1741:dbl[])
          }
        }
        n376 = Insert Into Array(array=w1632, new element=w1641) -> (w1638:dbl[])  [unwired: 1 in]
        n377 = Insert Into Array(array=w1634, new element=w1639) -> (w1637:dbl[])  [unwired: 1 in]
        n378 = Concatenate Strings(w1652, "_" ("Substring"), w1648, "_" ("Substring"), w1645, ".txt" ("Substring")) -> (w1643:string)
        n379 = Concatenate Strings(w1654, w1653, w1729, w1689, "_S_" ("Substring"), w1643) -> (w1728:string)
        n380 = String To Path(string=w1728) -> (path=w1713:path)
        n381 = Add(x=w1624, y=w1623) -> (x+y=w1642:dbl[])
        n382 = Insert Into Array(array=w1631, new element=w1642) -> (w1635:dbl[])  [unwired: 1 in]
        n383 = case shown="True" w1659 {
          tunnel: w1642 -> [_ w1744]
          tunnel: [w1742 w1745] -> w1656
          tunnel: w1660 -> [w1742 w1743]
          frame False {
          }
          frame True {
            n384 = Insert Into Array(array=w1743, new element=w1744) -> (w1745:i32[])  [unwired: 1 in]
          }
        }
        n385 = case shown="True" "Plot sample extrema vs time" {
          tunnel: w1641 -> [_ w1774]
          tunnel: w1640 -> [_ w1775]
          tunnel: w1639 -> [_ w1776]
          tunnel: [w1752 w1762] -> w1630
          tunnel: w1667 -> [w1752 w1767]
          tunnel: w1673 -> [w1751 w1779]
          tunnel: w1672 -> [w1750 w1778]
          tunnel: w1671 -> [w1749 w1780]
          tunnel: w1670 -> [w1748 w1777]
          tunnel: w1669 -> [w1747 w1782]
          tunnel: w1668 -> [w1746 w1781]
          tunnel: [w1751 w1766] -> w1666
          tunnel: [w1750 w1760] -> w1665
          tunnel: [w1749 w1764] -> w1664
          tunnel: [w1748 w1759] -> w1663
          tunnel: [w1747 w1765] -> w1662
          tunnel: [w1746 w1758] -> w1661
          tunnel: w1656 -> [_ w1756]
          frame False {
          }
          frame True {
            w1761 = 1
            # "Number of VAR2 steps is 1."
            # "abs(Ig)"
            # "abs(Is)"
            # "abs(Id)"
            # "Adjusts graph colors."
            n386 = Absolute Value(x=w1776) -> (abs(x)=w1753:dbl[])
            n387 = Absolute Value(x=w1775) -> (abs(x)=w1754:dbl[])
            n388 = Absolute Value(x=w1774) -> (abs(x)=w1755:dbl[])
            n389 = Array Max & Min(array=w1755) -> (max value=w1773:dbl, min value=w1770:dbl)  [unwired: 2 out]
            n390 = Array Max & Min(array=w1754) -> (max value=w1772:dbl, min value=w1769:dbl)  [unwired: 2 out]
            n391 = Array Max & Min(array=w1753) -> (max value=w1771:dbl, min value=w1768:dbl)  [unwired: 2 out]
            n392 = local write "Id max"(w1772) -> ()
            n393 = local write "Id min"(w1769) -> ()
            n394 = local write "Ig max"(w1771) -> ()
            n395 = local write "Ig min"(w1768) -> ()
            n396 = Insert Into Array(array=w1782, new element=w1753) -> (w1765:dbl[])  [unwired: 1 in]
            n397 = Insert Into Array(array=w1781, new element=w1753) -> (w1758:dbl[])  [unwired: 1 in]
            n398 = local write "Is max"(w1773) -> ()
            n399 = local write "Is min"(w1770) -> ()
            n400 = Insert Into Array(array=w1780, new element=w1754) -> (w1764:dbl[])  [unwired: 1 in]
            n401 = Insert Into Array(array=w1777, new element=w1754) -> (w1759:dbl[])  [unwired: 1 in]
            n402 = Insert Into Array(array=w1779, new element=w1755) -> (w1766:dbl[])  [unwired: 1 in]
            n403 = Insert Into Array(array=w1778, new element=w1755) -> (w1760:dbl[])  [unwired: 1 in]
            n404 = control-ref of="Imax vs time"() -> (w1783:refnum<vi>)
            n405 = call "4155C Config Chart Colours.vi"("Numeric"=w1761, "XY Graph 2"=w1783) -> ()  [unwired: 6 in]
            n406 = call "4155C Split array.vi"("Number of VAR2 steps"=w1761, "Y2 data in"=w1764, "X data in"=w1756, "Y1 data in"=w1766, "Y3 data in"=w1765, "error in (no error)"=w1767) -> ("Array of clusters"=w1784:cluster{"Y data in":dbl[], "X data in":dbl[]}[], "error out"=w1763:errorcluster)  [unwired: 1 in]
            n407 = call "4155C Split array.vi"("Number of VAR2 steps"=w1761, "Y2 data in"=w1759, "X data in"=w1756, "Y1 data in"=w1760, "Y3 data in"=w1758, "error in (no error)"=w1763) -> ("Array of clusters"=w1757:cluster{"Y data in":dbl[], "X data in":dbl[]}[], "error out"=w1762:errorcluster)  [unwired: 1 in]
            n408 = local write "Imax vs time"(w1784) -> ()
            n409 = local write "Imin vs time"(w1757) -> ()
          }
        }
        n410 = control-ref of="I vs time (Bias Stress)"() -> (w1655:refnum<vi>)
        n411 = call "4155C Split array.vi"("Number of VAR2 steps"=w1657, "Y2 data in"=w1636, "X data in"=w1635, "Y1 data in"=w1638, "Y3 data in"=w1637) -> ("Array of clusters"=w1658:cluster{"Y data in":dbl[], "X data in":dbl[]}[])  [unwired: 2 in, 1 out]
        n412 = local write "I vs time (Bias Stress)"(w1658) -> ()
        n413 = call "4155C Config Chart Colours.vi"("Numeric"=w1657, "XY Graph 2"=w1655) -> ()  [unwired: 6 in]
        n414 = Insert Into Array(array=dbl[][] [] ("Input Array"), new element=w1642) -> (w1717:dbl[][])  [unwired: 2 in]
        n415 = Insert Into Array(array=w1717, new element=w1639) -> (w1716:dbl[][])  [unwired: 2 in]
        n416 = VISA Write(VISA resource name=w1704, write buffer=":DISP ON" ("write buffer (\"\")"), error in (no error)=w1630) -> (VISA resource name out=w1703:refnum<visa-resource-name>, error out=w1705:errorcluster)  [unwired: 1 out]
        n417 = Insert Into Array(array=w1716, new element=w1640) -> (w1715:dbl[][])  [unwired: 2 in]
        n418 = Insert Into Array(array=w1715, new element=w1641) -> (w1709:dbl[][])  [unwired: 2 in]
        n419 = call <vilib>:"compatOverwrite.vi"("overwrite (F)"=TRUE) -> ("overwrite?"=w1692:T8)
        n420 = Open/Create/Replace File(file path (use dialog)=w1713, error in=w1705, operation (0:open)=w1692) -> (refnum out=w1720:refnum<file>, error out=w1719:errorcluster)  [unwired: 3 in, 1 out]
        n421 = Transpose 2D Array(2D array=w1709) -> (transposed array=w1708:dbl[][])
        n422 = call "4155C Write array to file.vi"("Byte Stream File Refnum"=w1720, "Header"=string[] ["Time /Units", "Ig /A", "Id /A", "Is /A"], "Data Array"=w1708, "error in (no error)"=w1719) -> ("dup refnum"=w1722:refnum<file>, "error out"=w1721:errorcluster)  [unwired: 1 in]
        n423 = Close File(refnum=w1722, error in=w1721) -> (error out=w1711:errorcluster)  [unwired: 1 out]
      }
      frame "samplei" {
        w1797 = 1
        # "Adjusts graph colors."
        # "Add a time offset (elapsed time) to the time axis."
        n424 = Number To Decimal String(number=w1838) -> (decimal integer string=w1886:string)  [unwired: 1 in]
        n425 = local read "Sample I - Probe 4 (Disabled)"() -> (w1812:u32)
        n426 = local read "Sample I - Source/Common"() -> (w1809:u32)
        n427 = Concatenate Strings(w1867, "-samplei-" ("Substring"), w1886, w1837, ".txt" ("Substring")) -> (w1884:string)
        n428 = Fract/Exp String To Number(string=w1883) -> (number=w1852:dbl[])  [unwired: 3 in, 1 out]
        n429 = String To Path(string=w1884) -> (path=w1870:path)
        n430 = Index Array(array=w1852, index=4 ("Index")) -> (element=w1846:dbl)
        n431 = Index Array(array=w1852, index=3 ("Index")) -> (element=w1847:dbl)
        n432 = Index Array(array=w1852, index=1 ("Index")) -> (element=w1849:dbl)
        n433 = Index Array(array=w1852, index=0 ("Index")) -> (element=w1850:dbl)
        n434 = local read "Sample I - Drain/Gate"() -> (w1811:u32)
        n435 = Index Array(array=w1852, index=2 ("Index")) -> (element=w1848:dbl)
        n436 = local read "Plot sample extrema vs time"() -> (w1806:bool)
        n437 = local read "Time Units"() -> (w1803:u16)
        n438 = local read "Sample I - Probe 3 (Disabled)"() -> (w1810:u32)
        n439 = call "4155C Config SamplingI Measurements v3.0.vi"("VISA session"=w1889, "Num Points"=w1849, "Sample I - Probe 3 (Disabled)"=w1810, "Display on/off"=TRUE, "Sample I - Source/Common"=w1809, "Sample I - Drain/Gate"=w1811, "Sampling interval"=w1847, "Standby"=w1813, "error in (no error)"=w1888, "Timings"=w1859, "Sample I - Probe 4 (Disabled)"=w1812, "Sample time"=w1848) -> ("dup VISA resource name"=w1891:refnum<visa-resource-name>, "error out"=w1890:errorcluster)  [unwired: 2 in]
        n440 = call "4155C Take SampleI v3.0.vi"("Sample I - Drain/Gate"=w1811, "Emergency Stop"=w1864, "error in (no error)"=w1890, "Idg 2"=w1850, "Vdg compliance 2"=w1846, "VISA resource name in"=w1891) -> ("error out"=w1862:errorcluster, "Idg"=w1789:dbl[], "Vdg"=w1790:dbl[], "VISA Resource Name out"=w1860:refnum<visa-resource-name>, "Is"=w1786:dbl[], "Time"=w1801:dbl[])
        n441 = case shown="2" w1803 {
          tunnel: [w1894 w1895 w1898] -> w1802
          tunnel: w1801 -> [w1893 w1895 w1897]
          frame 2 {
            n442 = Divide(x=w1893, y=3600.0) -> (x/y=w1894:dbl[])
          }
          frame 0, Default {
          }
          frame 1 {
            n443 = Divide(x=w1897, y=60.0) -> (x/y=w1898:dbl[])
          }
        }
        n444 = control-ref of="Vdg vs time (Bias Stress)"() -> (w1798:refnum<vi>)
        n445 = Add(x=w1802, y=w1800) -> (x+y=w1795:dbl[])
        n446 = Insert Into Array(array=w1796, new element=w1795) -> (w1794:dbl[])  [unwired: 1 in]
        n447 = case shown="True" w1806 {
          tunnel: w1795 -> [_ w1901]
          tunnel: [w1899 w1902] -> w1804
          tunnel: w1805 -> [w1899 w1900]
          frame False {
          }
          frame True {
            n448 = Insert Into Array(array=w1900, new element=w1901) -> (w1902:i32[])  [unwired: 1 in]
          }
        }
        n449 = Insert Into Array(array=w1791, new element=w1790) -> (w1785:dbl[])  [unwired: 1 in]
        n450 = call "4155C Split array.vi"("Number of VAR2 steps"=w1797, "X data in"=w1794, "Y1 data in"=w1785) -> ("Array of clusters"=w1799:cluster{"Y data in":dbl[], "X data in":dbl[]}[])  [unwired: 4 in, 1 out]
        n451 = local write "Vdg vs time (Bias Stress)"(w1799) -> ()
        n452 = Insert Into Array(array=dbl[][] [] ("Input Array"), new element=w1795) -> (w1874:dbl[][])  [unwired: 2 in]
        n453 = call "4155C Config Chart Colours.vi"("Numeric"=w1797, "XY Graph 2"=w1798) -> ()  [unwired: 6 in]
        n454 = Insert Into Array(array=w1793, new element=w1789) -> (w1792:dbl[])  [unwired: 1 in]
        n455 = Insert Into Array(array=w1874, new element=w1790) -> (w1873:dbl[][])  [unwired: 2 in]
        n456 = Insert Into Array(array=w1788, new element=w1786) -> (w1787:dbl[])  [unwired: 1 in]
        n457 = Insert Into Array(array=w1873, new element=w1789) -> (w1872:dbl[][])  [unwired: 2 in]
        n458 = VISA Write(VISA resource name=w1860, write buffer=":DISP ON" ("write buffer (\"\")"), error in (no error)=w1862) -> (VISA resource name out=w1845:refnum<visa-resource-name>, error out=w1861:errorcluster)  [unwired: 1 out]
        n459 = Insert Into Array(array=w1872, new element=w1786) -> (w1866:dbl[][])  [unwired: 2 in]
        n460 = call <vilib>:"compatOverwrite.vi"("overwrite (F)"=TRUE) -> ("overwrite?"=w1840:T8)
        n461 = Open/Create/Replace File(file path (use dialog)=w1870, error in=w1861, operation (0:open)=w1840) -> (refnum out=w1877:refnum<file>, error out=w1876:errorcluster)  [unwired: 3 in, 1 out]
        n462 = Transpose 2D Array(2D array=w1866) -> (transposed array=w1865:dbl[][])
        n463 = call "4155C Write array to file.vi"("Byte Stream File Refnum"=w1877, "Header"=string[] ["Time /s", "Vdg /V", "Idg /A", "Is /A"], "Data Array"=w1865, "error in (no error)"=w1876) -> ("dup refnum"=w1879:refnum<file>, "error out"=w1878:errorcluster)  [unwired: 1 in]
        n464 = Close File(refnum=w1879, error in=w1878) -> (error out=w1843:errorcluster)  [unwired: 1 out]
        n465 = VISA Write(VISA resource name=w1845, write buffer=";:PAGE:SCON:STAN OFF;:PAGE:CHAN:VSU2:DIS;" ("write buffer (\"\")"), error in (no error)=w1843) -> (VISA resource name out=w1841:refnum<visa-resource-name>, error out=w1842:errorcluster)  [unwired: 1 out]
      }
      frame "#" {
        n466 = VISA Write(VISA resource name=w1937, write buffer=":DISP ON" ("write buffer (\"\")"), error in (no error)=w1936) -> (VISA resource name out=w1935:refnum<visa-resource-name>, error out=w1934:errorcluster)  [unwired: 1 out]
      }
      frame "stressV" {
        n467 = Number To Decimal String(number=w1978) -> (decimal integer string=w2019:string)  [unwired: 1 in]
        n468 = Concatenate Strings(w2003, "-stressV-" ("Substring"), w2019, w1977, ".txt" ("Substring")) -> (w2017:string)
        n469 = Fract/Exp String To Number(string=w2016) -> (number=w1989:dbl[])  [unwired: 3 in, 1 out]
        n470 = local read "Stress V - Source/Common"() -> (w1952:u32)
        n471 = String To Path(string=w2017) -> (path=w2007:path)
        n472 = Index Array(array=w1989, index=3 ("Index")) -> (element=w1986:dbl)
        n473 = Index Array(array=w1989, index=1 ("Index")) -> (element=w1984:dbl)
        n474 = Index Array(array=w1989, index=0 ("Index")) -> (element=w1983:dbl)
        n475 = Index Array(array=w1989, index=4 ("Index")) -> (element=w1988:dbl)
        n476 = Index Array(array=w1989, index=2 ("Index")) -> (element=w1985:dbl)
        n477 = local read "Stress V - Drain"() -> (w1951:u32)
        n478 = local read "Stress V - Gate"() -> (w1950:u32)
        n479 = call "4155C Config V Stress v3.0.vi"("Display on/off"=TRUE, "Stress V - Gate"=w1950, "Stress V - Drain"=w1951, "Stress V - Source/Common"=w1952, "IG compliance"=w1985, "ID compliance"=w1986, "error in (no error)"=w2021, "VG"=w1983, "VD"=w1984, "VISA session"=w2022) -> ("error out"=w2023:errorcluster, "dup VISA resource name"=w2024:refnum<visa-resource-name>)
        n480 = call "4155C Apply Stress.vi"("error in (no error)"=w2023, "Duration"=w1988, "Emergency Stop"=w2002, "VISA resource name in"=w2024) -> ("error out"=w2000:errorcluster, "VISA Resource Name out"=w1998:refnum<visa-resource-name>)
        n481 = VISA Write(VISA resource name=w1998, write buffer=":DISP ON" ("write buffer (\"\")"), error in (no error)=w2000) -> (VISA resource name out=w1997:refnum<visa-resource-name>, error out=w1999:errorcluster)  [unwired: 1 out]
        n482 = call <vilib>:"compatOverwrite.vi"("overwrite (F)"=TRUE) -> ("overwrite?"=w1982:T8)
        n483 = Open/Create/Replace File(file path (use dialog)=w2007, error in=w1999, operation (0:open)=w1982) -> (refnum out=w2010:refnum<file>, error out=w2009:errorcluster)  [unwired: 3 in, 1 out]
        n484 = call "4155C Write array to file.vi"("Byte Stream File Refnum"=w2010, "Header"=string[] ["V stress completed successfully", ""], "error in (no error)"=w2009) -> ("dup refnum"=w2012:refnum<file>, "error out"=w2011:errorcluster)  [unwired: 2 in]
        n485 = Close File(refnum=w2012, error in=w2011) -> (error out=w2005:errorcluster)  [unwired: 1 out]
      }
      frame "stressI" {
        n486 = local read "Stress I - Source/Common"() -> (w2029:u32)
        n487 = Number To Decimal String(number=w2056) -> (decimal integer string=w2093:string)  [unwired: 1 in]
        n488 = Concatenate Strings(w2077, "-stressI-" ("Substring"), w2093, w2055, ".txt" ("Substring")) -> (w2091:string)
        n489 = Fract/Exp String To Number(string=w2090) -> (number=w2065:dbl[])  [unwired: 3 in, 1 out]
        n490 = Index Array(array=w2065, index=1 ("Index")) -> (element=w2061:dbl)
        n491 = Index Array(array=w2065, index=0 ("Index")) -> (element=w2062:dbl)
        n492 = Index Array(array=w2065, index=2 ("Index")) -> (element=w2063:dbl)
        n493 = String To Path(string=w2091) -> (path=w2081:path)
        n494 = local read "Stress I - Drain/Gate"() -> (w2030:u32)
        n495 = call "4155C Config I Stress v3.0.vi"("Stress I - Drain/Gate"=w2030, "Stress I - Source/Common"=w2029, "Display on/off"=TRUE, "error in (no error)"=w2095, "VDG compliance"=w2061, "IDG"=w2062, "VISA session"=w2096) -> ("error out"=w2097:errorcluster, "dup VISA resource name"=w2098:refnum<visa-resource-name>)  [unwired: 1 in]
        n496 = call "4155C Apply Stress.vi"("error in (no error)"=w2097, "Duration"=w2063, "Emergency Stop"=w2076, "VISA resource name in"=w2098) -> ("error out"=w2074:errorcluster, "VISA Resource Name out"=w2072:refnum<visa-resource-name>)
        n497 = VISA Write(VISA resource name=w2072, write buffer=":DISP ON" ("write buffer (\"\")"), error in (no error)=w2074) -> (VISA resource name out=w2071:refnum<visa-resource-name>, error out=w2073:errorcluster)  [unwired: 1 out]
        n498 = call <vilib>:"compatOverwrite.vi"("overwrite (F)"=TRUE) -> ("overwrite?"=w2060:T8)
        n499 = Open/Create/Replace File(file path (use dialog)=w2081, error in=w2073, operation (0:open)=w2060) -> (refnum out=w2084:refnum<file>, error out=w2083:errorcluster)  [unwired: 3 in, 1 out]
        n500 = call "4155C Write array to file.vi"("Byte Stream File Refnum"=w2084, "Header"=string[] ["I stress completed successfully", ""], "error in (no error)"=w2083) -> ("dup refnum"=w2086:refnum<file>, "error out"=w2085:errorcluster)  [unwired: 2 in]
        n501 = Close File(refnum=w2086, error in=w2085) -> (error out=w2079:errorcluster)  [unwired: 1 out]
      }
      frame "vsu2pulse" {
        n502 = Number To Decimal String(number=w2129) -> (decimal integer string=w2164:string)  [unwired: 1 in]
        n503 = Concatenate Strings(w2149, "-vsu2-" ("Substring"), w2164, w2128, ".txt" ("Substring")) -> (w2162:string)
        n504 = Fract/Exp String To Number(string=w2161) -> (number=w2137:dbl[])  [unwired: 3 in, 1 out]
        n505 = String To Path(string=w2162) -> (path=w2153:path)
        n506 = Index Array(array=w2137, index=1 ("Index")) -> (element=w2136:dbl)
        n507 = Index Array(array=w2137, index=0 ("Index")) -> (element=w2134:dbl)
        n508 = local read "VSU2 Stress - Source/Common"() -> (w2103:u32)
        n509 = call "4155C Config VSU2 Stress v3.0.vi"("VISA session"=w2167, "Display on/off"=TRUE, "VSU2"=w2134, "error in (no error)"=w2166, "VSU2 Stress - Source/Common"=w2103) -> ("dup VISA resource name"=w2169:refnum<visa-resource-name>, "error out"=w2168:errorcluster)
        n510 = call "4155C Apply Stress.vi"("error in (no error)"=w2168, "Duration"=w2136, "Emergency Stop"=w2148, "VISA resource name in"=w2169) -> ("error out"=w2146:errorcluster, "VISA Resource Name out"=w2144:refnum<visa-resource-name>)
        n511 = VISA Write(VISA resource name=w2144, write buffer=":DISP ON" ("write buffer (\"\")"), error in (no error)=w2146) -> (VISA resource name out=w2143:refnum<visa-resource-name>, error out=w2145:errorcluster)  [unwired: 1 out]
        n512 = call <vilib>:"compatOverwrite.vi"("overwrite (F)"=TRUE) -> ("overwrite?"=w2133:T8)
        n513 = Open/Create/Replace File(file path (use dialog)=w2153, error in=w2145, operation (0:open)=w2133) -> (refnum out=w2156:refnum<file>, error out=w2155:errorcluster)  [unwired: 3 in, 1 out]
        n514 = call "4155C Write array to file.vi"("Byte Stream File Refnum"=w2156, "Header"=string[] ["VSU2 pulse completed successfully", ""], "error in (no error)"=w2155) -> ("dup refnum"=w2158:refnum<file>, "error out"=w2157:errorcluster)  [unwired: 2 in]
        n515 = Close File(refnum=w2158, error in=w2157) -> (error out=w2151:errorcluster)  [unwired: 1 out]
      }
      frame "sample-fpp" {
        w2180 = 1
        w2245 = string[] ["Time /s", "Id VgVd /A", "Ig VgVd /A", "Vp1 VgVd /V", "Vp2 VgVd /V"] ("Header")
        w2249 = "%d" ("format string")
        # "Y1 = Y2 = ID\nY3 = IG"
        # "Y1 = Vp2\nY2 = Y3 = Vp1"
        # "Add a time offset (elapsed time) to the time axis."
        n516 = local read "Plot sample extrema vs time"() -> (w2189:bool)
        n517 = Number To Decimal String(number=w2237) -> (decimal integer string=w2291:string)  [unwired: 1 in]
        n518 = Fract/Exp String To Number(string=w2288) -> (number=w2276:dbl[])  [unwired: 3 in, 1 out]
        n519 = local read "Plot sample extrema vs time"() -> (w2192:bool)
        n520 = Concatenate Strings(w2282, "-samplefpp-" ("Substring"), w2291, w2236, ".txt" ("Substring")) -> (w2289:string)
        n521 = local read "FPP - Source"() -> (w2215:u32)
        n522 = local read "FPP - Drain"() -> (w2216:u32)
        n523 = local read "FPP - Gate"() -> (w2217:u32)
        n524 = local read "FPP - Probe 1"() -> (w2218:u32)
        n525 = control-ref of="I vs time (Bias Stress)"() -> (w2209:refnum<vi>)
        n526 = String To Path(string=w2289) -> (path=w2257:path)
        n527 = Index Array(array=w2276, index=0 ("Index")) -> (element=w2244:dbl)
        n528 = Index Array(array=w2276, index=1 ("Index")) -> (element=w2243:dbl)
        n529 = local read "Time Units"() -> (w2205:u16)
        n530 = Index Array(array=w2276, index=2 ("Index")) -> (element=w2284:dbl)
        n531 = Index Array(array=w2276, index=3 ("Index")) -> (element=w2274:dbl)
        n532 = Number To Decimal String(number=w2244) -> (decimal integer string=w2265:string)  [unwired: 1 in]
        n533 = local read "FPP - Probe 2"() -> (w2219:u32)
        n534 = call "4155C Config Sampling Measurements FPP v3.0.vi"("VISA session"=w2294, "Gate Compliance"=w2283, "FPP - Source"=w2215, "FPP - Drain"=w2216, "Drain Compliance"=w2292, "error in (no error)"=w2293, "Num Points"=w2284, "Timings"=w2281, "FPP - Gate"=w2217, "FPP - Probe 1"=w2218, "Vg"=w2244, "Vd"=w2243, "Display on/off"=TRUE, "Sample time"=w2274, "FPP - Probe 2"=w2219, "Standby"=w2220) -> ("dup VISA resource name"=w2259:refnum<visa-resource-name>, "error out"=w2258:errorcluster)  [unwired: 2 in]
        n535 = call "4155C Take Sample FPP.vi"("VISA resource name in"=w2259, "error in (no error)"=w2258, "Emergency Stop"=w2260) -> ("Time"=w2208:dbl[], "Vp1"=w2175:dbl[], "VISA Resource Name out"=w2241:refnum<visa-resource-name>, "Ig"=w2186:dbl[], "Id"=w2185:dbl[], "Vp2"=w2174:dbl[], "error out"=w2188:errorcluster)  [unwired: 10 in]
        n536 = Insert Into Array(array=w2213, new element=w2185) -> (w2172:dbl[])  [unwired: 1 in]
        n537 = Insert Into Array(array=w2214, new element=w2186) -> (w2211:dbl[])  [unwired: 1 in]
        n538 = Number To Decimal String(number=w2243) -> (decimal integer string=w2263:string)  [unwired: 1 in]
        n539 = call "4155C Config Chart Colours.vi"("Numeric"=w2180, "XY Graph 2"=w2209) -> ()  [unwired: 6 in]
        n540 = case shown="2" w2205 {
          tunnel: [w2334 w2335 w2338] -> w2207
          tunnel: w2208 -> [w2333 w2335 w2337]
          frame 2 {
            n541 = Divide(x=w2333, y=3600.0) -> (x/y=w2334:dbl[])
          }
          frame 0, Default {
          }
          frame 1 {
            n542 = Divide(x=w2337, y=60.0) -> (x/y=w2338:dbl[])
          }
        }
        n543 = Concatenate Strings("(Vg = " ("Substring"), w2265, "V, Vd = " ("Substring"), w2263, "V)" ("Substring")) -> (w2261:string)
        n544 = Add(x=w2207, y=w2206) -> (x+y=w2179:dbl[])
        n545 = case shown="True" w2189 {
          tunnel: w2179 -> [_ w2297]
          tunnel: [w2295 w2298] -> w2190
          tunnel: w2191 -> [w2295 w2296]
          frame False {
          }
          frame True {
            n546 = Insert Into Array(array=w2296, new element=w2297) -> (w2298:i32[])  [unwired: 1 in]
          }
        }
        n547 = case shown="True" w2192 {
          tunnel: w2185 -> [_ w2325]
          tunnel: w2186 -> [_ w2326]
          tunnel: [w2305 w2317] -> w2187
          tunnel: w2188 -> [w2305 w2320]
          tunnel: w2204 -> [w2304 w2310]
          tunnel: w2203 -> [w2303 w2309]
          tunnel: w2202 -> [w2302 w2328]
          tunnel: w2201 -> [w2301 w2327]
          tunnel: w2200 -> [w2300 w2329]
          tunnel: [w2304 w2310] -> w2198
          tunnel: [w2303 w2309] -> w2197
          tunnel: [w2302 w2306] -> w2196
          tunnel: [w2301 w2307] -> w2195
          tunnel: [w2300 w2319] -> w2194
          tunnel: [w2299 w2315] -> w2193
          tunnel: w2190 -> [_ w2313]
          tunnel: w2199 -> [w2299 w2308]
          frame False {
          }
          frame True {
            w2316 = 1
            # "Y1 = Y2 = ID\nY3 = IG"
            # "Number of VAR2 steps is 1."
            # "abs(Ig)"
            # "abs(Id)"
            # "Adjusts graph colors."
            n548 = Absolute Value(x=w2326) -> (abs(x)=w2311:dbl[])
            n549 = Absolute Value(x=w2325) -> (abs(x)=w2312:dbl[])
            n550 = Array Max & Min(array=w2312) -> (max value=w2324:dbl, min value=w2322:dbl)  [unwired: 2 out]
            n551 = Array Max & Min(array=w2311) -> (max value=w2323:dbl, min value=w2321:dbl)  [unwired: 2 out]
            n552 = Insert Into Array(array=w2329, new element=w2311) -> (w2319:dbl[])  [unwired: 1 in]
            n553 = local write "Id max"(w2324) -> ()
            n554 = local write "Id min"(w2322) -> ()
            n555 = local write "Ig max"(w2323) -> ()
            n556 = local write "Ig min"(w2321) -> ()
            n557 = Insert Into Array(array=w2308, new element=w2311) -> (w2315:dbl[])  [unwired: 1 in]
            n558 = Insert Into Array(array=w2328, new element=w2312) -> (w2306:dbl[])  [unwired: 1 in]
            n559 = Insert Into Array(array=w2327, new element=w2312) -> (w2307:dbl[])  [unwired: 1 in]
            n560 = control-ref of="Imax vs time"() -> (w2330:refnum<vi>)
            n561 = call "4155C Config Chart Colours.vi"("Numeric"=w2316, "XY Graph 2"=w2330) -> ()  [unwired: 6 in]
            n562 = call "4155C Split array.vi"("Number of VAR2 steps"=w2316, "Y2 data in"=w2306, "X data in"=w2313, "Y1 data in"=w2306, "Y3 data in"=w2319, "error in (no error)"=w2320) -> ("Array of clusters"=w2331:cluster{"Y data in":dbl[], "X data in":dbl[]}[], "error out"=w2318:errorcluster)  [unwired: 1 in]
            n563 = call "4155C Split array.vi"("Number of VAR2 steps"=w2316, "Y2 data in"=w2307, "X data in"=w2313, "Y1 data in"=w2307, "Y3 data in"=w2315, "error in (no error)"=w2318) -> ("Array of clusters"=w2314:cluster{"Y data in":dbl[], "X data in":dbl[]}[], "error out"=w2317:errorcluster)  [unwired: 1 in]
            n564 = local write "Imax vs time"(w2331) -> ()
            n565 = local write "Imin vs time"(w2314) -> ()
          }
        }
        n566 = Insert Into Array(array=w2212, new element=w2179) -> (w2181:dbl[])  [unwired: 1 in]
        n567 = call "4155C Split array.vi"("Number of VAR2 steps"=w2180, "Y2 data in"=w2172, "X data in"=w2181, "Y1 data in"=w2172, "Y3 data in"=w2211) -> ("Array of clusters"=w2210:cluster{"Y data in":dbl[], "X data in":dbl[]}[])  [unwired: 2 in, 1 out]
        n568 = local write "I vs time (Bias Stress)"(w2210) -> ()
        n569 = Insert Into Array(array=w2178, new element=w2175) -> (w2173:dbl[])  [unwired: 1 in]
        n570 = Insert Into Array(array=w2177, new element=w2174) -> (w2176:dbl[])  [unwired: 1 in]
        n571 = Insert Into Array(array=dbl[][] [] ("Input Array"), new element=w2179) -> (w2272:dbl[][])  [unwired: 2 in]
        n572 = control-ref of="Vp vs time (FPP Bias Stress)"() -> (w2182:refnum<vi>)
        n573 = Insert Into Array(array=w2272, new element=w2185) -> (w2271:dbl[][])  [unwired: 2 in]
        n574 = call <vilib>:"compatOverwrite.vi"("overwrite (F)"=TRUE) -> ("overwrite?"=w2239:T8)
        n575 = Open/Create/Replace File(file path (use dialog)=w2257, error in=w2187, operation (0:open)=w2239) -> (refnum out=w2254:refnum<file>, error out=w2255:errorcluster)  [unwired: 3 in, 1 out]
        n576 = Array To Spreadsheet String(array=w2245, 3:w2249) -> (spreadsheet string=w2251:string)  [unwired: 1 in]
        n577 = call "4155C Split array.vi"("Number of VAR2 steps"=w2180, "Y2 data in"=w2173, "X data in"=w2181, "Y1 data in"=w2176, "Y3 data in"=w2173) -> ("Array of clusters"=w2183:cluster{"Y data in":dbl[], "X data in":dbl[]}[])  [unwired: 2 in, 1 out]
        n578 = Insert Into Array(array=w2271, new element=w2186) -> (w2270:dbl[][])  [unwired: 2 in]
        n579 = Search and Replace String(replace all?=TRUE ("replace all? (F)"), input string=w2251, search string="VgVd", replace string=w2261) -> (result string=w2247:string)  [unwired: 4 in, 3 out]
        n580 = local write "Vp vs time (FPP Bias Stress)"(w2183) -> ()
        n581 = Insert Into Array(array=w2270, new element=w2175) -> (w2268:dbl[][])  [unwired: 2 in]
        n582 = call "4155C Config Chart Colours.vi"("Numeric"=w2180, "XY Graph 2"=w2182) -> ()  [unwired: 6 in]
        n583 = Spreadsheet String To Array(format string=w2249, spreadsheet string=w2247, array type (2D Dbl)=w2245) -> (array=w2246:string[])  [unwired: 1 in]
        n584 = Insert Into Array(array=w2268, new element=w2174) -> (w2242:dbl[][])  [unwired: 2 in]
        n585 = Transpose 2D Array(2D array=w2242) -> (transposed array=w2267:dbl[][])
        n586 = call "4155C Write array to file.vi"("Byte Stream File Refnum"=w2254, "Header"=w2246, "Data Array"=w2267, "error in (no error)"=w2255) -> ("dup refnum"=w2252:refnum<file>, "error out"=w2253:errorcluster)  [unwired: 1 in]
        n587 = Close File(refnum=w2252, error in=w2253) -> (error out=w2240:errorcluster)  [unwired: 1 out]
      }
      frame "resample-fpp" {
        w2349 = 1
        w2411 = string[] ["Time /s", "Id VgVd /A", "Ig VgVd /A", "Vp1 VgVd /V", "Vp2 VgVd /V"] ("Header")
        w2415 = "%d" ("format string")
        # "Y1 = Y2 = ID\nY3 = IG"
        # "Y1 = Vp2\nY2 = Y3 = Vp1"
        # "Add a time offset (elapsed time) to the time axis."
        n588 = Number To Decimal String(number=w2399) -> (decimal integer string=w2449:string)  [unwired: 1 in]
        n589 = local read "Plot sample extrema vs time"() -> (w2358:bool)
        n590 = Fract/Exp String To Number(string=w2446) -> (number=w2404:dbl[])  [unwired: 3 in, 1 out]
        n591 = Concatenate Strings(w2442, "-resamplefpp-" ("Substring"), w2449, w2400, ".txt" ("Substring")) -> (w2447:string)
        n592 = local read "Plot sample extrema vs time"() -> (w2361:bool)
        n593 = String To Path(string=w2447) -> (path=w2423:path)
        n594 = local read "Time Units"() -> (w2374:u16)
        n595 = Index Array(array=w2404, index=0 ("Index")) -> (element=w2410:dbl)
        n596 = Index Array(array=w2404, index=1 ("Index")) -> (element=w2409:dbl)
        n597 = Number To Decimal String(number=w2410) -> (decimal integer string=w2429:string)  [unwired: 1 in]
        n598 = call "4155C Take Sample FPP.vi"("VISA resource name in"=w2406, "error in (no error)"=w2405, "Emergency Stop"=w2424) -> ("Time"=w2375:dbl[], "Vp1"=w2344:dbl[], "VISA Resource Name out"=w2408:refnum<visa-resource-name>, "Ig"=w2355:dbl[], "Id"=w2354:dbl[], "Vp2"=w2343:dbl[], "error out"=w2357:errorcluster)  [unwired: 10 in]
        n599 = Insert Into Array(array=w2382, new element=w2354) -> (w2341:dbl[])  [unwired: 1 in]
        n600 = case shown="1" w2374 {
          tunnel: [w2490 w2491 w2494] -> w2377
          tunnel: w2375 -> [w2489 w2491 w2493]
          frame 2 {
            n601 = Divide(x=w2489, y=3600.0) -> (x/y=w2490:dbl[])
          }
          frame 0, Default {
          }
          frame 1 {
            n602 = Divide(x=w2493, y=60.0) -> (x/y=w2494:dbl[])
          }
        }
        n603 = Insert Into Array(array=w2383, new element=w2355) -> (w2380:dbl[])  [unwired: 1 in]
        n604 = Number To Decimal String(number=w2409) -> (decimal integer string=w2427:string)  [unwired: 1 in]
        n605 = Add(x=w2377, y=w2376) -> (x+y=w2348:dbl[])
        n606 = case shown="True" w2358 {
          tunnel: w2348 -> [_ w2453]
          tunnel: [w2451 w2454] -> w2359
          tunnel: w2360 -> [w2451 w2452]
          frame False {
          }
          frame True {
            n607 = Insert Into Array(array=w2452, new element=w2453) -> (w2454:i32[])  [unwired: 1 in]
          }
        }
        n608 = case shown="True" w2361 {
          tunnel: w2354 -> [_ w2480]
          tunnel: w2355 -> [_ w2481]
          tunnel: [w2461 w2472] -> w2356
          tunnel: w2357 -> [w2461 w2475]
          tunnel: w2373 -> [w2460 w2465]
          tunnel: w2371 -> [w2459 w2464]
          tunnel: w2369 -> [w2458 w2483]
          tunnel: w2368 -> [w2457 w2482]
          tunnel: w2367 -> [w2456 w2485]
          tunnel: w2366 -> [w2455 w2484]
          tunnel: [w2460 w2465] -> w2372
          tunnel: [w2459 w2464] -> w2370
          tunnel: [w2458 w2463] -> w2365
          tunnel: [w2457 w2462] -> w2364
          tunnel: [w2456 w2474] -> w2363
          tunnel: [w2455 w2470] -> w2362
          tunnel: w2359 -> [_ w2468]
          frame False {
          }
          frame True {
            w2471 = 1
            # "Y1 = Y2 = ID\nY3 = IG"
            # "Number of VAR2 steps is 1."
            # "abs(Ig)"
            # "abs(Id)"
            # "Adjusts graph colors."
            n609 = Absolute Value(x=w2481) -> (abs(x)=w2466:dbl[])
            n610 = Absolute Value(x=w2480) -> (abs(x)=w2467:dbl[])
            n611 = Array Max & Min(array=w2467) -> (max value=w2479:dbl, min value=w2477:dbl)  [unwired: 2 out]
            n612 = Array Max & Min(array=w2466) -> (max value=w2478:dbl, min value=w2476:dbl)  [unwired: 2 out]
            n613 = local write "Id max"(w2479) -> ()
            n614 = local write "Id min"(w2477) -> ()
            n615 = local write "Ig max"(w2478) -> ()
            n616 = local write "Ig min"(w2476) -> ()
            n617 = Insert Into Array(array=w2485, new element=w2466) -> (w2474:dbl[])  [unwired: 1 in]
            n618 = Insert Into Array(array=w2484, new element=w2466) -> (w2470:dbl[])  [unwired: 1 in]
            n619 = Insert Into Array(array=w2483, new element=w2467) -> (w2463:dbl[])  [unwired: 1 in]
            n620 = Insert Into Array(array=w2482, new element=w2467) -> (w2462:dbl[])  [unwired: 1 in]
            n621 = control-ref of="Imax vs time"() -> (w2486:refnum<vi>)
            n622 = call "4155C Config Chart Colours.vi"("Numeric"=w2471, "XY Graph 2"=w2486) -> ()  [unwired: 6 in]
            n623 = call "4155C Split array.vi"("Number of VAR2 steps"=w2471, "Y2 data in"=w2463, "X data in"=w2468, "Y1 data in"=w2463, "Y3 data in"=w2474, "error in (no error)"=w2475) -> ("Array of clusters"=w2487:cluster{"Y data in":dbl[], "X data in":dbl[]}[], "error out"=w2473:errorcluster)  [unwired: 1 in]
            n624 = call "4155C Split array.vi"("Number of VAR2 steps"=w2471, "Y2 data in"=w2462, "X data in"=w2468, "Y1 data in"=w2462, "Y3 data in"=w2470, "error in (no error)"=w2473) -> ("Array of clusters"=w2469:cluster{"Y data in":dbl[], "X data in":dbl[]}[], "error out"=w2472:errorcluster)  [unwired: 1 in]
            n625 = local write "Imax vs time"(w2487) -> ()
            n626 = local write "Imin vs time"(w2469) -> ()
          }
        }
        n627 = Insert Into Array(array=w2381, new element=w2348) -> (w2350:dbl[])  [unwired: 1 in]
        n628 = Concatenate Strings("(Vg = " ("Substring"), w2429, "V, Vd = " ("Substring"), w2427, "V)" ("Substring")) -> (w2425:string)
        n629 = control-ref of="I vs time (Bias Stress)"() -> (w2378:refnum<vi>)
        n630 = call "4155C Split array.vi"("Number of VAR2 steps"=w2349, "Y2 data in"=w2341, "X data in"=w2350, "Y1 data in"=w2341, "Y3 data in"=w2380) -> ("Array of clusters"=w2379:cluster{"Y data in":dbl[], "X data in":dbl[]}[])  [unwired: 2 in, 1 out]
        n631 = local write "I vs time (Bias Stress)"(w2379) -> ()
        n632 = call "4155C Config Chart Colours.vi"("Numeric"=w2349, "XY Graph 2"=w2378) -> ()  [unwired: 6 in]
        n633 = Insert Into Array(array=dbl[][] [] ("Input Array"), new element=w2348) -> (w2436:dbl[][])  [unwired: 2 in]
        n634 = Insert Into Array(array=w2347, new element=w2344) -> (w2342:dbl[])  [unwired: 1 in]
        n635 = Insert Into Array(array=w2436, new element=w2354) -> (w2435:dbl[][])  [unwired: 2 in]
        n636 = call <vilib>:"compatOverwrite.vi"("overwrite (F)"=TRUE) -> ("overwrite?"=w2402:T8)
        n637 = Open/Create/Replace File(file path (use dialog)=w2423, error in=w2356, operation (0:open)=w2402) -> (refnum out=w2420:refnum<file>, error out=w2421:errorcluster)  [unwired: 3 in, 1 out]
        n638 = Array To Spreadsheet String(array=w2411, 3:w2415) -> (spreadsheet string=w2417:string)  [unwired: 1 in]
        n639 = Insert Into Array(array=w2435, new element=w2355) -> (w2434:dbl[][])  [unwired: 2 in]
        n640 = Insert Into Array(array=w2346, new element=w2343) -> (w2345:dbl[])  [unwired: 1 in]
        n641 = Search and Replace String(replace all?=TRUE ("replace all? (F)"), input string=w2417, search string="VgVd", replace string=w2425) -> (result string=w2413:string)  [unwired: 4 in, 3 out]
        n642 = Insert Into Array(array=w2434, new element=w2344) -> (w2432:dbl[][])  [unwired: 2 in]
        n643 = Spreadsheet String To Array(format string=w2415, spreadsheet string=w2413, array type (2D Dbl)=w2411) -> (array=w2412:string[])  [unwired: 1 in]
        n644 = Insert Into Array(array=w2432, new element=w2343) -> (w2403:dbl[][])  [unwired: 2 in]
        n645 = control-ref of="Vp vs time (FPP Bias Stress)"() -> (w2351:refnum<vi>)
        n646 = Transpose 2D Array(2D array=w2403) -> (transposed array=w2431:dbl[][])
        n647 = call "4155C Write array to file.vi"("Byte Stream File Refnum"=w2420, "Header"=w2412, "Data Array"=w2431, "error in (no error)"=w2421) -> ("dup refnum"=w2418:refnum<file>, "error out"=w2419:errorcluster)  [unwired: 1 in]
        n648 = Close File(refnum=w2418, error in=w2419) -> (error out=w2407:errorcluster)  [unwired: 1 out]
        n649 = call "4155C Split array.vi"("Number of VAR2 steps"=w2349, "Y2 data in"=w2342, "X data in"=w2350, "Y1 data in"=w2345, "Y3 data in"=w2342) -> ("Array of clusters"=w2352:cluster{"Y data in":dbl[], "X data in":dbl[]}[])  [unwired: 2 in, 1 out]
        n650 = local write "Vp vs time (FPP Bias Stress)"(w2352) -> ()
        n651 = call "4155C Config Chart Colours.vi"("Numeric"=w2349, "XY Graph 2"=w2351) -> ()  [unwired: 6 in]
      }
      frame "serial" {
        n652 = local read "Termination char\n(0xA = '\\n' = LF)\n(0xD = '\\r' = CR)"() -> (w2530:u8)
        n653 = local read "Enable Termination\nChar (T)"() -> (w2531:bool)
        n654 = Index Array(array=w2538, index=0 ("Index")) -> (element=w2537:string)
        n655 = local read "parity"() -> (w2521:u16)
        n656 = local read "Delay before read (ms)"() -> (w2532:u32)
        n657 = local read "byte count"() -> (w2529:u32)
        n658 = local read "VISA resource name"() -> (w2525:refnum<visa-resource-name>)
        n659 = local read "baud rate"() -> (w2524:u32)
        n660 = local read "Serial End Mode for Reads"() -> (w2523:u16)
        n661 = local read "Timeout (ms)"() -> (w2528:u32)
        n662 = local read "data bits"() -> (w2522:u16)
        n663 = local read "stop bits"() -> (w2527:u16)
        n664 = local read "flow control"() -> (w2526:u16)
        n665 = call "Serial write and read v0.5.vi"("Delay before read (ms)"=w2532, "Termination char\n(0xA = '\\n' = LF)\n(0xD = '\\r' = CR)"=w2530, "Enable Termination\nChar (T)"=w2531, "parity"=w2521, "stop bits"=w2527, "string to write"=w2537, "flow control"=w2526, "byte count"=w2529, "Serial Settings:Serial End Mode for Reads"=w2523, "Timeout (ms)"=w2528, "error in (no error)"=w2543, "VISA resource name"=w2525, "baud rate"=w2524, "data bits"=w2522) -> ("Serial port output"=w2533:string, "error out"=w2542:errorcluster)
        n666 = Build Array (concatenate)(w2533, w2534) -> (w2535:string[])
      }
      frame "pump" {
        # "Time array for valve position"
        # "Time array for absolute plunger position"
        # "Valve position"
        # "Absolute plunger position"
        # "Remove \"_\""
        # "Check if pump is idle. Else halt."
        n667 = Index Array(array=w2615, index=0 ("Index")) -> (element=w2596:string)
        n668 = local read "Hard stop pump"() -> (w2555:bool)
        n669 = local read "Halt pump"() -> (w2556:bool)
        n670 = local read "Serial End Mode for Reads"() -> (w2603:u16)
        n671 = local read "flow control"() -> (w2606:u16)
        n672 = local read "stop bits"() -> (w2607:u16)
        n673 = local read "parity"() -> (w2601:u16)
        n674 = local read "Delay before read (ms)"() -> (w2612:u32)
        n675 = local read "byte count"() -> (w2609:u32)
        n676 = local read "VISA resource name"() -> (w2605:refnum<visa-resource-name>)
        n677 = local read "baud rate"() -> (w2604:u32)
        n678 = local read "Timeout (ms)"() -> (w2608:u32)
        n679 = local read "Termination char\n(0xA = '\\n' = LF)\n(0xD = '\\r' = CR)"() -> (w2610:u8)
        n680 = local read "Enable Termination\nChar (T)"() -> (w2611:bool)
        n681 = case shown="\"Internal failure\"" w2595 {
          tunnel: w2596 -> [w2651 _ w2653 w2654 w2655 w2656 _ _ w2659 w2660 _]
          tunnel: [w2651 "/1H" w2653 w2654 w2655 w2656 "/1H" "/1H" w2659 w2660 "/1H"] -> w2557
          frame "No error", Default {
          }
          frame "Initialization" {
          }
          frame "Invalid command" {
          }
          frame "Invalid operand" {
          }
          frame "Device not initialized" {
          }
          frame "Internal failure" {
          }
          frame "Plunger overload" {
          }
          frame "Valve overload" {
          }
          frame "Plunger move not allowed" {
          }
          frame "A/D converter failure" {
          }
          frame "Command overflow" {
          }
        }
        n682 = local read "data bits"() -> (w2602:u16)
        n683 = String Subset(string=w2591, offset (0)=1) -> (substring=w2589:string)  [unwired: 1 in]
        n684 = call "SPM Pump v0.7.vi"("Termination char\n(0xA = '\\n' = LF)\n(0xD = '\\r' = CR)"=w2610, "Enable Termination\nChar (T)"=w2611, "Timeout (ms)"=w2608, "Serial Settings:Serial End Mode for Reads"=w2603, "byte count"=w2609, "Delay before read (ms)"=w2612, "Time <input>"=w2594, "error in (no error)"=w2620, "Serial port input"=w2557, "VISA resource name"=w2605, "parity"=w2601, "baud rate"=w2604, "stop bits"=w2607, "data bits"=w2602, "flow control"=w2606, "Time units <input>"=w2589, "Hard stop pump"=w2555, "Halt pump"=w2556) -> ("Input command"=w2588:string, "Serial port data"=w2578:string[], "Pump status"=w2584:string, "Valve position"=w2586:i32, "Absolute plunger position"=w2597:i32, "Serial port"=w2593:string, "error out"=w2619:errorcluster)  [unwired: 2 in, 1 out]
        n685 = case shown="\"?6\"" w2588 {
          tunnel: [w2632 w2640 w2646] -> w2600
          tunnel: w2599 -> [w2632 w2639 w2646]
          tunnel: w2597 -> [_ w2638 _]
          tunnel: w2585 -> [w2631 w2637 w2647]
          tunnel: [w2631 w2637 w2649] -> w2587
          tunnel: w2586 -> [_ _ w2648]
          tunnel: w2583 -> [_ w2636 w2644]
          tunnel: w2582 -> [w2630 w2635 w2645]
          tunnel: [w2630 w2634 w2645] -> w2581
          tunnel: [w2629 w2633 w2643] -> w2580
          tunnel: w2579 -> [w2629 w2633 w2642]
          frame "Q", Default {
          }
          frame "?" {
            n686 = Build Array (concatenate)(w2639, w2638) -> (w2640:i32[])
            n687 = Build Array (concatenate)(w2635, w2636) -> (w2634:i32[])
            n688 = call "4155C Split array.vi"("X data in"=w2634, "Y1 data in"=w2640) -> ("Array of clusters"=w2641:cluster{"Y data in":dbl[], "X data in":dbl[]}[])  [unwired: 5 in, 1 out]
            n689 = local write "Absolute plunger position vs time"(w2641) -> ()
          }
          frame "?6" {
            n690 = Build Array (concatenate)(w2647, w2648) -> (w2649:i32[])
            n691 = Build Array (concatenate)(w2642, w2644) -> (w2643:i32[])
            n692 = call "4155C Split array.vi"("X data in"=w2643, "Y1 data in"=w2649) -> ("Array of clusters"=w2650:cluster{"Y data in":dbl[], "X data in":dbl[]}[])  [unwired: 5 in, 1 out]
            n693 = local write "Valve position vs time"(w2650) -> ()
          }
        }
        n694 = Build Array (concatenate)(w2576, w2578) -> (w2577:string[][])
        n695 = Build Array (concatenate)(w2592, w2593) -> (w2613:string[])
      }
      frame "filename" {
        n696 = Index Array(array=w2672, index=0 ("Index")) -> (element=w2671:string)
      }
    }
    "Probe 4 Indicator" <- w78
    "Timings Indicator" <- w77
    n697 = local read "Time Units"() -> (w111:u16)
    n698 = case shown="0" w111 {
      tunnel: ["Time (Seconds)" ("element") "Time (Minutes)" ("element") "Time (Hours)" ("element")] -> w79
      frame 0 {
      }
      frame 1, Default {
      }
      frame 2 {
      }
    }
    n699 = Build Array(w185, w118, w128, w127, w126, w125, w124, w123, w122, w121, w120, w119, w117) -> (w223:dbl[][])
    n700 = Transpose 2D Array(2D array=w223) -> (transposed array=w222:dbl[][])
    n701 = Concatenate Strings(w86, w85, "I-vs-time.txt" ("Suffix (Imax,Imin,Ion,Ioff)")) -> (w233:string)
    n702 = Build Array(w79, "Is max (A)" ("VAR2 Name"), "Is min (A)" ("VAR2 Name"), "Id max (A)" ("VAR2 Name"), "Id min (A)" ("VAR2 Name"), "Ig max (A)" ("VAR2 Name"), "Ig min (A)" ("VAR2 Name"), "Is on (A)" ("VAR2 Name"), "Is off (A)" ("VAR2 Name"), "Id on (A)" ("VAR2 Name"), "Id off (A)" ("VAR2 Name"), "Ig on (A)" ("VAR2 Name"), "Ig off (A)" ("VAR2 Name")) -> (w228:string[])
    n703 = Array To Spreadsheet String(array=w222, 3:"%e" ("format string")) -> (spreadsheet string=w226:string)  [unwired: 1 in]
    n704 = Array To Spreadsheet String(array=w228, 3:"" ("format string")) -> (spreadsheet string=w227:string)  [unwired: 1 in]
    n705 = String To Path(string=w233) -> (path=w232:path)
    n706 = Build Array(w227, w226) -> (w225:string[])
    n707 = Write to Text File(file (use dialog)=w232, text=w225, error in=w182) -> (refnum out=w234:refnum<file>, error out=w224:errorcluster)  [unwired: 1 in, 1 out]
    n708 = Close File(refnum=w234, error in=w224) -> (error out=w166:errorcluster)  [unwired: 1 out]
    n709 = Build Array(w163, w186) -> (w191:i32[][])
    n710 = Build Array(w79, "Absolute plunger position" ("VAR2 Name")) -> (w194:string[])
    n711 = Transpose 2D Array(2D array=w191) -> (transposed array=w184:i32[][])
    n712 = Array To Spreadsheet String(array=w194, 3:"" ("format string")) -> (spreadsheet string=w193:string)  [unwired: 1 in]
    n713 = Array To Spreadsheet String(array=w184, 3:"%e" ("format string")) -> (spreadsheet string=w190:string)  [unwired: 1 in]
    n714 = Build Array(w193, w190) -> (w196:string[])
    n715 = Concatenate Strings(w86, w85, "plunger.txt" ("Suffix (plunger)")) -> (w188:string)
    n716 = String To Path(string=w188) -> (path=w187:path)
    n717 = Write to Text File(file (use dialog)=w187, text=w196, error in=w166) -> (refnum out=w189:refnum<file>, error out=w198:errorcluster)  [unwired: 1 in, 1 out]
    n718 = Close File(refnum=w189, error in=w198) -> (error out=w165:errorcluster)  [unwired: 1 out]
    n719 = Concatenate Strings(w86, w85, "serial-port.txt" ("Suffix (serial port log)")) -> (w204:string)
    n720 = String To Path(string=w204) -> (path=w203:path)
    n721 = Build Array(w79, "Serial port input" ("VAR2 Name"), "Pump status" ("VAR2 Name"), "Serial port output: ") -> (w153:string[])
    n722 = Array To Spreadsheet String(array=w159, 3:"" ("format string")) -> (spreadsheet string=w150:string)  [unwired: 1 in]
    n723 = Array To Spreadsheet String(array=w153, 3:"" ("format string")) -> (spreadsheet string=w151:string)  [unwired: 1 in]
    n724 = Array To Spreadsheet String(array=w158, 3:"" ("format string")) -> (spreadsheet string=w209:string)  [unwired: 1 in]
    n725 = Build Array(w151, w150) -> (w152:string[])
    n726 = Write to Text File(file (use dialog)=w203, text=w152, error in=w165) -> (refnum out=w205:refnum<file>, error out=w206:errorcluster)  [unwired: 1 in, 1 out]
    n727 = local write "Serial port data"(w209) -> ()
    n728 = Close File(refnum=w205, error in=w206) -> (error out=w164:errorcluster)  [unwired: 1 out]
    n729 = Build Array(w162, w168) -> (w174:i32[][])
    n730 = Build Array(w79, "Valve port" ("VAR2 Name")) -> (w177:string[])
    n731 = Transpose 2D Array(2D array=w174) -> (transposed array=w169:i32[][])
    n732 = Array To Spreadsheet String(array=w177, 3:"" ("format string")) -> (spreadsheet string=w176:string)  [unwired: 1 in]
    n733 = Array To Spreadsheet String(array=w169, 3:"%e" ("format string")) -> (spreadsheet string=w173:string)  [unwired: 1 in]
    n734 = Build Array(w176, w173) -> (w179:string[])
    n735 = Concatenate Strings(w86, w85, "valve-port.txt" ("Suffix (valve)")) -> (w171:string)
    n736 = String To Path(string=w171) -> (path=w170:path)
    n737 = Write to Text File(file (use dialog)=w170, text=w179, error in=w164) -> (refnum out=w172:refnum<file>, error out=w181:errorcluster)  [unwired: 1 in, 1 out]
    n738 = Close File(refnum=w172, error in=w181) -> (error out=w87:errorcluster)  [unwired: 1 out]
    n739 = Build Array(w84, w83, w82, w81) -> (w96:dbl[][])
    n740 = Build Array(w79, "Is (A)" ("VAR2 Name"), "Id (A)" ("VAR2 Name"), "Ig (A)" ("VAR2 Name")) -> (w92:string[])
    n741 = Transpose 2D Array(2D array=w96) -> (transposed array=w95:dbl[][])
    n742 = Concatenate Strings(w86, w85, "sample.txt" ("Suffix (Imax,Imin,Ion,Ioff)")) -> (w102:string)
    n743 = Array To Spreadsheet String(array=w92, 3:"" ("format string")) -> (spreadsheet string=w91:string)  [unwired: 1 in]
    n744 = Array To Spreadsheet String(array=w95, 3:"%e" ("format string")) -> (spreadsheet string=w99:string)  [unwired: 1 in]
    n745 = local write "Hard stop pump"(w71) -> ()
    n746 = String To Path(string=w102) -> (path=w101:path)
    n747 = local write "Halt pump"(w71) -> ()
    n748 = Build Array(w91, w99) -> (w98:string[])
    n749 = Write to Text File(file (use dialog)=w101, text=w98, error in=w87) -> (refnum out=w103:refnum<file>, error out=w97:errorcluster)  [unwired: 1 in, 1 out]
    n750 = Close File(refnum=w103, error in=w97) -> (error out=w76:errorcluster)  [unwired: 1 out]
    "error out" <- w76
  }
  "Is max" <- w15
  "Id max" <- w15
  "Ig max" <- w15
  "Imax vs time" <- w2
  "I vs Vg" <- w2
  "Imin vs time" <- w2
  "I vs Vd" <- w2
  "Serial port data" <- "" ("Serial port data")
  "Absolute plunger position vs time" <- w2
  "Valve position vs time" <- cluster{"Y data in":dbl[], "X data in":dbl[]}[] [] ("Valve position vs time")
  "Is min" <- w14
  "Id min" <- w14
  "Ig min" <- w14
  "Ion vs time" <- w2
  "Ioff vs time" <- w2
  "Is on" <- w13
  "Id on" <- w13
  "Ig on" <- w13
  "Is off" <- w12
  "Id off" <- w12
  "Ig off" <- w12
  "I vs time (Bias Stress)" <- w2
  "Vp1" <- w3
  "Vp2" <- w3
  "Vp vs time (FPP Bias Stress)" <- w2
  "Vp vs Vg (FPP)" <- w2
  "Vdg vs time (Bias Stress)" <- w2
